vi "Position_TOTAL_R17.vi"() -> (0 "Valid Beacon Sets":bool[](array[boolean])=[TRUE, TRUE, TRUE, TRUE, FALSE], 5 "Distance Between \nCameras  (*unit)":sgl=1.6977187, 12 "dX, dY\nLeft Cam":cluster{"X":sgl[], "Y":sgl[]}={"X"=[-5.750775, -4.1849813, -3.081379, -2.0098581, 0.0], "Y"=[7.9585915, 7.9595685, 7.960258, 7.960927, 0.0]}, 13 "Position Valid":bool=TRUE, 14 "Left Camera Real Coordinates":cluster{"X":sgl, "Y":sgl}={"X"=7.9602513, "Y"=5.592073}, 16 "dX, dY\nRight Cam":cluster{"X":sgl[], "Y":sgl[]}={"X"=[-7.3032045, -5.737411, -4.6338086, -3.5622878, -1.5524296], "Y"=[7.2714148, 7.2723923, 7.2730813, 7.273751, -0.68717635]}, 17 "Distance to Each Beacon":cluster{" Right Cam":sgl[], " Left Cam":sgl[]}={" Right Cam"=[10.303839, 9.074741, 8.6335535, 8.091994, 1.0], " Left Cam"=[9.816596, 8.779684, 8.546625, 8.202919, 1.0]}, 18 "Robot Coordinates":cluster{"X":sgl, "Y":sgl}={"X"=7.616663, "Y"=6.3682876}, 19 "Orietnation\n(current)":sgl=-23.843685 format="%#_13g")   [LabVIEW 2015]
uses:
  <vilib>/Analysis/NI_AALPro.lvlib
  <vilib>/myRIO/Instrument Drivers/Onboard IO/DIO/DIO.lvlib
  <vilib>/Instr/_visa.llb/VISA Configure Serial Port (Instr).vi
  <vilib>/Analysis/coordinate.llb/2D Cartesian Coordinate Rotation (Array).vi
panel:
  out "IMAQ Scale":sgl=54.176815
  out "Current Recovery State -L":enum16{"Generic Sweep", "Recovery Search"}(ring)=enum."Recovery Search"
  out "Current Move Delta - L 2":u16
  out "Next Recovery State - Left":enum16{"Generic Sweep", "Recovery Search"}(ring)=enum."Recovery Search"
  out "Next Recovery State - Right":enum16{"Generic Sweep", "Recovery Search"}(ring)=enum."Recovery Search"
  out "Current Recovery State - Right":enum16{"Generic Sweep", "Recovery Search"}(ring)=enum."Recovery Search"
  in  "Initial Recovery State  - Right":enum16{"Generic Sweep", "Recovery Search"}(ring)=enum."Recovery Search"
  in  "Initial Recovery State - L":enum16{"Generic Sweep", "Recovery Search"}(ring)=enum."Recovery Search"
  out "Next Tracking State - Right":enum16{"Track", "Reactive Predict", ""}(ring)
  out "Current Tracking State - Right 2":enum16{"Track", "Reactive Predict", ""}(ring)
  in  "Initial Tracking State - Right":enum16{"Track", "Reactive Predict", ""}(ring)
  out "Last Track Angle - R":sgl=98.61328
  out "Next Tracking State - Left":enum16{"Track", "Reactive Predict", ""}(ring)
  in  "Initial Tracking State - Left":enum16{"Track", "Reactive Predict", ""}(ring)
  out "Current Tracking State - Left":enum16{"Track", "Reactive Predict", ""}(ring)
  in  "Timeout to \nEnable Reactive Predict":u16=5
  out "Tracking Timeout\nCount - R":i32
  in  "Tracking Timeout\nThreshold":i32=10
  out "Tracking Timeout\nCount - L":i32
  in  "Search Direction - in - Right":bool=TRUE
  out "Next Main State - Right":T1(ring)=enum."Tracking"
  in  "Recovery Search\nDirection - R":bool
  out "Recovery Mode Count in Right":i32
  out "Frames Processed\nCount - in Right":i32
  out "Recovery Search\nmove Count - Right":u16
  out "Recovery Search\nAttempt Count - Right":u16
  in  "Mounting Offset - Right":sgl=45.0
  in  "Tracking Angle - Right":sgl=98.60307
  in  "Current Servo Position\n- Right":u16
  out "New Data  Flag\nRight Servo":bool
  in  "Track Angle Valid  - R":bool=TRUE
  out "Current Main State - Right":T1(ring)=enum."Tracking"
  in  "Initial Main State- Right":T1(ring)
  in  "Recovery Search\nDirection - L 2":bool
  in  "Max Recovery Count\n(Recovery Search) 2":u16
  in  "Max Recovery\nSearch Attempts 2":u16
  in  "Image Lock - Right 2":bool
  out "Last Track Angle - L":sgl=87.24609
  in  "Recovery Search\nDirection - L":bool=TRUE
  out "Next Main State - Left":T1(ring)=enum."Tracking"
  out "Current Move Delta - L":u16
  in  "Max Recovery Count\n(Recovery Search)":u16=10
  in  "Max Recovery\nSearch Attempts":u16=3
  out "Recovery Search\nAttempt Count - in - L":u16
  out "Recovery Search\nmove Count - in - L":u16
  in  "Image Lock - Right":bool=TRUE
  out "Recovery Mode Count - in Left":u16
  in  "Middle Beacon\nCoordinates":cluster{"X":sgl, "Y":sgl}={"X"=0.0, "Y"=2.5}
  in  "Min Num Frames\nper Search":i32=2
  in  "Wait Tick Threshold":i32=10
  out "Frames Processed\nCount - in -L":i32
  in  "Maximum Move \nServo Threshold":i16=300
  in  "Minimum Delta \nServo Threshold":i16=3
  in  "Mounting Offset - Left":sgl=-45.0
  in  "Search Step Size":u16=50
  in  "Search Direction - in - L":bool
  in  "Current Servo Position\n- Left":u16
  in  "Tracking Angle - Left":sgl=87.25689
  out "New Data  Flag\nLeft Servo":bool
  in  "Track Angle Valid - Left":bool=TRUE
  in  "Image Lock - Left":bool=TRUE
  in  "Initial Main State - Left":T1(ring)
  out "Current Main State - Left":T1(ring)=enum."Tracking"
  in  "Position Calc\nTimer":u32=100 caption="Position Calc Timer"
  in  "Fetch Input\n(mSec)":u32=20 caption="Update Camera Input\n(mSec)"
  out "Right Data\nInput Flag\n- Internal":bool=TRUE
  in  "Position Calc\nReady":bool
  out "This Servo \nAngle - Right":sgl=98.90625
  in  "Beacon Angles -R":sgl[](array[numeric])=[111.28093, 105.355774, 98.60307, 92.04714, 103.90625]
  in  "Beacon Angles - L":sgl[](array[numeric])=[101.98467, 94.59042, 87.25689, 80.30646, 91.66016]
  in  "Valid Angles -R":bool[](array[boolean])=[TRUE, TRUE, TRUE, TRUE, FALSE]
  in  "Valid Angles - L":bool[](array[boolean])=[TRUE, TRUE, TRUE, TRUE, FALSE]
  out "Left Data\nInput Flag\n- Internal":bool
  in  "Check Shared Var Timer":u32=50 caption="Main Loop\n Timer (ms)"
  out "Left_Flag 2":bool
  out "Right_Flag 2":bool
  out "Beacons Found\n- Left (Bool Array) 2":bool[](array[boolean])=[TRUE, TRUE, TRUE, TRUE, FALSE]
  out "LEFT Beacon Coord - X px (IN) 2":sgl[](array[numeric])=[76.306, 116.841255, 157.35043, 195.67218, 0.0]
  out "LEFT Beacon Position - Y px (IN) 2":sgl[](array[numeric])=[154.30304, 148.59094, 148.39949, 146.94655, 0.0]
  out "This Servo \nAngle - Left":sgl=86.66016
  in  "Compliance Slope":u8=128
  out "deltaMoveServo\n- R":i16
  out "Move Respond - R":bool
  out "Move Respond - L":bool
  out "Last Position":cluster{"X":sgl, "Y":sgl}={"X"=7.6261, "Y"=6.350474}
  out "Last Orientation":sgl=-23.876373
  in  "Distance\nBetween Beacons \n- Tolerance":sgl=0.35 format="%#_13g"
  in  "Distance\nBetween Beacons":sgl=1.0 format="%#_13g"
  out "atan2(y,x)":sgl=0.35412386
  out "dT":dbl=143.499
  in  "Orientation (-2) \nWeight":sgl=0.083333336 format="%#_13g"
  in  "Orientation (-1) \nWeight":sgl=0.16666667 format="%#_13g"
  in  "New Orientation \nThreshold":sgl=10.0
  out "Position Valid\nHistory":bool[](array[boolean])=[TRUE, FALSE, FALSE, TRUE, TRUE, FALSE, TRUE, TRUE, TRUE, TRUE, TRUE, TRUE, FALSE, TRUE, FALSE]
  out "Orientation\nHistory":sgl[](array[numeric])=[-23.876373, 0.0, 0.0, -23.938759, -24.0458, 0.0, -23.14014, -22.504314, -22.596928, -22.90728, -23.237453, -23.75214, 0.0, -23.808718, 0.0]
  out "Robot Coordinates\nHistory":cluster{sgl, sgl}[](array[cluster])=[{7.6261, 6.350474}, {0.0, 0.0}, {0.0, 0.0}, {7.63815, 6.33973}, {7.6316156, 6.322055}, {0.0, 0.0}, {7.6863523, 6.2558875}, {7.688662, 6.2228284}, {7.6736236, 6.2455945}, {7.6880507, 6.2819676}, {7.6893277, 6.3140097}, {7.668109, 6.3330927}, {0.0, 0.0}, {7.6506357, 6.3142757}, {0.0, 0.0}]
  in  "New Position \nThreshold":sgl=0.2
  in  "position(-2) weight":sgl=0.2 format="%#_13g"
  in  "position(-1) weight":sgl=0.3 format="%#_13g"
  out "Orientation Avgd":sgl=-23.876373
  in  "History Size":u8=15
  in  "Max Y (arena)":sgl=15.0
  in  "Max X (arena)":sgl=35.0
  in  "New Position\nWeight":sgl=0.5 format="%#_13g"
  in  "New Orientation\nWeight":sgl=0.75 format="%#_13g"
  in  "Max Std Dev (3)":sgl=0.2 format="%#_13g"
  in  "Max Std Dev (4)":sgl=0.2 format="%#_13g"
  out "Post Filtering\n- Valid Beacons":bool[](array[boolean])=[FALSE, TRUE, TRUE, TRUE, FALSE]
  in  "New Pos\nThreshold (*unit)\nfilterd UNUSED":sgl=0.2
  out "Robot Coordinates - Avgd":cluster{"X":sgl, "Y":sgl}={"X"=7.6261, "Y"=6.350474}
  out "Real Position in Course 2":cluster{"X":dbl[], "Y":dbl[]}(graph)={"X"=[7.626100046018056], "Y"=[6.35047366782369]}
  out "Position \nLock Status":bool=TRUE
  out "Right Camera Real Coordinate":cluster{"X":sgl, "Y":sgl}={"X"=7.2730746, "Y"=7.1445026}
  out "deltaMoveServo\n- L":i16
  in  "Search Step Size\n(deg)":sgl=15.0 format="%#_13g"
  out "Beacons Found\n- Right (Bool Array)":bool[](array[boolean])=[TRUE, TRUE, TRUE, TRUE, FALSE]
  out "RIGHT Beacon Position - Y px (IN)":sgl[](array[numeric])=[153.02994, 149.48933, 150.4864, 150.33003, 0.0]
  out "RIGHT Beacon Coord - X px (IN)":sgl[](array[numeric])=[91.3685, 123.99656, 161.27843, 197.4523, 0.0]
  in  "Right Servo\nID":string="\u0001"
  in  "Servo Comm\nWait Time - (ms)":i32
  in  "Left Servo\nID":string="\u0000"
  out "dT - Comm Loop":u32=19
  in  "Servo Comm\nLoop Time (ms)":i32=20
  in  "close comms":bool
  in  "Max Read\nTx Attempts":u8=3
  in  "Max Write\nTx Attempts":u8=3
  out "Current R (10bit)":u16=696
  out "Servo Moving - R":bool
  out "Servo Moving - L":bool
  out "Current L (10bit)":u16=347
  in  "SERVO ENABLE":bool=TRUE
  out "Move Servo - L":bool
  out "Move Servo - R":bool
  in  "Servo Goal Position\n - Right":u16=695
  in  "Move Servo\nThreshold (deg)":sgl=2.0 format="%#_13g"
  in  "Servo Algorithm\nCycle Time(ms)":i32=25
  in  "Servo Goal Position\n - Left":u16=349
  in  "Current Angle\n - Left (internal)":sgl=86.66016
  in  "Current Angle\n - Right (internal)":sgl=98.90625
  in  "stop":bool
  in  "Num of Beacons (Total)":i8=5
  out "Angle to Pixel Ratios":T2={"Angle to Pixel\nRatio - Horizontal"=0.18125, "Angle to Pixel\nRatio - Vertical"=0.1875} {"Angle to Pixel\nRatio - Vertical" format="%#_13g"; "Angle to Pixel\nRatio - Horizontal" format="%#_13g"}
  in  "Cam AOV Vertical (deg)":sgl=45.0
  in  "Cam AOV Horizontal (deg)":sgl=58.0
  in  "Image Height (px)":sgl=240.0
  in  "Image Width (px)":sgl=320.0
  out "Beacon Coordinates - Left Image":T3={"Beacon Position - X px"=[76.306, 116.841255, 157.35043, 195.67218, 0.0], "Beacon Position - Y px"=[154.30304, 148.59094, 148.39949, 146.94655, 0.0]}
  out "Beacon Coordinates - Right Image":T3={"Beacon Position - X px"=[91.3685, 123.99656, 161.27843, 197.4523, 0.0], "Beacon Position - Y px"=[153.02994, 149.48933, 150.4864, 150.33003, 0.0]}
  out "Distance to LBF":sgl[](array[numeric])=[0.024284193, 0.015691843, 0.008273765, 0.028971607, 0.03291407]
  out "Local Coordinates - Calculated":cluster{sgl[], sgl[]}(graph)={[-2.0384164, -0.70265853, 0.4090246, 1.3811935, 0.0], [9.602626, 8.751521, 8.536832, 8.085801, 0.0]}
  out "Local Coordinates - Adjusted":cluster{sgl[], sgl[]}(graph)={[-2.0372734, -0.60508364, 0.4043527, 1.3844445, 0.0], [9.605212, 8.972328, 8.526259, 8.093158, 0.0]}
  out "Normalized Beacons\nCoordinates Relative\nto Robot\n- Local":cluster{"X":sgl[], "Y":sgl[]}={"X"=[-2.0372734, -0.60508364, 0.4043527, 1.3844445, 0.0], "Y"=[9.605212, 8.972328, 8.526259, 8.093158, 0.0]}
  out "Local Coordinates - Rotated":cluster{dbl[], dbl[]}(graph)={[1.5524295802029098, -5.750774735805926, -4.1849814062260675, -3.0813788557258652, -2.009858210562305, 0.0], [0.6871763361707266, 7.9585912385832795, 7.959568450875426, 7.960257859242679, 7.960927027680405, 0.0]}
  out "All Object Coordinates \n- Local - Rotated":cluster{"X":sgl[], "Y":sgl[]}={"X"=[1.5524296, -5.750775, -4.1849813, -3.081379, -2.0098581, 0.0], "Y"=[0.68717635, 7.9585915, 7.9595685, 7.960258, 7.960927, 0.0]}
  out "Local Coordinates - Normalized":cluster{sgl[], dbl[]}(graph)={[1.6977187, -2.0372734, -0.60508364, 0.4043527, 1.3844445, 0.0], [0.0, 9.605212211608887, 8.972328186035156, 8.526259422302246, 8.093157768249512, 0.0]}
  in  "Max Std Dev (5)":sgl=0.2 format="%#_13g"
  out "All Object Coordinates \n- Local":cluster{"X":sgl[], "Y":sgl[]}={"X"=[1.6977187, -2.0372734, -0.60508364, 0.4043527, 1.3844445, 0.0], "Y"=[0.0, 9.605212, 8.972328, 8.526259, 8.093158, 0.0]}
  out "LOCAL\nBeacon Coordinates\nRelative to Robot":cluster{"dX_beacon":sgl[], "dY_beacon":sgl[]}={"dX_beacon"=[-2.0384164, -0.70265853, 0.4090246, 1.3811935, 0.0], "dY_beacon"=[9.602626, 8.751521, 8.536832, 8.085801, 0.0]}
  out "dA2":sgl=9.6935425 format="%#_13g"
  out "All Same\nDirection":bool=TRUE
  out "Valid Data\nSets":bool[](array[boolean])=[TRUE, TRUE, TRUE, TRUE, FALSE]
  in  "Distance Threshold\nRef Triangles (*unit)":sgl=30.0
  in  "Real Beacon\n - Coordinates":cluster{"X":dbl[], "Y":dbl[]}={"X"=[0.0, 0.0, 0.0, 0.0, 0.0, 0.0], "Y"=[0.5, 1.5, 2.5, 3.5, 4.5, 0.0]}
  # "POSITION CALCULATION VARIABLES"
  # "OUTPUT VALUES"
  # "CONFIG VALUES"
  # "FILTER CONFIG VALUES"
  # "FEEDBACK INPUT VALUES"
  # "INPUT VALUES"
  # "INTERMEDIATE VALUES"
  # "IMAGE TO ANGLE VARIABLES"
  # "VISION PROCESSEING INPUTS"
  # "Use moving average for previous orientation thresholds"
  # "INPUTS"
  # "CONFIG"
  # "OUTPUT VALUES"
  # "*********************"
  # "unfiltered"
  # "NEW FILTER VALS"
  # "Inter Beacon Distance Filtering"
  # "**Calibrate \"distance between cameras\" to image scale"
  # "SERVO CONTROL VARIABLES"
  # "SERVO CONTROL VARIABLES"
  # "CONFIG"
  # "SHARED VARIABLE INPUTS"
  # "LOCAL VARIABLE INPUTS"
  # "INTERNRAL VARIABLES"
  # "SEARCH ROUTINE VARIABLES"
  # "MISC"
  # "SERVO IDs"
  # "CONTROL DELAYS"
  # "COMM LOOP DELAY"
  # "COMM PROTOCOL"
  # "SETTINGS"
  # "Make function of distance^^"
  # "**** only left side starts search\nat previously known good angle"
  # "LEFT SERVO"
  # "RIGHT SERVO"
  # "Main State Machine"
  # "Recovery State Machine"
  # "Current Track Angle Inputs"
  # "Servo Status Inputs"
  # "Main State Machine Inputs"
  # "Recovery State Machine Inputs"
  # "Current Track Angle Inputs"
  # "Servo Status Inputs"
  # "Recovery State Machine Feedback"
  # "Tracking State Machine Inputs"
  # "Tracking State Machine Inputs"
  # "NOTE: Must be 1 bigger than amount of beacons"
  # "NOTE: Must be 1 bigger than amount of beacons"
types:
  T1 = enum16{"Start Up Search", "Tracking", "Recovery Mode", ""}
  T2 = cluster{"Angle to Pixel\nRatio - Horizontal":sgl, "Angle to Pixel\nRatio - Vertical":sgl}
  T3 = cluster{"Beacon Position - X px":sgl[], "Beacon Position - Y px":sgl[]}
  T4 = cluster{"Array of Double":dbl[], "Array of Double":dbl[]}
  T5 = typedef "DIO.lvlib/DIO Reference.ctl" = cluster{"myRIO Reference":T6, "DIO Channels List":T10}
  T6 = typedef "myRIO Generic Hardware Reference.ctl" = cluster{"myRIO Model":T7, "myRIO Hardware Reference":T8}
  T7 = typedef "Hardware Version Enum.ctl" = enum16{"Unknown", "myRIO-1900", "myRIO-1950", "roboRIO"}
  T8 = typedef "myRIO v1.0 Reference.ctl" = cluster{"Generic FPGA Reference":T9, "Allow multiple opens":bool}
  T9 = typedef "Generic FPGA Reference.ctl" = refnum<k20>
  T10 = typedef "DIO Channels List.ctl" = T11[]
  T11 = typedef "DIO Channels Enum.ctl" = enum16{"Not Connected", "C/DIO0", "C/DIO1", "C/DIO2", "C/DIO3", "C/DIO4", "C/DIO5", "C/DIO6", "C/DIO7", "A/DIO0", "A/DIO1", "A/DIO2", "A/DIO3", "A/DIO4", "A/DIO5", "A/DIO6", "A/DIO7", "A/DIO8", "A/DIO9", "A/DIO10", "A/DIO11", "A/DIO12", "A/DIO13", "A/DIO14", "A/DIO15", "B/DIO0", "B/DIO1", "B/DIO2", "B/DIO3", "B/DIO4", "B/DIO5", "B/DIO6", "B/DIO7", "B/DIO8", "B/DIO9", "B/DIO10", "B/DIO11", "B/DIO12", "B/DIO13", "B/DIO14", "B/DIO15", "LED0", "LED1", "LED2", "LED3", "Button0", "DIO/DIO0", "DIO/DIO1", "DIO/DIO2", "DIO/DIO3", "DIO/DIO4", "DIO/DIO5", "DIO/DIO6", "DIO/DIO7", "DIO/DIO8", "DIO/DIO9", "SPI/CS0", "SPI/CS1", "SPI/CS2", "SPI/CS3", "LED RADIO (Green)", "LED RADIO (Red)", "LED COMM (Green)", "LED COMM (Red)", "LED MODE (Green)", "LED MODE (Red)"}
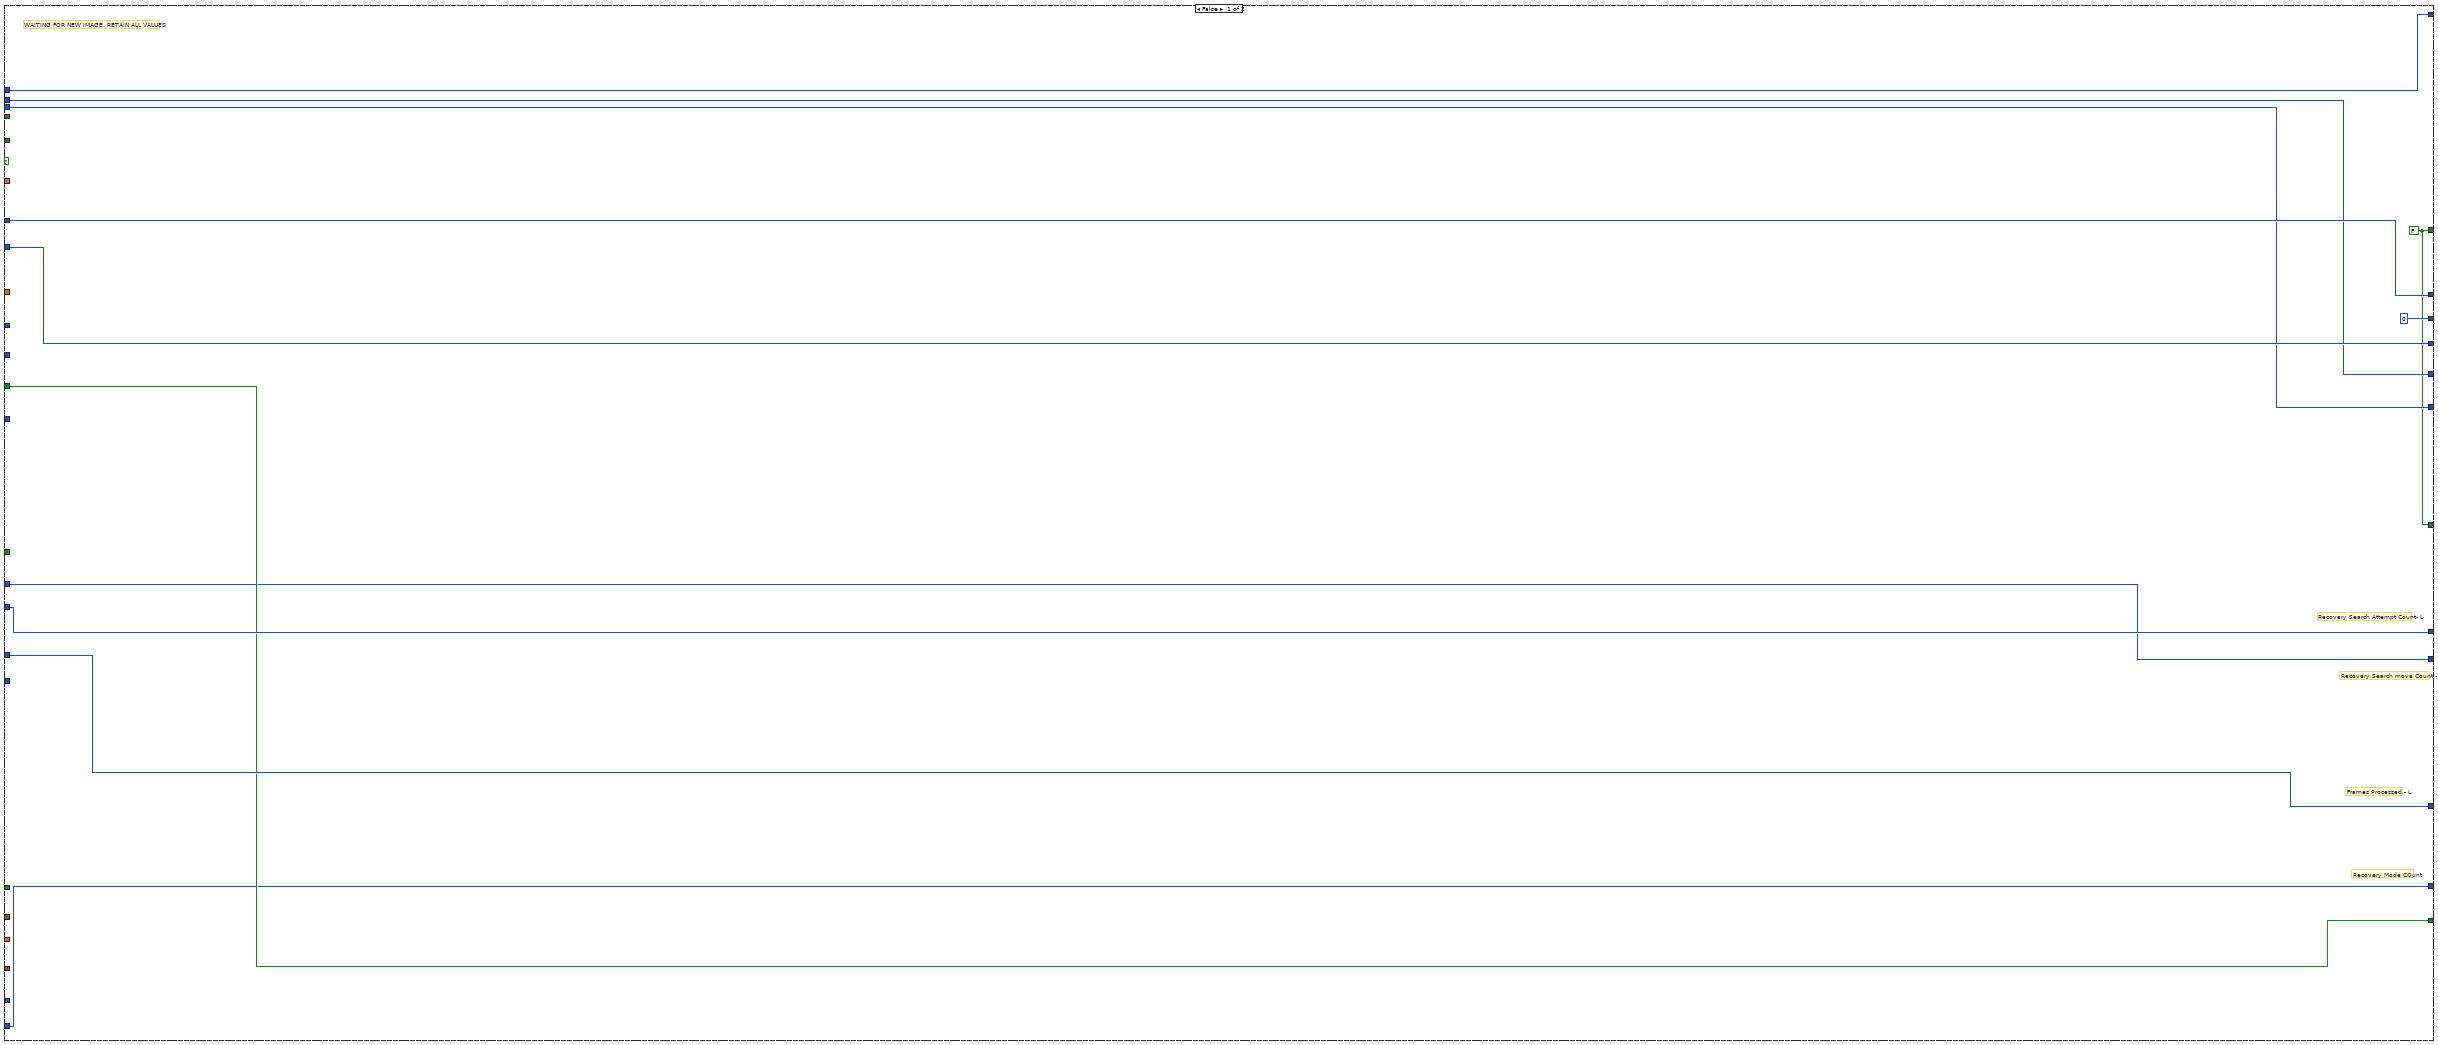
[diagram p2: hidden frame]
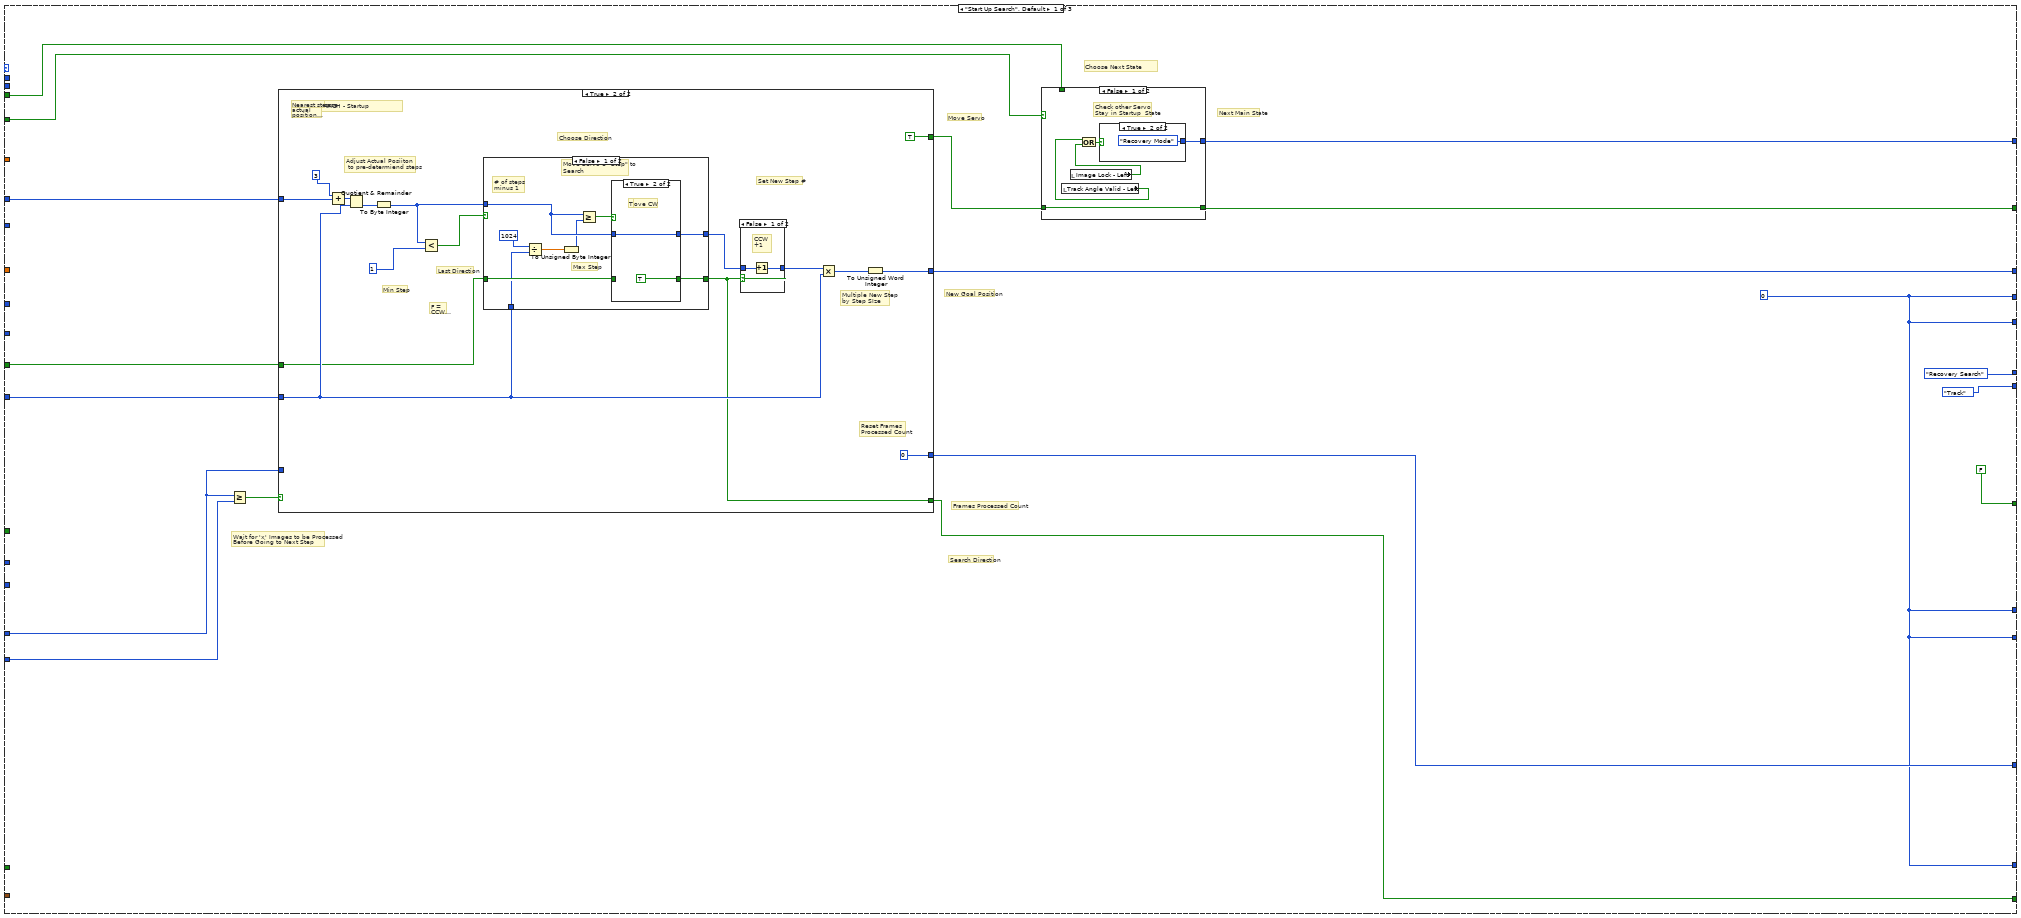
[diagram p3: hidden frame]
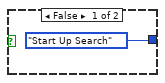
[diagram p4: hidden frame]
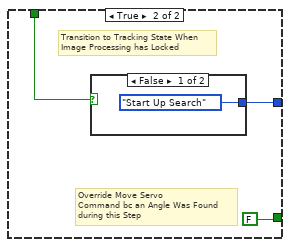
[diagram p5: hidden frame]
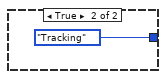
[diagram p6: hidden frame]
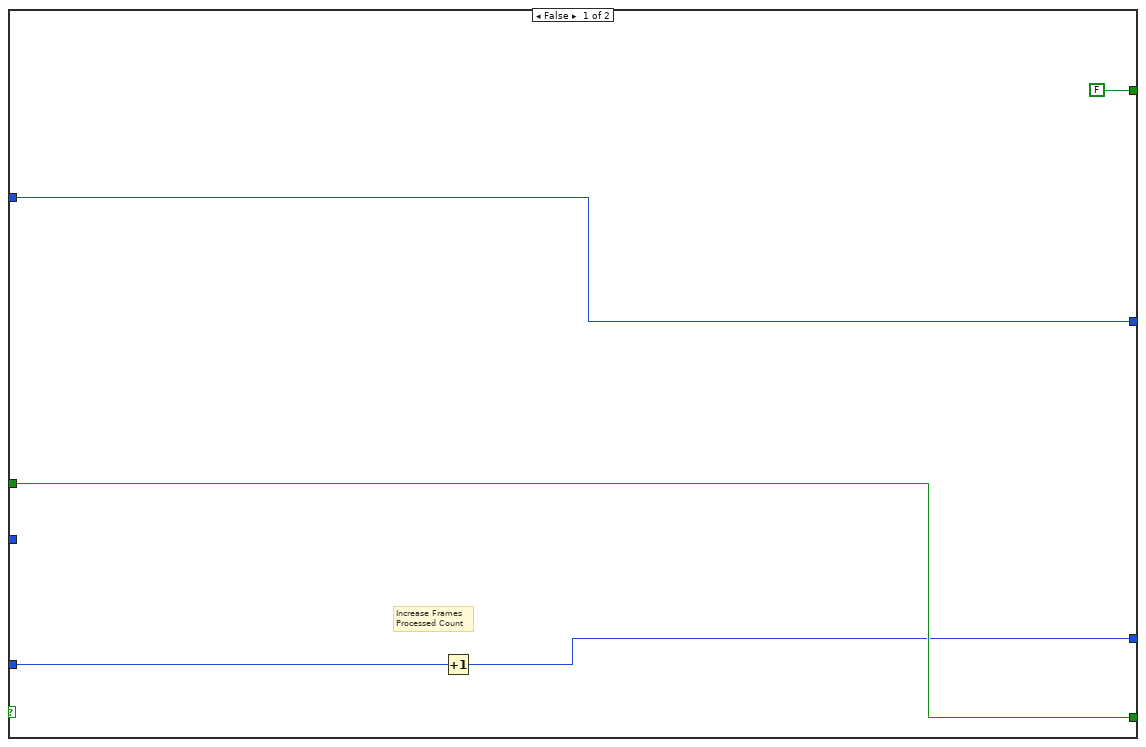
[diagram p7: hidden frame]
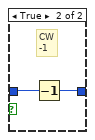
[diagram p8: hidden frame]
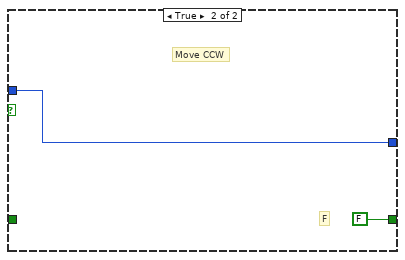
[diagram p10: hidden frame]
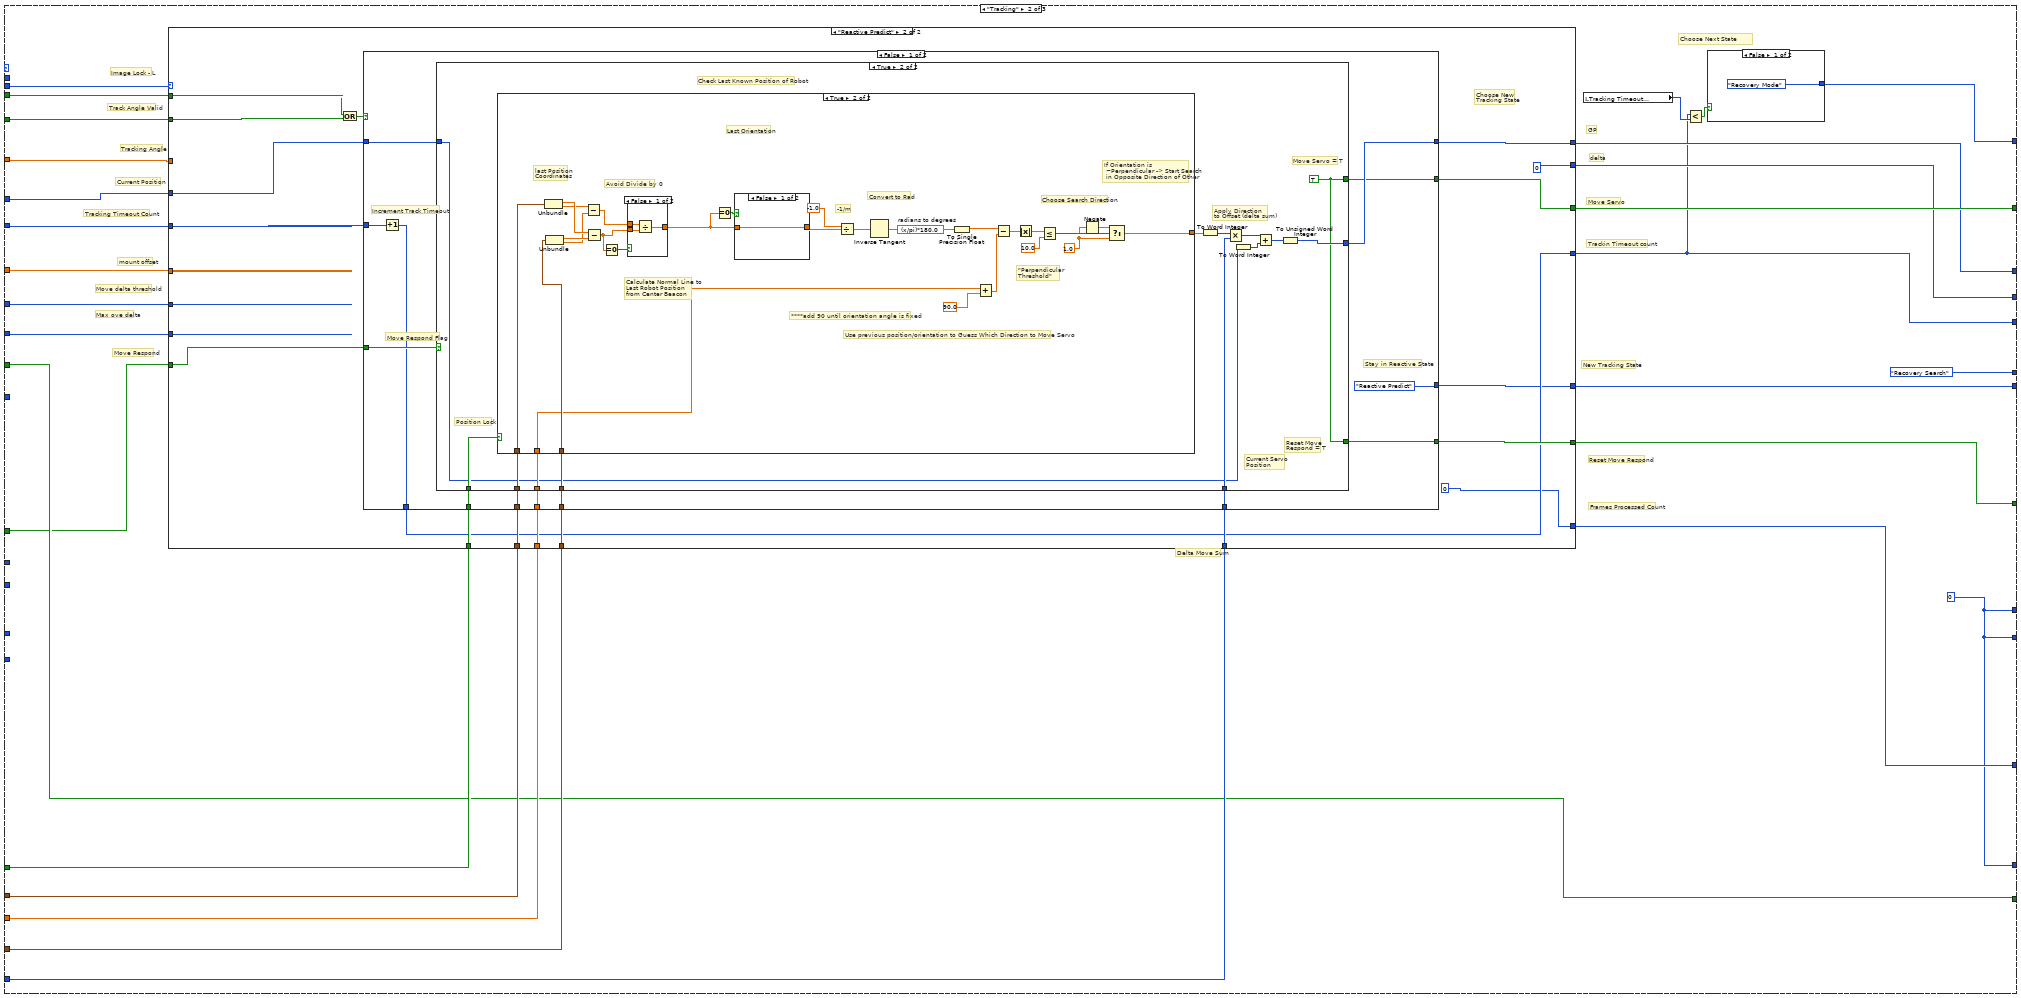
[diagram p11: hidden frame]
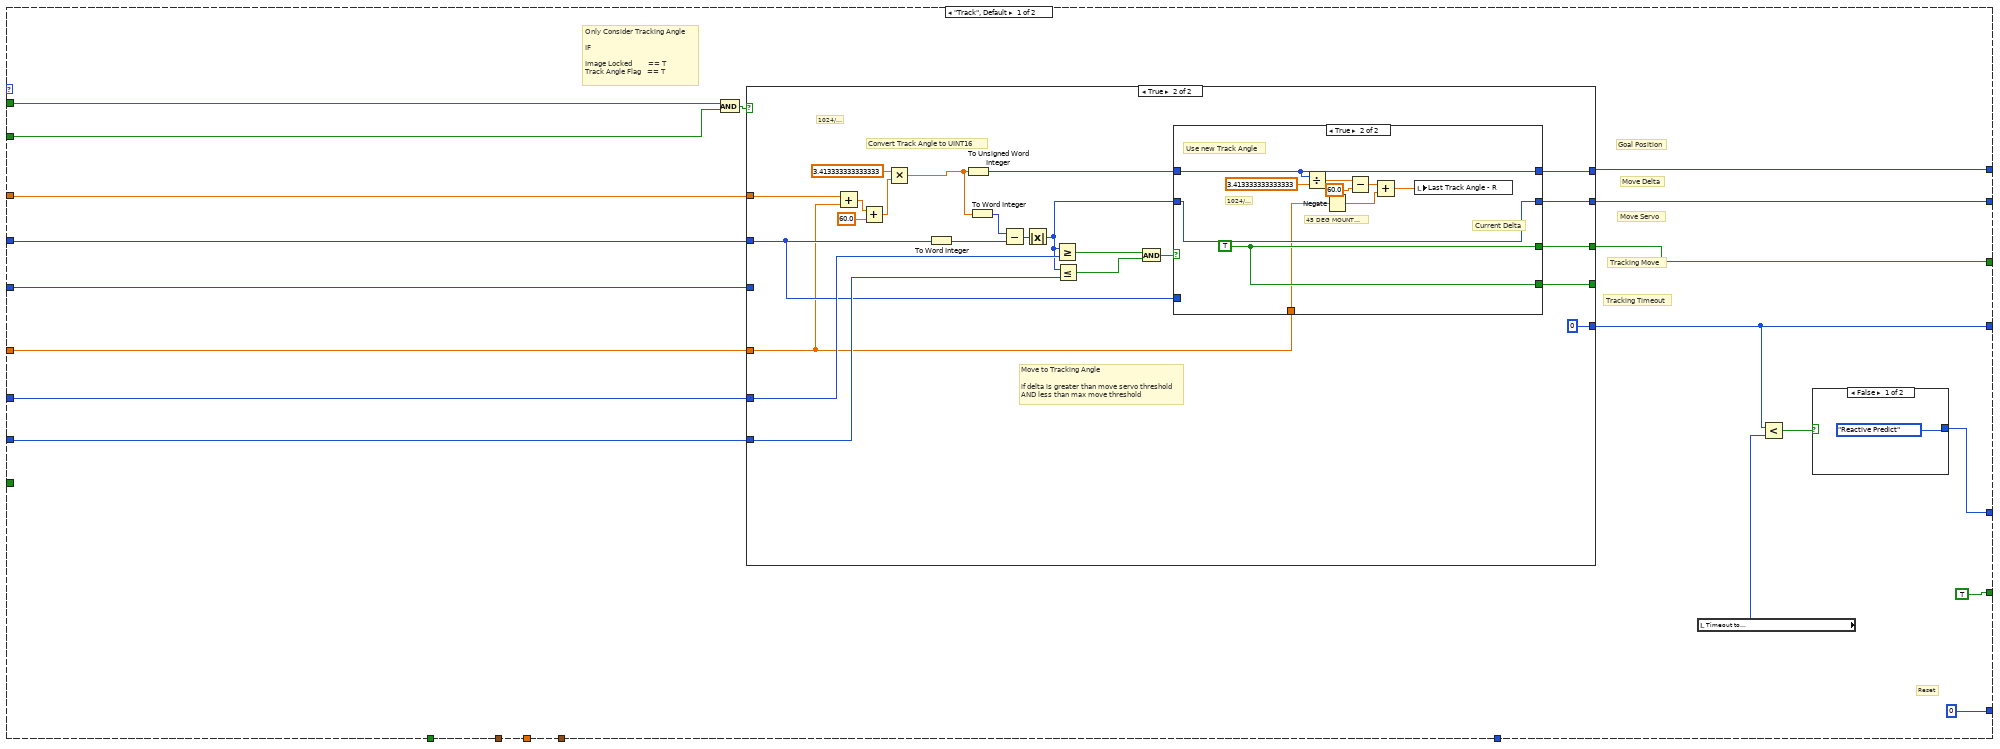
[diagram p12: hidden frame]
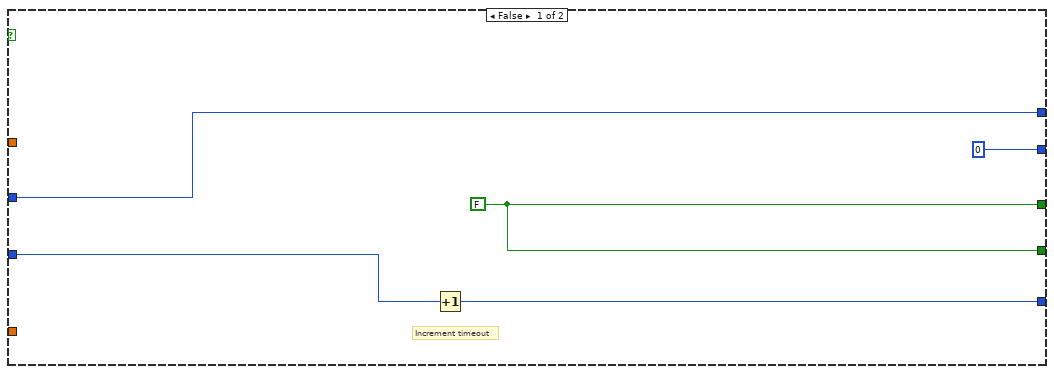
[diagram p13: hidden frame]
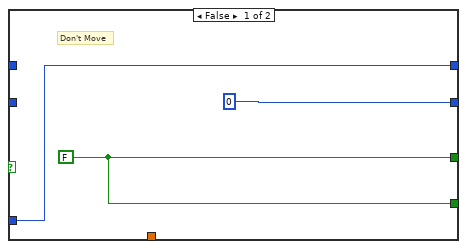
[diagram p14: hidden frame]
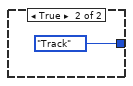
[diagram p15: hidden frame]
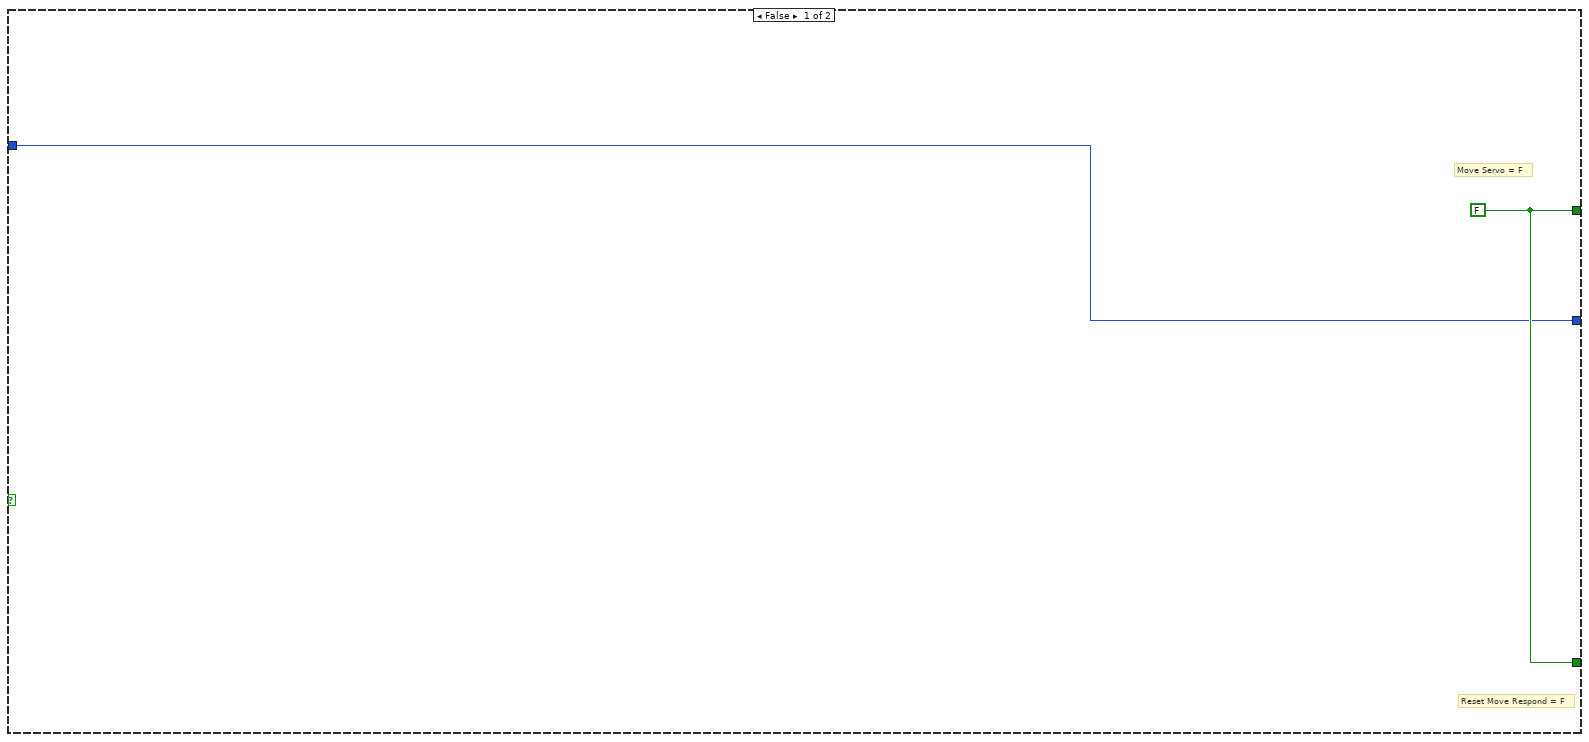
[diagram p16: hidden frame]
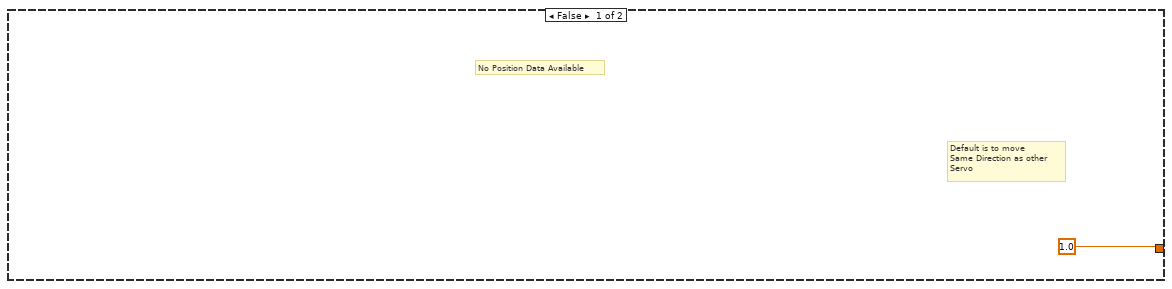
[diagram p17: hidden frame]
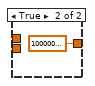
[diagram p18: hidden frame]
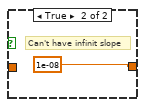
[diagram p19: hidden frame]
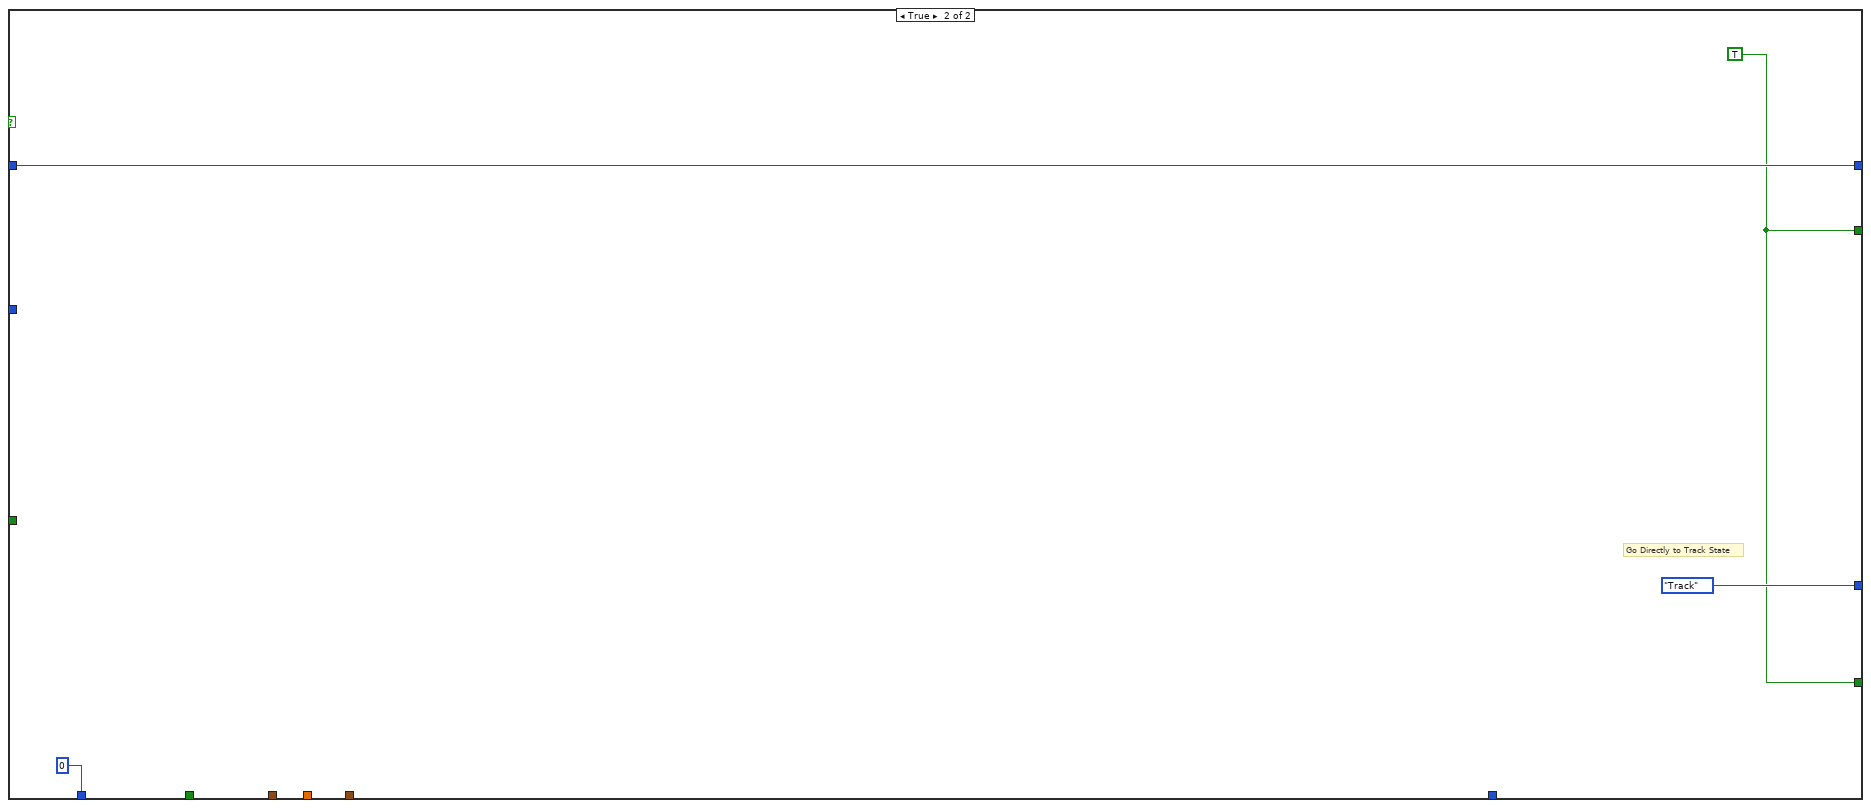
[diagram p20: hidden frame]
diagram:
  (unwired) enum16{"Generic Sweep", "Recovery Search"}."Recovery Search"
  w11 = 0 ("Frames Processed\nCount - in")
  w12 = 0 ("Frames Processed\nCount - in")
  w1 = FALSE
  w34 = sgl 0.0
  # "SERVO CONTROL FLAGS"
  # "***"
  # "Next Tracking State"
  # "Tracking Timeout Count"
  # "Search Direction - L"
  # "Next Recovery State"
  # "Move Respond"
  # "Recovery Mode Count - L"
  # "Delta Move Sum - L"
  # "Wait Tick Count - L"
  # "Frames Processed - L"
  # "Recovery Search move Count - L"
  # "Recovery Search Attempt Count- L"
  # "Next Main State"
  # "Search Direction - L"
  # "Next Recovery State"
  # "INPUTS - Local vars"
  # "Recovery Mode Count - L"
  # "Delta Move Sum - L"
  # "Frames Processed\nLeft"
  # "Move Respond - R"
  # "Initial Search Direction\n- Right"
  # "Move Respond"
  # "Recovery Mode Count - L"
  # "Delta Move Sum - L"
  # "Wait Tick Count - L"
  # "Frames Processed - L"
  # "Recovery Search move Count - L"
  # "Recovery Search Attempt Count- L"
  # "Next Main State"
  # "Settings -- Update in a slow loop"
  # "Recovery Mode Count - L"
  # "Delta Move Sum - L"
  # "Frames Processed\nLeft"
  # "Move Respond - L"
  # "Replace these with\nconstants"
  # "Initial Search Direction\n- Left"
  # "Read Inputs when Available"
  # "# of Physical Beacons"
  # "Right Data Internal Falg"
  # "Left Data Internal Falg"
  # "Initialize Shift Arrays"
  # "Robot Position (cluster)\nShift Array"
  # "Robot Position (cluster)\nShift Array"
  # "Position Valid Shift Array"
  # "Orientation Shift Array"
  # "Position Valid Shift Array"
  # "Orientation Shift Array"
  # "Servo Communication (to Servo- UART))"
  # "Internal Local Variables"
  # "Servo Control Logic"
  # "Local Variables"
  # "Images to Robot Position Calculation Process"
  # "SERVO MOTOR CONTROL"
  # "SERVO MOTOR CONTROL"
  n1 = Divide(x="Cam AOV Horizontal (deg)", y="Image Width (px)") -> (x/y=w25:sgl)
  n2 = Divide(x="Cam AOV Vertical (deg)", y="Image Height (px)") -> (x/y=w26:sgl)
  n3 = Bundle(w25, w26) -> (w20:cluster{sgl, sgl})  [unwired: 1 in]
  "Angle to Pixel Ratios" <- w20
  n4 = disable-structure shown="Disabled" {
    frame Disabled {
      # "Always Read Incoming Flags & Store"
      n5 = while {
        tunnel: "Check Shared Var Timer" -> [w46]
        stop <- FALSE stop-if-true
        n6 = shared-variable "myRIO-1900\\Lib1.lvlib\\RIGHT_FLAG"() -> (→"Right_Flag 2":bool)  [unwired: 1 in, 1 out]
        n7 = shared-variable "myRIO-1900\\Lib1.lvlib\\Left_Flag"() -> (→"Left_Flag 2":bool)  [unwired: 1 in, 1 out]
        n8 = call "Wait8"("Count(mSec)"=w46) -> ()  [unwired: 1 out]
      }
    }
    frame Enabled {
    }
  }
  n9 = while {
    shift-right: [w55] -> _
    shift-left: w1 -> [w60]
    shift-right: [w54] -> _
    shift-left: w1 -> [w58]
    tunnel: w20 -> [w56]
    tunnel: "Num of Beacons (Total)" -> [w57]
    stop <- FALSE stop-if-true
    # "Wait for Both Internal Flags"
    n10 = call "Wait6"("Count(mSec)"="Fetch Input\n(mSec)") -> ()  [unwired: 1 out]
    n11 = shared-variable "RT myRIO Target - Overlord\\Localization_Variables_r0.lvlib\\RIGHT_FLAG"() -> (w51:bool)  [unwired: 1 in, 1 out]
    n12 = shared-variable "RT myRIO Target - Overlord\\Localization_Variables_r0.lvlib\\Left_Flag"() -> (w52:bool)  [unwired: 1 in, 1 out]
    n13 = case shown="True" w51 {
      tunnel: w57 -> [_ w75]
      tunnel: w56 -> [_ w73]
      tunnel: [w61 w62] -> w49
      tunnel: w58 -> [w61 _]
      frame False {
        # "Don't Update Servo Position\nbc we're waiting on new Data to\ncome in and the servo position\nwas set at the previous set of data"
      }
      frame True {
        w62 = TRUE
        # "Store Values"
        # "Raise Internal Flag"
        # "If New Data Available"
        # "From Shift Reg"
        # "Perforrm Indivudual Angle Calculation"
        # "Pull Down Individual Flag"
        n14 = shared-variable "RT myRIO Target - Overlord\\Localization_Variables_r0.lvlib\\RIGHT_BEACON_X_array"() -> (w68:dbl[])  [unwired: 1 in, 1 out]
        "RIGHT Beacon Coord - X px (IN)" <- w68
        n15 = shared-variable "RT myRIO Target - Overlord\\Localization_Variables_r0.lvlib\\Image Lock - R"() -> (w63:bool)  [unwired: 1 in, 1 out]
        n16 = shared-variable "RT myRIO Target - Overlord\\Localization_Variables_r0.lvlib\\RIGHT_BEACON_Y_array"() -> (w67:dbl[])  [unwired: 1 in, 1 out]
        "RIGHT Beacon Position - Y px (IN)" <- w67
        n17 = shared-variable "RT myRIO Target - Overlord\\Localization_Variables_r0.lvlib\\RIGHT_BEACON_BOOL_array"() -> (w66:bool[])  [unwired: 1 in, 1 out]
        "Beacons Found\n- Right (Bool Array)" <- w66
        n18 = local write "Image Lock - Right"(w63) -> ()
        n19 = Bundle("Array of Double"=w68, "Array of Double"=w67) -> (w65:T4)  [unwired: 1 in]
        "Beacon Coordinates - Right Image" <- w65
        n20 = shared-variable "RT myRIO Target - Overlord\\Localization_Variables_r0.lvlib\\Right Servo Angle_Image"() -> (w64:dbl)  [unwired: 1 in, 1 out]
        "This Servo \nAngle - Right" <- w64
        n21 = shared-variable "RT myRIO Target - Overlord\\Localization_Variables_r0.lvlib\\RIGHT_FLAG"(FALSE) -> ()  [unwired: 1 in, 1 out]
        n22 = feedback #1() -> (w77:sgl[])  [unwired: 1 in]
        n23 = feedback #2() -> (w76:bool[])  [unwired: 1 in]
        n24 = call "Angle Calc_Individual Process R2.vi"("Angle to Pixel Ratios"=w73, "Previous Angles"=w77, "Num of Beacons"=w75, "Beacon Coordinates - Image"=w65, "Current Servo Angle"=w64, "Beacons Found (Bool Array)"=w66, "Previous Valid Angles"=w76) -> ("Servo Goal Angle"=w72:dbl, "Valid Beacons (Bool Array)\nPosition Calc"=w70:bool[], "Angle Of Beacons \nRelative to Robot"=w69:sgl[], "Angles Valid\nServo Control"=w71:bool)  [unwired: 2 in, 3 out]
        n25 = feedback-in #1(w69) -> ()
        n26 = feedback-in #2(w70) -> ()
        n27 = local write "Track Angle Valid  - R"(w71) -> ()
        n28 = local write "Beacon Angles -R"(w69) -> ()
        n29 = local write "Valid Angles -R"(w70) -> ()
        n30 = local write "Tracking Angle - Right"(w72) -> ()
        n31 = local write "New Data  Flag\nRight Servo"(w62) -> ()
      }
    }
    "Right Data\nInput Flag\n- Internal" <- w49
    n32 = case shown="False" w52 {
      tunnel: [w78 w79] -> w48
      tunnel: w60 -> [w78 _]
      tunnel: w56 -> [_ w83]
      tunnel: w57 -> [_ w82]
      frame False {
        # "Don't Update Servo Position\nbc we're waiting on new Data to\ncome in and the servo position\nwas set at the previous set of data"
      }
      frame True {
        w79 = TRUE
        # "Store Values"
        # "Raise Internal Flag"
        # "If New Data Available"
        # "Perforrm Indivudual Angle Calculation"
        # "Pull Down Individual Flag"
        n33 = shared-variable "RT myRIO Target - Overlord\\Localization_Variables_r0.lvlib\\LEFT_BEACON_X_array"() -> (w90:dbl[])  [unwired: 1 in, 1 out]
        "LEFT Beacon Coord - X px (IN) 2" <- w90
        n34 = shared-variable "RT myRIO Target - Overlord\\Localization_Variables_r0.lvlib\\LEFT_BEACON_Y_array"() -> (w91:dbl[])  [unwired: 1 in, 1 out]
        "LEFT Beacon Position - Y px (IN) 2" <- w91
        n35 = shared-variable "RT myRIO Target - Overlord\\Localization_Variables_r0.lvlib\\LEFT_BEACON_BOOL_array"() -> (w92:bool[])  [unwired: 1 in, 1 out]
        "Beacons Found\n- Left (Bool Array) 2" <- w92
        n36 = shared-variable "RT myRIO Target - Overlord\\Localization_Variables_r0.lvlib\\Image Lock - L"() -> (w80:bool)  [unwired: 1 in, 1 out]
        n37 = local write "Image Lock - Left"(w80) -> ()
        n38 = Bundle("Array of Double"=w90, "Array of Double"=w91) -> (w88:T4)  [unwired: 1 in]
        "Beacon Coordinates - Left Image" <- w88
        n39 = shared-variable "RT myRIO Target - Overlord\\Localization_Variables_r0.lvlib\\Left Servo Angle_Image"() -> (w81:dbl)  [unwired: 1 in, 1 out]
        "This Servo \nAngle - Left" <- w81
        n40 = shared-variable "RT myRIO Target - Overlord\\Localization_Variables_r0.lvlib\\Left_Flag"(FALSE) -> ()  [unwired: 1 in, 1 out]
        n41 = feedback #3() -> (w94:sgl[])  [unwired: 1 in]
        n42 = feedback #4() -> (w93:bool[])  [unwired: 1 in]
        n43 = call "Angle Calc_Individual Process R2.vi"("Angle to Pixel Ratios"=w83, "Previous Angles"=w94, "Num of Beacons"=w82, "Beacon Coordinates - Image"=w88, "Current Servo Angle"=w81, "Beacons Found (Bool Array)"=w92, "Previous Valid Angles"=w93) -> ("Servo Goal Angle"=w87:dbl, "Valid Beacons (Bool Array)\nPosition Calc"=w85:bool[], "Angle Of Beacons \nRelative to Robot"=w84:sgl[], "Angles Valid\nServo Control"=w86:bool)  [unwired: 2 in, 3 out]
        n44 = feedback-in #3(w84) -> ()
        n45 = feedback-in #4(w85) -> ()
        n46 = local write "Track Angle Valid - Left"(w86) -> ()
        n47 = local write "Beacon Angles - L"(w84) -> ()
        n48 = local write "Valid Angles - L"(w85) -> ()
        n49 = local write "Tracking Angle - Left"(w87) -> ()
        n50 = local write "New Data  Flag\nLeft Servo"(w79) -> ()
      }
    }
    "Left Data\nInput Flag\n- Internal" <- w48
    n51 = And(x=w48, y=w49) -> (x .and. y?=w59:bool)
    n52 = case shown="True" w59 {
      selector: w59 -> [_ w97]
      tunnel: w48 -> [w96 _]
      tunnel: [w96 w98] -> w55
      tunnel: [w95 w98] -> w54
      tunnel: w49 -> [w95 _]
      frame False {
      }
      frame True {
        w98 = FALSE
        # "Reset Internal Data Flags"
        # "Position Data\nReady Enabled"
        n53 = local write "Position Calc\nReady"(w97) -> ()
      }
    }
  }
  n54 = Bundle(w34, w34) -> (w37:cluster{sgl, sgl})  [unwired: 1 in]
  n55 = Initialize Array(w34, "History Size") -> (w32:sgl[])
  n56 = Initialize Array(w37, "History Size") -> (w33:cluster{sgl, sgl}[])
  n57 = Initialize Array(FALSE, "History Size") -> (w31:bool[])
  n58 = call "Tick Count4"() -> ("Tick Count(uSec)"=w30:u32)
  n59 = while {
    shift-right: [w109] -> _
    shift-left: w32 -> [w106]
    shift-right: [w108] -> _
    shift-left: w31 -> [w107]
    shift-right: [w110] -> _
    shift-left: w33 -> [w101]
    shift-right: [w102] -> _
    shift-left: w30 -> [w103]
    stop <- "stop" stop-if-true
    n60 = call "Wait5"("Count(mSec)"="Position Calc\nTimer") -> ()  [unwired: 1 out]
    n61 = case shown="True" "Position Calc\nReady" {
      selector: "Position Calc\nReady" -> [_ w124]
      tunnel: w101 -> [_ w159]
      tunnel: w101 -> [w119 w149]
      tunnel: w106 -> [w121 w148]
      tunnel: w107 -> [w120 w147]
      tunnel: [w121 w146] -> w109
      tunnel: [w120 w141] -> w108
      tunnel: [w119 w145] -> w110
      tunnel: w107 -> [_ w144]
      tunnel: w106 -> [_ w143]
      tunnel: [w118 w136] -> w104
      tunnel: w103 -> [_ w136]
      tunnel: [FALSE TRUE] -> w105
      tunnel: w101 -> [_ w131]
      frame False {
        n62 = call "Tick Count5"() -> ("Tick Count(uSec)"=w118:u32)
      }
      frame True {
        # "Update Outputs\nif Current Calc is Invalid\n(shouldn't matter)"
        # "Estimate Orienation Based on Previous Position"
        # "****# of previous in history that must be true\nin order for position to be considered \"locked\""
        # "New Position is Valid if both \nOrientation and Positions\nis within range of previous"
        # "Robot Position\n Shift Array"
        # "Position Valid Shift Array"
        # "Orientation Shift Array"
        # "Orientation Value"
        # "Shift & Insert Current Position Valid"
        # "Position Valid\n(orientation)"
        # "Position Valid\n(position)"
        # "Update Shift Registers"
        # "Shift & Insert Current Calculated Orientation"
        # "Shift & Insert Current Robot Position"
        # "UPDATE FINAL OUTPUT\n VALUES"
        # "Find Common Beacons\nAmong Cameras"
        # "Valid Beacon Sets"
        # "Currently will only\ncalculate position if 2+ \nbeacons are available \nfrom both cameras"
        n63 = Not(x=w124) -> (.not. x?=w125:bool)
        n64 = local write "Position Calc\nReady"(w125) -> ()
        n65 = disable-structure shown="Disabled" {
          disable-tunnel: "Valid Angles - L" -> [w225 _]
          disable-tunnel: "Valid Angles -R" -> [w224 _]
          frame Disabled {
            # "Each has at \nleast 1 beacon"
            n66 = Boolean Array To Number(Boolean array=w224) -> (number=w226:u32)
            n67 = Boolean Array To Number(Boolean array=w225) -> (number=w227:u32)
            n68 = Greater Than 0?(x=w226) -> (x > 0?=w228:bool)
            n69 = Greater Than 0?(x=w227) -> (x > 0?=w229:bool)
            n70 = And(x=w229, y=w228) -> ()  [unwired: 1 out]
          }
          frame Enabled {
          }
        }
        n71 = And(x="Valid Angles - L", y="Valid Angles -R") -> (x .and. y?=w160:bool[])
        "Valid Beacon Sets" <- w160
        n72 = local read "Num of Beacons (Total)"() -> (w126:i8)
        n73 = Boolean To (0,1)(Boolean=w160) -> (0, 1=w164:i16[])
        n74 = Add Array Elements(numeric array=w164) -> (sum=w163:i16)
        n75 = Greater?(x=w163, y=1) -> (0:w161:bool)
        n76 = case shown="True" w161 {
          tunnel: w160 -> [_ w252]
          tunnel: "Beacon Angles - L" -> [_ w250]
          tunnel: "Beacon Angles -R" -> [_ w249]
          tunnel: w126 -> [_ w251]
          tunnel: w160 -> [_ w248]
          tunnel: w159 -> [_ w247]
          tunnel: [w231 w246] -> w151
          tunnel: [w232 w245] -> w134
          tunnel: [w232 w244] -> w133
          tunnel: [w230 w243] -> w152
          tunnel: w144 -> [_ w242]
          tunnel: w143 -> [_ w241]
          tunnel: w131 -> [_ w240]
          frame False {
            w230 = sgl 0.0 ("f")
            w232 = FALSE
            # "FALSE"
            # "F"
            n77 = Bundle("f"=w230, "f"=w230) -> (w231:cluster{"f":sgl, "f":sgl})  [unwired: 1 in]
          }
          frame True {
            # "Number of Beacons"
            # "**maybe add case\nto handle if some arent\nsame direction"
            # "Check 1st element\nwith rest of elements"
            # "Find delta X and delta Y\nto Each Camera from Each Beacon"
            # "Make Sure all Pointed \nIn Same Direction"
            # "For Each Valid Beacon\nCalculate Distance from Each Camera to Each Beacon"
            n78 = shared-variable "RT myRIO Target - Overlord\\Localization_Variables_r0.lvlib\\Scale - Right"() -> (w236:sgl)  [unwired: 1 in, 1 out]
            n79 = shared-variable "RT myRIO Target - Overlord\\Localization_Variables_r0.lvlib\\Scale - Left"() -> (w237:sgl)  [unwired: 1 in, 1 out]
            n80 = Add(x=w237, y=w236) -> (x+y=w235:sgl)
            n81 = Divide(x=w235, y=sgl 2.0) -> (x/y=w233:sgl)
            "IMAQ Scale" <- w233
            n82 = call "Scaling and Mapping"("Signals"=w233) -> ("Scaled Signals"=w239:dynamicdata)  [unwired: 9 in, 1 out]
            n83 = To Single Precision Float(number=w239) -> (single precision float=w238:sgl)
            "Distance Between \nCameras  (*unit)" <- w238
            n84 = for {
              N: w251 -> [_]
              tunnel: w252 -> [w726] mode=indexing
              tunnel: w250 -> [w725] mode=indexing
              tunnel: w249 -> [w724] mode=indexing
              tunnel: w238 -> [w723]
              tunnel: "Distance Threshold\nRef Triangles (*unit)" -> [w722]
              tunnel: [w721] -> w257 mode=indexing
              tunnel: [w720] -> _ mode=indexing
              tunnel: [w719] -> w258 mode=indexing
              tunnel: [w718] -> w254 mode=indexing
              tunnel: [w717] -> w253 mode=indexing
              tunnel: [w716] -> w259 mode=indexing
              n85 = case shown="True" w726 {
                tunnel: w725 -> [w731 w741]
                tunnel: w724 -> [w730 w740]
                tunnel: w723 -> [_ w732]
                tunnel: w722 -> [_ w733]
                tunnel: [w731 w739] -> w721
                tunnel: [w730 w738] -> w720
                tunnel: [FALSE w737] -> w719
                tunnel: [w728 w736] -> w718
                tunnel: [w728 w735] -> w717
                tunnel: [0 w734] -> w716
                frame False {
                  w728 = sgl 1.0
                }
                frame True {
                  # "Build Reference Triangle"
                  n86 = call "Position Calc_Build Reference Triangle_R1.vi"("A2_in"=w741, "A3_in"=w740, "S1 (Length Between\n Cameras - inches)"=w732, "Distance\nThreshold"=w733) -> ("S2"=w736:sgl, "S3"=w735:sgl, "Direction"=w734:i8, "A2"=w739:sgl, "A3"=w738:sgl, "Accept"=w737:bool)  [unwired: 6 in]
                }
              }
            }
            "Valid Data\nSets" <- w258
            n87 = Bundle(w254, w253) -> (→"Distance to Each Beacon":cluster{sgl[], sgl[]})  [unwired: 1 in]
            n88 = Boolean To (0,1)(Boolean=w258) -> (0, 1=w267:i16[])
            n89 = for {
              N: w251 -> [_]
              tunnel: w258 -> [w269] mode=indexing
              tunnel: w259 -> [w270] mode=indexing
              tunnel: [w270] -> w264 mode=indexing if=w269
              # "Only add to array\nif valid distance"
            }
            n90 = Add Array Elements(numeric array=w267) -> (sum=w255:i16)
            n91 = Greater?(x=w255, y=1) -> (0:w261:bool)
            n92 = Index Array(array=w264, index=0) -> (element=w263:i32)
            n93 = Equal?(x=w264, y=w263) -> (x = y?=w262:bool[])
            n94 = And Array Elements(Boolean array=w262) -> (logical AND=w260:bool)
            "All Same\nDirection" <- w260
            n95 = case shown="True" w260 {
              tunnel: w251 -> [_ w291]
              tunnel: w258 -> [_ w295]
              tunnel: w261 -> [_ w294]
              tunnel: w253 -> [_ w292]
              tunnel: w254 -> [_ _]
              tunnel: w257 -> [_ w293]
              tunnel: w255 -> [_ w290]
              tunnel: w254 -> [_ w289]
              tunnel: w253 -> [_ w288]
              tunnel: w250 -> [_ w287]
              tunnel: w249 -> [_ w286]
              tunnel: w248 -> [_ w285]
              tunnel: w238 -> [_ w284]
              tunnel: w247 -> [_ w283]
              tunnel: [w272 w282] -> w246
              tunnel: [w273 w281] -> w245
              tunnel: [w273 w280] -> w244
              tunnel: [w271 w279] -> w243
              tunnel: w242 -> [_ w278]
              tunnel: w241 -> [_ w277]
              tunnel: w240 -> [_ w276]
              frame False {
                w271 = sgl 0.0 ("f")
                w273 = FALSE
                w274 = 0
                w275 = sgl 0.0
                (unwired) FALSE
                # "FALSE"
                n96 = Build Array(w275, w275, w275) -> ()  [unwired: 1 out]
                n97 = Build Array(w275, w275, w275) -> ()  [unwired: 1 out]
                n98 = Build Array(w275, w275, w275) -> ()  [unwired: 1 out]
                n99 = Build Array(w275, w275, w275) -> ()  [unwired: 1 out]
                n100 = Build Array(w275, w275, w275) -> ()  [unwired: 1 out]
                n101 = Build Array(w275, w275, w275) -> ()  [unwired: 1 out]
                n102 = Build Array(w274, w274, w274) -> ()  [unwired: 1 out]
                n103 = Bundle("f"=w271, "f"=w271) -> (w272:cluster{"f":sgl, "f":sgl})  [unwired: 1 in]
              }
              frame True {
                # "All Values in Same Direction"
                n104 = case shown="True" w294 {
                  tunnel: w291 -> [_ w313]
                  tunnel: w295 -> [_ w383]
                  tunnel: w293 -> [_ w382]
                  tunnel: w292 -> [_ w381]
                  tunnel: w290 -> [_ _]
                  tunnel: w289 -> [_ _]
                  tunnel: w288 -> [_ _]
                  tunnel: w287 -> [_ _]
                  tunnel: w286 -> [_ _]
                  tunnel: w285 -> [_ _]
                  tunnel: w284 -> [_ w346]
                  tunnel: w283 -> [_ w331]
                  tunnel: [w298 w328] -> w282
                  tunnel: [w296 w325] -> w281
                  tunnel: [w296 w319] -> w280
                  tunnel: [w297 w316] -> w279
                  tunnel: w278 -> [_ w320]
                  tunnel: w277 -> [_ w321]
                  tunnel: w276 -> [_ w309]
                  frame False {
                    w297 = sgl 0.0 ("f")
                    w296 = FALSE
                    w299 = 0
                    w300 = sgl 0.0
                    (unwired) FALSE
                    # "FALSE"
                    # "1 Valid Data Set\n\nRun Single Position Calc for each?\n\nor estimate position based on previous \nposition and orientation"
                    n105 = Build Array(w300, w300, w300) -> ()  [unwired: 1 out]
                    n106 = Build Array(w300, w300, w300) -> ()  [unwired: 1 out]
                    n107 = Build Array(w300, w300, w300) -> ()  [unwired: 1 out]
                    n108 = Build Array(w300, w300, w300) -> ()  [unwired: 1 out]
                    n109 = Build Array(w300, w300, w300) -> ()  [unwired: 1 out]
                    n110 = Build Array(w300, w300, w300) -> ()  [unwired: 1 out]
                    n111 = Build Array(w299, w299, w299) -> ()  [unwired: 1 out]
                    n112 = Bundle("f"=w297, "f"=w297) -> (w298:cluster{"f":sgl, "f":sgl})  [unwired: 1 in]
                  }
                  frame True {
                    w357 = sgl 2.0
                    w376 = 0
                    # "Only Apply This Filtering \nif 3 or More Beacons Still Valid"
                    # "Orientation Value"
                    # "Orientation Valid"
                    # "Y (current)"
                    # "X (current)"
                    # "Number of Valid\nPrevious Orientations"
                    # "Position Valid Shift Array"
                    # "More than 1 Previous\nValid Positions"
                    # "More than\n1 previous position\navailable"
                    # "Choose Beacon Set\nwith Lowest Std Dev"
                    # "Y value cannot be negative"
                    # "Find New # Of Valid Beacons"
                    # "Adjust/Normalize\nLocal Beacon Positions\nusing Line of Best fit"
                    # "# Valid\nData Sets"
                    # "cam, y"
                    # "cam, x"
                    # "Calculate dX and dY\nfor right cam"
                    # "Average dX and dY from each (valid) beacon to find position of each camera\n\nthen average all  positions for each camera find center between"
                    # "Convert Slope\nto Radians"
                    # "*rotate CCW in rad"
                    # "Rotate Coordinate\n System by Slope"
                    # "2+ Data Sets"
                    n113 = for {
                      N: w313 -> [_]
                      tunnel: w383 -> [w684] mode=indexing
                      tunnel: w382 -> [w688] mode=indexing
                      tunnel: w381 -> [w687] mode=indexing
                      tunnel: [w686] -> w339 mode=indexing
                      tunnel: [w685] -> w338 mode=indexing
                      tunnel: [w683] -> w324 mode=indexing
                      n114 = case shown="True" w684 {
                        selector: w684 -> [w690 w694]
                        tunnel: w688 -> [_ w702]
                        tunnel: [w689 w692] -> w686
                        tunnel: [w689 w693] -> w685
                        tunnel: w687 -> [_ w691]
                        tunnel: [w690 w694] -> w683
                        frame False {
                          w689 = sgl 0.0
                          # "Current Data Set Was Not Valid\nFill with 0\nWill not be used later"
                        }
                        frame True {
                          # "dY"
                          # "dX"
                          # "Negate dX if A2>90"
                          # "Find LOCAL Coordinate of Each Beacon"
                          # "Current - Valid Data Set"
                          n115 = Less?(x=w702, y=sgl 90.0) -> (x < y?=w704:bool)
                          n116 = case shown="False" w704 {
                            tunnel: w702 -> [w711 w713]
                            tunnel: [w709 w714] -> w701
                            tunnel: [FALSE TRUE] -> w696
                            frame False {
                              # "Negative Y"
                              # "A2 is > 90"
                              n117 = Subtract(x=w711, y=sgl 90.0) -> (x-y=w709:sgl)
                            }
                            frame True {
                              # "Positive Y"
                              # "A2 is < 90"
                              n118 = Subtract(x=sgl 90.0, y=w713) -> (x-y=w714:sgl)
                            }
                          }
                          "dA2" <- w701
                          n119 = expression code="(x/180.0)*pi" "degrees to radians"(w701) -> (w699:sgl)
                          n120 = expression code="(x/180.0)*pi" "degrees to radians"(w701) -> (w700:sgl)
                          n121 = Cosine(x=w699) -> (cos(x)=w697:sgl)
                          n122 = Sine(x=w700) -> (sin(x)=w698:sgl)
                          n123 = Multiply(x=w691, y=w697) -> (x*y=w693:sgl)
                          n124 = Multiply(x=w691, y=w698) -> (x*y=w695:sgl)
                          n125 = case shown="True" w696 {
                            tunnel: w695 -> [w706 w707]
                            tunnel: [w705 w707] -> w692
                            frame False {
                              n126 = Negate(x=w706) -> (-x=w705:sgl)
                            }
                            frame True {
                            }
                          }
                        }
                      }
                    }
                    n127 = Boolean To (0,1)(Boolean=w320) -> (0, 1=w334:i16[])
                    n128 = Add Array Elements(numeric array=w334) -> (sum=w318:i16)
                    n129 = Greater?(x=w318, y=1) -> (0:w322:bool)
                    n130 = Bundle(w339, w338) -> (→"LOCAL\nBeacon Coordinates\nRelative to Robot" →"Local Coordinates - Calculated":cluster{sgl[], sgl[]})  [unwired: 1 in]
                    n131 = call "Coordinate_Outlier_Filtering_R2.vi"("Num of Beacons"=w313, "Max Std Dev(all 5)"="Max Std Dev (5)", "X in"=w339, "Valid Data\nSets in"=w324, "Y in"=w338, "Max Std Dev( 4 )"="Max Std Dev (4)", "Max Std Dev (3)"="Max Std Dev (3)") -> ("Y out"=w311:sgl[], "X out"=w312:sgl[], "Valid Beacons\nout"=w308:bool[], "Slope out"=w327:dbl)  [unwired: 3 in, 2 out]
                    n132 = Inverse Tangent(1:w327) -> (0:w351:dbl)
                    n133 = expression code="(x/pi)*180.0" "radians to degrees"(w351) -> (w326:dbl)
                    n134 = Boolean To (0,1)(Boolean=w308) -> (0, 1=w307:i16[])
                    n135 = To Single Precision Float(number=w326) -> (single precision float=w317:sgl)
                    "Orietnation\n(current)" <- w317
                    n136 = case shown="True" w322 {
                      tunnel: w320 -> [_ w417]
                      tunnel: [w393 w403] -> w319
                      tunnel: w321 -> [_ w404]
                      tunnel: w317 -> [w394 w398]
                      tunnel: [w392 w399] -> w316
                      tunnel: w309 -> [_ _]
                      frame False {
                        # "Since no history available,\ncheck that current is with 0-360"
                        # "Use Current Orientation bc \nPrevious are not available"
                        # "New Position\nValid"
                        n137 = In Range and Coerce(upper limit=sgl 360.0, x=w394, lower limit=sgl -360.0 ("upper limit")) -> (In Range?=w393:bool)  [unwired: 1 out]
                        n138 = Select(t=w394, s=w393, f=sgl 0.0) -> (s? t:f=w392:sgl)
                      }
                      frame True {
                        # "Valid Position Ccount\n(up to 2)"
                        # "Weighted\nOrientation"
                        # "New \nWeight"
                        # "Weighted Orientation (new)"
                        # "Position\nValid\n(current)\n\nbased on orientation"
                        # "Only Calculate MOving Avg\nif xx% of previous positions were valid"
                        n139 = Initialize Array(u8 0, u8 2) -> (w412:u8[])
                        n140 = local read "History Size"() -> (w413:u8)
                        n141 = while {
                          shift-right: [w468] -> w405
                          shift-left: w412 -> [w470]
                          tunnel: w417 -> [w477] mode=indexing
                          shift-right: [w475] -> w410
                          shift-left: u8 0 -> [w478]
                          tunnel: w413 -> [w476]
                          i -> [w469]
                          stop <- w471 stop-if-true
                          # "Grab Last 2 Valid Position Indexes"
                          n142 = case shown="True" w477 {
                            tunnel: w478 -> [w480 w482]
                            tunnel: [w480 w485] -> w475
                            tunnel: w470 -> [w479 w484]
                            tunnel: w469 -> [_ w483]
                            tunnel: [w479 w481] -> w468
                            frame False {
                            }
                            frame True {
                              # "Update Index\nto use"
                              # "Increment\nValid Count"
                              n143 = Replace Array Subset(array=w484, new element=w483, index=w482) -> (w481:u8[])
                              n144 = Increment(x=w482) -> (x+1=w485:u8)
                            }
                          }
                          n145 = Greater?(x=w469, y=w476) -> (0:w472:bool)
                          n146 = Greater?(x=w475, y=u8 2) -> (0:w473:bool)
                          n147 = Or(x=w473, y=w472) -> (x .or. y?=w471:bool)
                        }
                        n148 = case shown="2, Default" w410 {
                          tunnel: w405 -> [_ w452 w464]
                          tunnel: w404 -> [_ w453 w463]
                          tunnel: [sgl 0.0 ("y") w446 w459] -> w408
                          tunnel: "Orientation (-2) \nWeight" -> [w438 w449 w458]
                          tunnel: "Orientation (-1) \nWeight" -> [w440 w442 w456]
                          tunnel: "New Orientation\nWeight" -> [w439 w444 w457]
                          tunnel: [w437 w443 w457] -> w409
                          frame 0 {
                            n149 = Compound Arithmetic op=ADD(w440, w439, w438) -> (w437:sgl)
                          }
                          frame 1 {
                            # "Grab Last 1 Valid Position Values"
                            n150 = Index Array(array=w452, index=u8 0) -> (element=w450:u8)
                            n151 = Index Array(array=w453, index=w450) -> (element=w441:sgl)
                            n152 = Divide(x=w449, y=sgl 2.0) -> (x/y=w445:sgl)
                            n153 = Add(x=w442, y=w445) -> (x+y=w447:sgl)
                            n154 = Add(x=w445, y=w444) -> (x+y=w443:sgl)
                            n155 = Multiply(x=w441, y=w447) -> (x*y=w446:sgl)
                          }
                          frame 2, Default {
                            # "weighted vals"
                            # "Grab Last 2 Valid Position Values"
                            n156 = Index Array(array=w464, index=u8 0) -> (element=w466:u8)
                            n157 = Index Array(array=w464, index=u8 1) -> (element=w462:u8)
                            n158 = Index Array(array=w463, index=w466) -> (element=w455:sgl)
                            n159 = Index Array(array=w463, index=w462) -> (element=w454:sgl)
                            n160 = Multiply(x=w456, y=w455) -> (x*y=w460:sgl)
                            n161 = Multiply(x=w454, y=w458) -> (x*y=w461:sgl)
                            n162 = Add(x=w460, y=w461) -> (x+y=w459:sgl)
                          }
                        }
                        n163 = Multiply(x=w398, y=w409) -> (x*y=w407:sgl)
                        n164 = Add(x=w407, y=w408) -> (x+y=w406:sgl)
                        n165 = Greater Than 0?(x=w410) -> (x > 0?=w411:bool)
                        n166 = case shown="True" w411 {
                          tunnel: w406 -> [w420 w425]
                          tunnel: w405 -> [_ w433]
                          tunnel: w404 -> [_ w432]
                          tunnel: [w419 w424] -> w399
                          tunnel: [w418 w427] -> w403
                          frame False {
                            # "No Pevious is Available to Compare\ncheck that current is real angle"
                            n167 = In Range and Coerce(upper limit=sgl 360.0, x=w420, lower limit=sgl -360.0 ("upper limit")) -> (In Range?=w418:bool)  [unwired: 1 out]
                            n168 = Select(t=w420, s=w418, f=sgl 0.0) -> (s? t:f=w419:sgl)
                          }
                          frame True {
                            # "Calculate New, Weighted\nOrientation"
                            # "Check That New Value\nis within Range of Old\n(avg)"
                            # "(X1 - X2)^2"
                            # "Previous"
                            # "Pevious is Available to Compare"
                            n169 = Index Array(array=w433, index=u8 0) -> (element=w434:u8)
                            n170 = Index Array(array=w432, index=w434) -> (element=w430:sgl)
                            n171 = Subtract(x=w430, y=w425) -> (x-y=w429:sgl)
                            n172 = Absolute Value(x=w429) -> (abs(x)=w428:sgl)
                            n173 = Less Or Equal?(x=w428, y="New Orientation \nThreshold") -> (x <= y?=w427:bool)
                            n174 = Select(t=w425, s=w427, f=sgl 0.0) -> (s? t:f=w424:sgl)
                          }
                        }
                      }
                    }
                    n175 = Add Array Elements(numeric array=w307) -> (sum=w306:i16)
                    n176 = Greater?(x=w306, y=i16 2) -> (0:w304:bool)
                    n177 = case shown="True" w304 {
                      tunnel: w313 -> [_ w391]
                      tunnel: w308 -> [w384 w390]
                      tunnel: w312 -> [_ w389]
                      tunnel: w311 -> [_ w388]
                      tunnel: [w384 w387] -> w310
                      tunnel: "Distance\nBetween Beacons" -> [_ w386]
                      tunnel: "Distance\nBetween Beacons \n- Tolerance" -> [_ w385]
                      frame False {
                        # "Don't apply filtering,\nnot enough data points"
                      }
                      frame True {
                        # "This will filter beacons if they are calculate to be \ntoo close to each other. The beacon(s) that is\n discarded is chosen based distance between each/every\nbeacon,. Capable of filtering as long as 1/2 of sample\nset has uniform distances (between beacons)."
                        # "Validate Distance Between\nEach Beacon"
                        n178 = call "Beacon_Filtering_Inter_Beacon_Distance_R1.vi"("Num of Beacons"=w391, "Inter Beacon\nReal Distance"=w386, "X in"=w389, "Inter Beacon\ndelta Threshold"=w385, "Y in"=w388, "Valid Data\nSets in"=w390) -> ("Beacons Valid - Out"=w387:bool[])  [unwired: 9 in]
                      }
                    }
                    "Post Filtering\n- Valid Beacons" <- w310
                    n179 = Bundle("X out"=w312, "Y out"=w311) -> (→"Normalized Beacons\nCoordinates Relative\nto Robot\n- Local" →"Local Coordinates - Adjusted":cluster{"X out":sgl[], "Y out":sgl[]})  [unwired: 1 in]
                    n180 = Increment(x=w313) -> (x+1=w377:i8)
                    n181 = for {
                      N: w377 -> [_]
                      tunnel: [w673] -> w379 mode=indexing
                      tunnel: w312 -> [w669]
                      tunnel: w311 -> [w672]
                      tunnel: [w671] -> w380 mode=indexing
                      tunnel: w346 -> [w668]
                      i -> [w670]
                      # "Build Array's of Coordinates\nFor All Objects"
                      n182 = Greater Than 0?(x=w670) -> (x > 0?=w674:bool)
                      n183 = case shown="True" w674 {
                        tunnel: [w676 w682] -> w673
                        tunnel: w669 -> [w679 _]
                        tunnel: w672 -> [w678 _]
                        tunnel: [w675 0.0] -> w671
                        tunnel: w670 -> [w680 _]
                        tunnel: w668 -> [_ w682]
                        frame True {
                          # "Rest of Array is\nBeacon Coordinates"
                          n184 = Decrement(x=w680) -> (x-1=w677:i32)
                          n185 = Index Array(array=w679, index=w677) -> (element=w676:sgl)
                          n186 = Index Array(array=w678, index=w677) -> (element=w675:sgl)
                        }
                        frame False {
                          # "First object is the\nother Camera\n\nthis coordinate\nis simply:\nx = 0\ny = distance btween cams"
                        }
                      }
                    }
                    n187 = Bundle(w379, w380) -> (→"All Object Coordinates \n- Local" →"Local Coordinates - Normalized":cluster{sgl[], dbl[]})  [unwired: 1 in]
                    n188 = expression code="(x/180.0)*pi" "degrees to radians"(w316) -> (w323:sgl)
                    n189 = call-poly <vilib>:"2D Cartesian Coordinate Rotation.vi"("theta"=w323, "Y"=w380, "X"=w379) -> ("Y Out"=w354:dbl[], "X Out"=w355:dbl[])  [unwired: 6 in, 1 out]
                    n190 = Bundle("X Out"=w355, "Y Out"=w354) -> (→"All Object Coordinates \n- Local - Rotated" →"Local Coordinates - Rotated":cluster{"X Out":dbl[], "Y Out":dbl[]})  [unwired: 1 in]
                    n191 = Index Array(array=w354, index=w376) -> (element=w347:dbl)
                    n192 = Index Array(array=w355, index=w376) -> (element=w375:dbl)
                    n193 = for {
                      N: w313 -> [_]
                      tunnel: w354 -> [w664]
                      tunnel: w355 -> [w665]
                      tunnel: w375 -> [w663]
                      tunnel: w347 -> [w662]
                      tunnel: [w661] -> w343 mode=indexing
                      tunnel: [w660] -> w342 mode=indexing
                      tunnel: [w659] -> w301 mode=indexing
                      tunnel: [w658] -> w344 mode=indexing
                      i -> [w667]
                      n194 = Increment(x=w667) -> (x+1=w666:i32)
                      n195 = Index Array(array=w664, index=w666) -> (element=w658:dbl)
                      n196 = Index Array(array=w665, index=w666) -> (element=w659:dbl)
                      n197 = Subtract(x=w658, y=w662) -> (x-y=w660:dbl)
                      n198 = Subtract(x=w659, y=w663) -> (x-y=w661:dbl)
                    }
                    n199 = Bundle(w343, w342) -> (→"dX, dY\nRight Cam":cluster{dbl[], dbl[]})  [unwired: 1 in]
                    n200 = Bundle(w301, w344) -> (→"dX, dY\nLeft Cam":cluster{dbl[], dbl[]})  [unwired: 1 in]
                    n201 = Unbundle("Real Beacon\n - Coordinates") -> ("X"=w372:dbl[], "Y"=w348:dbl[])
                    n202 = Boolean To (0,1)(Boolean=w310) -> (0, 1=w345:i16[])
                    n203 = for {
                      N: w313 -> [_]
                      tunnel: w310 -> [w644] mode=indexing
                      tunnel: w372 -> [w641] mode=indexing
                      tunnel: w348 -> [w640] mode=indexing
                      tunnel: w301 -> [w643] mode=indexing
                      tunnel: w344 -> [w639] mode=indexing
                      tunnel: w343 -> [w642] mode=indexing
                      tunnel: w342 -> [w638] mode=indexing
                      tunnel: [w637] -> w371 mode=indexing
                      tunnel: [w636] -> w370 mode=indexing
                      tunnel: [w635] -> w369 mode=indexing
                      tunnel: [w634] -> w368 mode=indexing
                      n204 = case shown="True" w644 {
                        tunnel: w643 -> [_ w657]
                        tunnel: w642 -> [_ w656]
                        tunnel: w641 -> [_ w647]
                        tunnel: w640 -> [_ w646]
                        tunnel: w639 -> [_ w655]
                        tunnel: w638 -> [_ w648]
                        tunnel: [w645 w653] -> w637
                        tunnel: [w645 w652] -> w636
                        tunnel: [w645 w651] -> w635
                        tunnel: [w645 w650] -> w634
                        frame False {
                          w645 = sgl 0.0
                          # "Add Nothing"
                        }
                        frame True {
                          # "realX = beaconX + dY\nrealY = beaconY + (-dx)"
                          # "Right Cam"
                          # "Left Cam"
                          # "dX = -dX\nSwap dX, dY"
                          # "Translate to Real Coordinates\nOnly Apply for Valid Beacons"
                          n205 = Negate(x=w657) -> (-x=w654:dbl)
                          n206 = Negate(x=w656) -> (-x=w649:dbl)
                          n207 = Add(x=w647, y=w655) -> (x+y=w653:dbl)
                          n208 = Add(x=w646, y=w654) -> (x+y=w652:dbl)
                          n209 = Add(x=w647, y=w648) -> (x+y=w651:dbl)
                          n210 = Add(x=w646, y=w649) -> (x+y=w650:dbl)
                        }
                      }
                    }
                    n211 = Add Array Elements(numeric array=w345) -> (sum=w349:i16)
                    n212 = Add Array Elements(numeric array=w371) -> (sum=w367:dbl)
                    n213 = Add Array Elements(numeric array=w370) -> (sum=w366:dbl)
                    n214 = Add Array Elements(numeric array=w369) -> (sum=w365:dbl)
                    n215 = Add Array Elements(numeric array=w368) -> (sum=w364:dbl)
                    n216 = Divide(x=w367, y=w349) -> (x/y=w362:dbl)
                    n217 = Divide(x=w366, y=w349) -> (x/y=w360:dbl)
                    n218 = Divide(x=w365, y=w349) -> (x/y=w361:dbl)
                    n219 = Divide(x=w364, y=w349) -> (x/y=w359:dbl)
                    n220 = Bundle(w362, w360) -> (→"Left Camera Real Coordinates":cluster{dbl, dbl})  [unwired: 1 in]
                    n221 = Bundle(w361, w359) -> (→"Right Camera Real Coordinate":cluster{dbl, dbl})  [unwired: 1 in]
                    n222 = Add(x=w362, y=w361) -> (x+y=w358:dbl)
                    n223 = Add(x=w360, y=w359) -> (x+y=w356:dbl)
                    n224 = Divide(x=w358, y=w357) -> (x/y=w330:dbl)
                    n225 = Divide(x=w356, y=w357) -> (x/y=w329:dbl)
                    n226 = Bundle(w330, w329) -> (→"Robot Coordinates":cluster{dbl, dbl})  [unwired: 1 in]
                    n227 = case shown="False" w322 {
                      tunnel: w320 -> [_ w524]
                      tunnel: w318 -> [_ _]
                      tunnel: w330 -> [w490 w512]
                      tunnel: [w491 w502] -> w325
                      tunnel: w331 -> [_ w497]
                      tunnel: w329 -> [w489 w511]
                      tunnel: [w488 w523] -> w328
                      tunnel: "Max X (arena)" -> [w487 w500]
                      tunnel: "Max Y (arena)" -> [w486 w499]
                      frame False {
                        # "New Position\nValid"
                        # "Since no history available,\ncheck that current is within\nthe bounds of the arena size"
                        # "Use Current Position bc \nPrevious are not available"
                        n228 = In Range and Coerce(upper limit=w487, x=w490, lower limit=sgl 0.0 ("upper limit")) -> (In Range?=w493:bool)  [unwired: 1 out]
                        n229 = In Range and Coerce(upper limit=w486, x=w489, lower limit=sgl 0.0 ("upper limit")) -> (In Range?=w492:bool)  [unwired: 1 out]
                        n230 = Bundle(w490, w489) -> (w488:cluster{dbl, dbl})  [unwired: 1 in]
                        n231 = And(x=w493, y=w492) -> (x .and. y?=w491:bool)
                      }
                      frame True {
                        # "Only consider if velocity is\ngreater than certain speed"
                        # "Valid Position Ccount\n(up to 2)"
                        # "Weighted Y"
                        # "Weighted X"
                        # "New Pos\nWeight"
                        # "Weighted Robot \nCoordinates"
                        # "Position\nValid\n(current)"
                        # "Only Calculate MOving Avg\nif xx% of previous positions were valid"
                        n232 = Initialize Array(u8 0, u8 2) -> (w518:u8[])
                        n233 = local read "History Size"() -> (w519:u8)
                        n234 = while {
                          shift-right: [w617] -> w496
                          shift-left: w518 -> [w619]
                          tunnel: w524 -> [w625] mode=indexing
                          shift-right: [w623] -> w514
                          shift-left: u8 0 -> [w626]
                          tunnel: w519 -> [w624]
                          tunnel: [w616] -> w498
                          i -> [w618]
                          stop <- w620 stop-if-true
                          # "Grab Last 3 Valid Position Indexes"
                          n235 = case shown="True" w625 {
                            tunnel: w626 -> [w628 w630]
                            tunnel: [w628 w633] -> w623
                            tunnel: w619 -> [w627 w632]
                            tunnel: w618 -> [_ w631]
                            tunnel: [w627 w629] -> w617
                            frame False {
                            }
                            frame True {
                              # "Update Index\nto use"
                              # "Increment\nValid Count"
                              n236 = Replace Array Subset(array=w632, new element=w631, index=w630) -> (w629:u8[])
                              n237 = Increment(x=w630) -> (x+1=w633:u8)
                            }
                          }
                          n238 = Greater?(x=w618, y=w624) -> (0:w621:bool)
                          n239 = Greater?(x=w623, y=u8 2) -> (0:w616:bool)
                          n240 = Or(x=w616, y=w621) -> (x .or. y?=w620:bool)
                        }
                        n241 = case shown="True" w498 {
                          tunnel: w497 -> [_ w546]
                          tunnel: w496 -> [_ w532]
                          frame False {
                          }
                          frame True {
                            # "Angle between p(1) - p(2)"
                            # "Angle between p(0) - p(1)"
                            # "Calculate Orientation Based on Recent Positions"
                            # "*******"
                            n242 = Index Array(array=w532, index #1=0, index #2=1, index #3=2) -> (element #1=w528:u8, element #2=w527:u8, element #3=w526:u8)
                            n243 = Index Array(array=w546, index=w528) -> (element=w545:cluster{sgl, sgl})
                            n244 = Unbundle(w545) -> (w542:sgl, w541:sgl)
                            n245 = Index Array(array=w546, index=w527) -> (element=w544:cluster{sgl, sgl})
                            n246 = Unbundle(w544) -> (w534:sgl, w533:sgl)
                            n247 = Subtract(x=w542, y=w534) -> (x-y=w543:sgl)
                            n248 = Subtract(x=w541, y=w533) -> (x-y=w540:sgl)
                            n249 = Inverse Tangent (2 Input)(1:w540, 2:w543) -> (0:→"atan2(y,x)":sgl)
                            n250 = Index Array(array=w546, index=w526) -> (element=w535:cluster{sgl, sgl})
                            n251 = Unbundle(w535) -> (w538:sgl, w537:sgl)
                            n252 = Subtract(x=w534, y=w538) -> (x-y=w539:sgl)
                            n253 = Subtract(x=w533, y=w537) -> (x-y=w536:sgl)
                            n254 = Inverse Tangent (2 Input)(1:w536, 2:w539) -> ()  [unwired: 1 out]
                          }
                        }
                        n255 = case shown="2, Default" w514 {
                          tunnel: w496 -> [_ w593 w613]
                          tunnel: w497 -> [_ w594 w612]
                          tunnel: [w574 w583 w601] -> w510
                          tunnel: [w574 w582 w600] -> w509
                          tunnel: "position(-2) weight" -> [w576 w587 w599]
                          tunnel: "position(-1) weight" -> [w578 w585 w598]
                          tunnel: "New Position\nWeight" -> [w577 w580 w597]
                          tunnel: [w575 w579 w597] -> w513
                          frame 0 {
                            w574 = sgl 0.0 ("y")
                            n256 = Compound Arithmetic op=ADD(w578, w577, w576) -> (w575:sgl)
                          }
                          frame 1 {
                            # "Grab Last 1 Valid Position Values"
                            n257 = Index Array(array=w593, index=u8 0) -> (element=w591:u8)
                            n258 = Index Array(array=w594, index=w591) -> (element=w588:cluster{sgl, sgl})
                            n259 = Unbundle(w588) -> (w589:sgl, w590:sgl)
                            n260 = Divide(x=w587, y=sgl 2.0) -> (x/y=w581:sgl)
                            n261 = Add(x=w585, y=w581) -> (x+y=w584:sgl)
                            n262 = Add(x=w581, y=w580) -> (x+y=w579:sgl)
                            n263 = Multiply(x=w589, y=w584) -> (x*y=w583:sgl)
                            n264 = Multiply(x=w590, y=w584) -> (x*y=w582:sgl)
                          }
                          frame 2, Default {
                            # "weighted vals"
                            # "Grab Last 2 Valid Position Values"
                            n265 = Index Array(array=w613, index #1=u8 0, index #2=u8 1) -> (element #1=w614:u8, element #2=w595:u8)
                            n266 = Index Array(array=w612, index=w614) -> (element=w611:cluster{sgl, sgl})
                            n267 = Index Array(array=w612, index=w595) -> (element=w610:cluster{sgl, sgl})
                            n268 = Unbundle(w611) -> (w608:sgl, w609:sgl)
                            n269 = Unbundle(w610) -> (w607:sgl, w606:sgl)
                            n270 = Multiply(x=w608, y=w598) -> (x*y=w604:sgl)
                            n271 = Multiply(x=w609, y=w598) -> (x*y=w603:sgl)
                            n272 = Multiply(x=w607, y=w599) -> (x*y=w605:sgl)
                            n273 = Multiply(x=w606, y=w599) -> (x*y=w602:sgl)
                            n274 = Add(x=w604, y=w605) -> (x+y=w601:sgl)
                            n275 = Add(x=w603, y=w602) -> (x+y=w600:sgl)
                          }
                        }
                        n276 = Multiply(x=w512, y=w513) -> (x*y=w507:dbl)
                        n277 = Multiply(x=w511, y=w513) -> (x*y=w508:dbl)
                        n278 = Greater Than 0?(x=w514) -> (x > 0?=w515:bool)
                        n279 = Add(x=w507, y=w510) -> (x+y=w506:dbl)
                        n280 = Add(x=w508, y=w509) -> (x+y=w505:dbl)
                        n281 = case shown="True" w515 {
                          tunnel: w506 -> [w551 w558]
                          tunnel: w505 -> [w550 w557]
                          tunnel: w496 -> [_ w570]
                          tunnel: w497 -> [_ w569]
                          tunnel: [w548 w558] -> w504
                          tunnel: [w547 w557] -> w503
                          tunnel: [w552 w559] -> w502
                          tunnel: w500 -> [w554 _]
                          tunnel: w499 -> [w553 _]
                          frame False {
                            w549 = sgl 0.0 ("upper limit")
                            # "Check that within bounds of arena"
                            # "No Pevious is Available to Compare"
                            n282 = In Range and Coerce(upper limit=w554, x=w551, lower limit=w549) -> (In Range?=w556:bool)  [unwired: 1 out]
                            n283 = In Range and Coerce(upper limit=w553, x=w550, lower limit=w549) -> (In Range?=w555:bool)  [unwired: 1 out]
                            n284 = And(x=w556, y=w555) -> (x .and. y?=w552:bool)
                            n285 = Select(t=w551, s=w552, f=w549) -> (s? t:f=w548:dbl)
                            n286 = Select(t=w550, s=w552, f=w549) -> (s? t:f=w547:dbl)
                          }
                          frame True {
                            # "New"
                            # "(Y1 - Y2)^2"
                            # "(X1 - X2)^2"
                            # "Previous"
                            # "Pevious is Available to Compare"
                            n287 = Index Array(array=w570, index=u8 0) -> (element=w572:u8)
                            n288 = Index Array(array=w569, index=w572) -> (element=w571:cluster{sgl, sgl})
                            n289 = Unbundle(w571) -> (w561:sgl, w560:sgl)
                            n290 = Subtract(x=w561, y=w558) -> (x-y=w566:dbl)
                            n291 = Subtract(x=w557, y=w560) -> (x-y=w565:dbl)
                            n292 = Square(x=w566) -> (x^2=w564:dbl)
                            n293 = Square(x=w565) -> (x^2=w563:dbl)
                            n294 = Add(x=w564, y=w563) -> (x+y=w567:dbl)
                            n295 = Square Root(x=w567) -> (sqrt(x)=w562:dbl)
                            n296 = Less Or Equal?(x=w562, y="New Position \nThreshold") -> (x <= y?=w559:bool)
                          }
                        }
                        n297 = Bundle("upper limit"=w504, "upper limit"=w503) -> (w523:cluster{"upper limit":dbl, "upper limit":dbl})  [unwired: 1 in]
                      }
                    }
                    n298 = Less Than 0?(x=w329) -> ()  [unwired: 1 out]
                  }
                }
              }
            }
          }
        }
        n299 = And(x=w134, y=w133) -> (x .and. y?=w137:bool)
        "Position Valid" <- w137
        n300 = Exclusive Or(1:w133, 2:w134) -> (0:w132:bool)
        n301 = case shown="True" w137 {
          tunnel: [w171 w175] -> w150
          tunnel: [w172 w174] -> w122
          tunnel: w152 -> [_ w175]
          tunnel: w151 -> [_ w174]
          tunnel: w132 -> [_ _]
          frame False {
            w171 = sgl 0.0 ("f")
            n302 = Bundle("f"=w171, "f"=w171) -> (w172:cluster{"f":sgl, "f":sgl})  [unwired: 1 in]
          }
          frame True {
            # "For Servos"
            n303 = Unbundle(w174) -> ("upper limit"=w173:dbl)  [unwired: 1 out]
            n304 = shared-variable "RT myRIO Target - Overlord\\Localization_Variables_r0.lvlib\\loc_y"(w173) -> ()  [unwired: 1 in, 1 out]
            n305 = shared-variable "RT myRIO Target - Overlord\\Localization_Variables_r0.lvlib\\loc_x"(w173) -> ()  [unwired: 1 in, 1 out]
            "Last Orientation" <- w175
            "Last Position" <- w174
          }
        }
        "Robot Coordinates - Avgd" <- w122
        "Orientation Avgd" <- w150
        n306 = local read "History Size"() -> (w142:u8)
        n307 = Reverse 1D Array(array=w149) -> (reversed array=w155:cluster{sgl, sgl}[])
        n308 = for {
          N: w142 -> [w213]
          shift-right: [w214] -> w156
          shift-left: w155 -> [w209]
          tunnel: w122 -> [w208]
          i -> [w210]
          n309 = Decrement(x=w213) -> (x-1=w211:i32)
          n310 = Equal?(x=w211, y=w210) -> (x = y?=w212:bool)
          n311 = case shown="True" w212 {
            tunnel: w210 -> [w216 w221]
            tunnel: w209 -> [w219 w222]
            tunnel: [w217 w223] -> w214
            tunnel: w208 -> [_ w220]
            frame False {
              n312 = Increment(x=w216) -> (x+1=w215:i32)
              n313 = Index Array(array=w219, index=w215) -> (element=w218:cluster{sgl, sgl})
              n314 = Replace Array Subset(array=w219, new element=w218, index=w216) -> (w217:cluster{sgl, sgl}[])
            }
            frame True {
              n315 = Replace Array Subset(array=w222, new element=w220, index=w221) -> (w223:cluster{sgl, sgl}[])
            }
          }
        }
        n316 = Reverse 1D Array(array=w148) -> (reversed array=w157:sgl[])
        n317 = Reverse 1D Array(array=w156) -> (reversed array=w145:cluster{sgl, sgl}[])
        n318 = for {
          N: w142 -> [w197]
          shift-right: [w198] -> w158
          shift-left: w157 -> [w193]
          tunnel: w150 -> [w192]
          i -> [w194]
          n319 = Decrement(x=w197) -> (x-1=w195:i32)
          n320 = Equal?(x=w195, y=w194) -> (x = y?=w196:bool)
          n321 = case shown="True" w196 {
            tunnel: w194 -> [w200 w205]
            tunnel: w193 -> [w203 w206]
            tunnel: [w201 w207] -> w198
            tunnel: w192 -> [_ w204]
            frame False {
              n322 = Increment(x=w200) -> (x+1=w199:i32)
              n323 = Index Array(array=w203, index=w199) -> (element=w202:sgl)
              n324 = Replace Array Subset(array=w203, new element=w202, index=w200) -> (w201:sgl[])
            }
            frame True {
              n325 = Replace Array Subset(array=w206, new element=w204, index=w205) -> (w207:sgl[])
            }
          }
        }
        n326 = Reverse 1D Array(array=w147) -> (reversed array=w153:bool[])
        n327 = Reverse 1D Array(array=w158) -> (reversed array=w146:sgl[])
        n328 = for {
          N: w142 -> [w181]
          shift-right: [w182] -> w154
          shift-left: w153 -> [w177]
          tunnel: w137 -> [w176]
          i -> [w178]
          n329 = Decrement(x=w181) -> (x-1=w179:i32)
          n330 = Equal?(x=w179, y=w178) -> (x = y?=w180:bool)
          n331 = case shown="True" w180 {
            tunnel: w178 -> [w184 w189]
            tunnel: w177 -> [w187 w190]
            tunnel: [w185 w191] -> w182
            tunnel: w176 -> [_ w188]
            frame False {
              n332 = Increment(x=w184) -> (x+1=w183:i32)
              n333 = Index Array(array=w187, index=w183) -> (element=w186:bool)
              n334 = Replace Array Subset(array=w187, new element=w186, index=w184) -> (w185:bool[])
            }
            frame True {
              n335 = Replace Array Subset(array=w190, new element=w188, index=w189) -> (w191:bool[])
            }
          }
        }
        n336 = Reverse 1D Array(array=w154) -> (reversed array=w141:bool[])
        n337 = Boolean To (0,1)(Boolean=w141) -> (0, 1=w140:i16[])
        n338 = Add Array Elements(numeric array=w140) -> (sum=w139:i16)
        n339 = Greater Or Equal?(x=w139, y=i16 2) -> (x >= y?=w123:bool)
        "Position \nLock Status" <- w123
        n340 = shared-variable "RT myRIO Target - Overlord\\Localization_Variables_r0.lvlib\\loc_flag"(w123) -> ()  [unwired: 1 in, 1 out]
        n341 = case shown="True" w137 {
          tunnel: w122 -> [_ w170]
          frame False {
          }
          frame True {
            # "update debug graph\nif current is valid"
            n342 = Unbundle(w170) -> ("upper limit"=w169:dbl, "upper limit"=w168:dbl)
            n343 = Build Array(w168) -> (w166:dbl[])
            n344 = Build Array(w169) -> (w167:dbl[])
            n345 = Bundle(w167, w166) -> (→"Real Position in Course 2":cluster{dbl[], dbl[]})  [unwired: 1 in]
          }
        }
      }
    }
    n346 = case shown="True" w105 {
      tunnel: w104 -> [_ w112]
      frame False {
      }
      frame True {
        n347 = call "Tick Count3"() -> ("Tick Count(uSec)"=w113:u32)
        n348 = Subtract(x=w113, y=w112) -> (x-y=w116:u32)
        n349 = Divide(x=w116, y=u32 1000 ("x")) -> (x/y=→"dT":dbl)
      }
    }
    n350 = call "Tick Count6"() -> ("Tick Count(uSec)"=w102:u32)
    "Robot Coordinates\nHistory" <- w101
    "Orientation\nHistory" <- w106
    "Position Valid\nHistory" <- w107
  }
  n351 = disable-structure shown="Disabled" {
    frame Disabled {
      w748 = sgl 0.0
      # "Y"
      # "X"
      n352 = Bundle(w748, w748) -> (w745:cluster{sgl, sgl})  [unwired: 1 in]
      n353 = Initialize Array(w748, 10 ("dimension size")) -> (w742:sgl[])
      n354 = Initialize Array(FALSE, 10 ("dimension size")) -> (w743:bool[])
      n355 = local read "Real Beacon\n - Coordinates"() -> (w749:cluster{"X":dbl[], "Y":dbl[]})
      n356 = Unbundle(w749) -> ("X"=w747:dbl[], "Y"=w746:dbl[])
      n357 = while {
        shift-right: [w775] -> _
        shift-left: w742 -> [w776]
        shift-right: [w759] -> _
        shift-left: w743 -> [w779]
        shift-right: [w761] -> _
        shift-left: w742 -> [w780]
        shift-right: [w762] -> _
        shift-left: w745 -> [w764]
        shift-right: [w758] -> _
        shift-left: FALSE -> [w763]
        tunnel: w747 -> [w755]
        tunnel: w746 -> [w754]
        stop <- FALSE stop-if-true
        w760 = 0
        w772 = 5
        # "Update Shift Regs"
        # "Update Shift Arrays"
        n358 = local read "Robot Coordinates"() -> (w768:cluster{"X":sgl, "Y":sgl})
        n359 = local read "Position Valid"() -> (w769:bool)
        n360 = Unbundle(w768) -> ("X"=w778:sgl, "Y"=w777:sgl)
        n361 = Reverse 1D Array(array=w779) -> (reversed array=w781:bool[])
        n362 = Reverse 1D Array(array=w780) -> (reversed array=w787:sgl[])
        n363 = Reverse 1D Array(array=w776) -> (reversed array=w784:sgl[])
        n364 = for {
          N: 10 -> [w876]
          shift-right: [w877] -> w789
          shift-left: w787 -> [w872]
          tunnel: w778 -> [w871]
          i -> [w873]
          n365 = Decrement(x=w876) -> (x-1=w874:i32)
          n366 = Equal?(x=w874, y=w873) -> (x = y?=w875:bool)
          n367 = case shown="True" w875 {
            tunnel: w873 -> [w879 w884]
            tunnel: w872 -> [w882 w885]
            tunnel: [w880 w886] -> w877
            tunnel: w871 -> [_ w883]
            frame False {
              n368 = Increment(x=w879) -> (x+1=w878:i32)
              n369 = Index Array(array=w882, index=w878) -> (element=w881:sgl)
              n370 = Replace Array Subset(array=w882, new element=w881, index=w879) -> (w880:sgl[])
            }
            frame True {
              n371 = Replace Array Subset(array=w885, new element=w883, index=w884) -> (w886:sgl[])
            }
          }
        }
        n372 = for {
          N: 10 -> [w860]
          shift-right: [w861] -> w786
          shift-left: w784 -> [w856]
          tunnel: w777 -> [w855]
          i -> [w857]
          n373 = Decrement(x=w860) -> (x-1=w858:i32)
          n374 = Equal?(x=w858, y=w857) -> (x = y?=w859:bool)
          n375 = case shown="True" w859 {
            tunnel: w857 -> [w863 w868]
            tunnel: w856 -> [w866 w869]
            tunnel: [w864 w870] -> w861
            tunnel: w855 -> [_ w867]
            frame False {
              n376 = Increment(x=w863) -> (x+1=w862:i32)
              n377 = Index Array(array=w866, index=w862) -> (element=w865:sgl)
              n378 = Replace Array Subset(array=w866, new element=w865, index=w863) -> (w864:sgl[])
            }
            frame True {
              n379 = Replace Array Subset(array=w869, new element=w867, index=w868) -> (w870:sgl[])
            }
          }
        }
        n380 = for {
          N: 10 -> [w844]
          shift-right: [w845] -> w783
          shift-left: w781 -> [w840]
          tunnel: w769 -> [w839]
          i -> [w841]
          n381 = Decrement(x=w844) -> (x-1=w842:i32)
          n382 = Equal?(x=w842, y=w841) -> (x = y?=w843:bool)
          n383 = case shown="False" w843 {
            tunnel: w841 -> [w847 w852]
            tunnel: w840 -> [w850 w853]
            tunnel: [w848 w854] -> w845
            tunnel: w839 -> [_ w851]
            frame False {
              n384 = Increment(x=w847) -> (x+1=w846:i32)
              n385 = Index Array(array=w850, index=w846) -> (element=w849:bool)
              n386 = Replace Array Subset(array=w850, new element=w849, index=w847) -> (w848:bool[])
            }
            frame True {
              n387 = Replace Array Subset(array=w853, new element=w851, index=w852) -> (w854:bool[])
            }
          }
        }
        n388 = Reverse 1D Array(array=w783) -> (reversed array=w759:bool[])
        n389 = Reverse 1D Array(array=w786) -> (reversed array=w775:sgl[])
        n390 = Reverse 1D Array(array=w789) -> (reversed array=w761:sgl[])
        n391 = Boolean To (0,1)(Boolean=w759) -> (0, 1=w774:i16[])
        n392 = Add Array Elements(numeric array=w774) -> (sum=w767:i16)
        n393 = Greater Or Equal?(x=w767, y=3) -> (x >= y?=w765:bool)
        n394 = case shown="True" w765 {
          tunnel: w775 -> [_ w808]
          tunnel: w761 -> [_ w807]
          tunnel: w759 -> [_ w802]
          tunnel: w767 -> [_ w801]
          tunnel: [w793 w794] -> w762
          tunnel: w764 -> [w793 w800]
          tunnel: "New Pos\nThreshold (*unit)\nfilterd UNUSED" -> [_ w799]
          tunnel: w763 -> [_ w798]
          tunnel: [FALSE w797] -> w758
          tunnel: [w791 w796] -> w757
          tunnel: [w791 w795] -> w756
          frame False {
            w791 = sgl 0.0
            # "false bc did not meet\ncriteria for enough previous \nvalid positions"
            # "Retain Last Valid Position Value"
          }
          frame True {
            w806 = sgl 0.0
            # "Only Calculate MOving Avg\nif xx% of previous positions were valid"
            n395 = for {
              N: 10 -> [_]
              tunnel: w802 -> [w830] mode=indexing
              tunnel: w808 -> [w829] mode=indexing
              tunnel: w807 -> [w828] mode=indexing
              shift-right: [w826] -> w804
              shift-left: w806 -> [w827]
              shift-right: [w824] -> w803
              shift-left: w806 -> [w825]
              # "Calculate Moving Average"
              n396 = case shown="True" w830 {
                tunnel: w829 -> [_ w834]
                tunnel: w828 -> [_ w837]
                tunnel: w827 -> [w832 w838]
                tunnel: [w832 w836] -> w826
                tunnel: w825 -> [w831 w835]
                tunnel: [w831 w833] -> w824
                frame False {
                }
                frame True {
                  n397 = Add(x=w838, y=w837) -> (x+y=w836:sgl)
                  n398 = Add(x=w835, y=w834) -> (x+y=w833:sgl)
                }
              }
            }
            n399 = Divide(x=w804, y=w801) -> (x/y=w796:sgl)
            n400 = Divide(x=w803, y=w801) -> (x/y=w795:sgl)
            n401 = Bundle(w796, w795) -> (w794:cluster{sgl, sgl})  [unwired: 1 in]
            n402 = case shown="True" w798 {
              tunnel: w800 -> [_ w813]
              tunnel: w794 -> [_ w812]
              tunnel: w799 -> [_ w811]
              tunnel: [TRUE w810] -> w797
              frame False {
                # "True bc this position has\nno previous position\nto compare to"
              }
              frame True {
                # "Previous Position"
                # "New (filtered) Position"
                # "Only Check If Close to previous position\nif previous position was valid"
                # "(Y1 - Y2)^2"
                # "(X1 - X2)^2"
                n403 = Unbundle(w813) -> (w821:sgl, w823:sgl)
                n404 = Unbundle(w812) -> (w820:sgl, w822:sgl)
                n405 = Subtract(x=w820, y=w821) -> (x-y=w818:sgl)
                n406 = Subtract(x=w822, y=w823) -> (x-y=w817:sgl)
                n407 = Square(x=w818) -> (x^2=w816:sgl)
                n408 = Square(x=w817) -> (x^2=w815:sgl)
                n409 = Add(x=w816, y=w815) -> (x+y=w819:sgl)
                n410 = Square Root(x=w819) -> (sqrt(x)=w814:sgl)
                n411 = Less?(x=w814, y=w811) -> (x < y?=w810:bool)
              }
            }
          }
        }
        n412 = Replace Array Subset(array=w761, new element=w757, index=w760) -> ()  [unwired: 1 out]
        n413 = Replace Array Subset(array=w759, new element=w758, index=w760) -> ()  [unwired: 1 out]
        n414 = Replace Array Subset(array=w761, new element=w756, index=w760) -> ()  [unwired: 1 out]
        n415 = Replace Array Subset(array=w755, new element=w757, index=w772) -> (w771:dbl[])
        n416 = Replace Array Subset(array=w754, new element=w756, index=w772) -> (w770:dbl[])
        n417 = call "Wait7"("Count(mSec)"=u32 200) -> ()  [unwired: 1 out]
      }
    }
    frame Enabled {
    }
  }
  n418 = disable-structure shown="Enabled" {
    disable-tunnel: [w889 _] -> _
    disable-tunnel: ["Search Step Size\n(deg)" _] -> _
    frame Enabled {
      n419 = Multiply(x=3.413333333333333, y="Search Step Size\n(deg)") -> (x*y=w887:dbl)
      n420 = To Unsigned Word Integer(number=w887) -> (unsigned 16bit integer=w889:u16)
    }
    frame Disabled {
    }
  }
  n421 = Multiply(x="Move Servo\nThreshold (deg)", y=3.413333333333333) -> (x*y=w17:dbl)
  n422 = To Unsigned Word Integer(number=w17) -> ()  [unwired: 1 out]
  n423 = call "Tick Count8"() -> ()  [unwired: 1 out]
  n424 = flat-sequence {
    tunnel: [w893] -> w42
    tunnel: [w892] -> w41
    tunnel: [w897] -> w40
    tunnel: ["Left Servo\nID"] -> w29
    tunnel: ["Right Servo\nID"] -> w28
    tunnel: ["Compliance Slope"] -> w27
    tunnel: [w937] -> w39
    tunnel: [w936] -> w38
    tunnel: w42 -> [w935]
    tunnel: w41 -> [w934]
    tunnel: w40 -> [w933]
    tunnel: w29 -> [w931]
    tunnel: w28 -> [w930]
    tunnel: w27 -> [w929]
    tunnel: w39 -> [w1210]
    tunnel: w38 -> [w1209]
    frame #0 {
      # "BAUD RATE"
      # "Initialize UART and DIO"
      n425 = call-poly "VISA Configure Serial Port"("VISA resource name"=refnum<visa-resource-name> "ASRL1::INSTR", "Enable Termination\nChar (T)"=FALSE ("Enable Termination\nChar (T)"), "baud rate (9600)"=u32 115200) -> ("VISA resource name out"=w893:refnum<visa-resource-name>)  [unwired: 11 in, 1 out]
      n426 = call <vilib>:"Smart Open.vi"("Channel Names"=tag[] ["A/DIO2"]) -> ("DIO Ref Out"=w892:T5)  [unwired: 9 in, 1 out]
      n427 = flat-sequence {
        tunnel: w893 -> [w905]
        tunnel: w892 -> [w904]
        tunnel: "Left Servo\nID" -> [w906]
        tunnel: [w903] -> w894
        tunnel: "Compliance Slope" -> [w902]
        tunnel: "Right Servo\nID" -> [w919]
        tunnel: w894 -> [w918]
        tunnel: "Compliance Slope" -> [w917]
        tunnel: w893 -> [w916]
        tunnel: w892 -> [w915]
        frame #0 {
          w903 = 3
          n428 = while {
            tunnel: w903 -> [w912]
            tunnel: w905 -> [w910]
            tunnel: w904 -> [w909]
            tunnel: w906 -> [w908]
            tunnel: w902 -> [w907]
            i -> [w913]
            stop <- w911 stop-if-true
            n429 = call "Set_Compliance_Slope_R2.vi"("Compliance Slope"=w907, "DIO Ref Out"=w909, "VISA resource name"=w910, "Servo ID"=w908) -> ()  [unwired: 6 in, 2 out]
            n430 = Increment(x=w913) -> (x+1=w914:i32)
            n431 = Greater Or Equal?(x=w914, y=w912) -> (x >= y?=w911:bool)
          }
        }
        frame #1 {
          n432 = while {
            tunnel: w918 -> [w925]
            tunnel: w919 -> [w923]
            tunnel: w916 -> [w922]
            tunnel: w915 -> [w921]
            tunnel: w917 -> [w920]
            i -> [w926]
            stop <- w924 stop-if-true
            n433 = call "Set_Compliance_Slope_R2.vi"("Compliance Slope"=w920, "DIO Ref Out"=w921, "VISA resource name"=w922, "Servo ID"=w923) -> ()  [unwired: 6 in, 2 out]
            n434 = Increment(x=w926) -> (x+1=w927:i32)
            n435 = Greater Or Equal?(x=w927, y=w925) -> (x >= y?=w924:bool)
          }
        }
      }
      n436 = call "Tick Count"() -> ("Tick Count(uSec)"=w897:u32)
    }
    frame #1 {
      # "Service Count"
      n437 = while {
        shift-right: [w940] -> _
        shift-left: w933 -> [w957]
        tunnel: "Max Write\nTx Attempts" -> [w952]
        tunnel: "Max Read\nTx Attempts" -> [w951]
        shift-right: [w947] -> w937
        shift-left: w935 -> [w950]
        shift-right: [w946] -> w936
        shift-left: w934 -> [w949]
        tunnel: w931 -> [w945]
        tunnel: w930 -> [w944]
        tunnel: w929 -> [w943]
        shift-right: [w941] -> _
        shift-left: u16 0 -> [w942]
        stop <- "close comms" stop-if-true
        # "Loop Timer"
        n438 = local read "SERVO ENABLE"() -> (w939:bool)
        n439 = call "Tick Count2"() -> ("Tick Count(uSec)"=w940:u32)
        n440 = Subtract(x=w940, y=w957) -> (x-y=w956:u32)
        n441 = call "Wait4"("Count(mSec)"="Servo Comm\nLoop Time (ms)") -> ()  [unwired: 1 out]
        n442 = Divide(x=w956, y=u32 1000) -> (x/y=→"dT - Comm Loop":dbl)
        n443 = case shown="True" w939 {
          tunnel: w952 -> [_ w966]
          tunnel: w951 -> [_ w997]
          tunnel: w950 -> [w960 w961]
          tunnel: w949 -> [w959 w990]
          tunnel: [w960 w963] -> w947
          tunnel: [w959 w962] -> w946
          tunnel: w945 -> [_ w969]
          tunnel: w944 -> [_ w968]
          tunnel: w943 -> [_ w967]
          tunnel: w942 -> [_ w965]
          tunnel: [u16 100 w964] -> w941
          frame False {
            # "Restart at same value\nUsed to Periodically update \nCompliance Slope"
          }
          frame True {
            n444 = flat-sequence {
              tunnel: [w1003] -> w1001
              tunnel: [w1004] -> w1000
              tunnel: [w1002] -> w999
              tunnel: w997 -> [w1005]
              tunnel: [w1007] -> w988
              tunnel: [w1006] -> w986
              tunnel: w961 -> [w1007]
              tunnel: w990 -> [w1006]
              tunnel: w969 -> [w1002]
              tunnel: w1001 -> [w1025]
              tunnel: w1000 -> [w1026]
              tunnel: w999 -> [w1024]
              tunnel: [w1024] -> w998
              tunnel: [w1023] -> w991
              tunnel: [w1022] -> w989
              tunnel: w988 -> [w1022]
              tunnel: [w1021] -> w987
              tunnel: w986 -> [w1021]
              tunnel: w998 -> [w1047]
              tunnel: w966 -> [w1046]
              tunnel: w991 -> [w1041]
              tunnel: w989 -> [w1043]
              tunnel: w987 -> [w1042]
              tunnel: [w1043] -> w984
              tunnel: [w1042] -> w982
              tunnel: [w1080] -> w985
              tunnel: w984 -> [w1080]
              tunnel: [w1079] -> w983
              tunnel: w982 -> [w1079]
              tunnel: ["Servo Comm\nWait Time - (ms)"] -> w974
              tunnel: w997 -> [w1087]
              tunnel: [w1086] -> w996
              tunnel: [w1085] -> w995
              tunnel: [w1081] -> w993
              tunnel: w985 -> [w1084]
              tunnel: w983 -> [w1083]
              tunnel: [w1084] -> w981
              tunnel: [w1083] -> w978
              tunnel: [w1082] -> w975
              tunnel: w974 -> [w1082]
              tunnel: w968 -> [w1081]
              tunnel: w996 -> [w1107]
              tunnel: w995 -> [w1106]
              tunnel: [w1105] -> w994
              tunnel: w993 -> [w1105]
              tunnel: [w1104] -> w992
              tunnel: w981 -> [w1103]
              tunnel: [w1103] -> w980
              tunnel: [w1102] -> w979
              tunnel: w978 -> [w1102]
              tunnel: w975 -> [w1101]
              tunnel: [w1101] -> w973
              tunnel: w994 -> [w1129]
              tunnel: w992 -> [w1127]
              tunnel: w966 -> [w1128]
              tunnel: w980 -> [w1126]
              tunnel: w979 -> [w1125]
              tunnel: [w1126] -> w977
              tunnel: [w1125] -> w976
              tunnel: w973 -> [w1122]
              tunnel: [w1122] -> w972
              tunnel: w977 -> [w1162]
              tunnel: w976 -> [w1161]
              tunnel: w972 -> [w1160]
              tunnel: [w1162] -> w971
              tunnel: [w1161] -> w970
              tunnel: w971 -> [w1166]
              tunnel: w970 -> [w1165]
              tunnel: w969 -> [w1171]
              tunnel: w968 -> [w1170]
              tunnel: w967 -> [w1169]
              tunnel: w965 -> [w1164]
              tunnel: w966 -> [w1168]
              tunnel: [w1167] -> w964
              tunnel: [w1166] -> w963
              tunnel: [w1165] -> w962
              frame #0 {
                n445 = while {
                  tunnel: [w1020] -> w1003
                  tunnel: w1002 -> [w1019]
                  tunnel: [w1012] -> w1004
                  tunnel: w1005 -> [w1010]
                  tunnel: w1007 -> [w1009]
                  tunnel: w1006 -> [w1008]
                  i -> [w1011]
                  stop <- w1013 stop-if-true
                  # "Attemp to Read Until\nMax Read Tx Attemps Limit"
                  n446 = call "ReadServo_R3.vi"("DIO Ref In"=w1008, "VISA resource name out"=w1009, "Servo ID"=w1019) -> ("Error"=w1016:u8, "Valid Checksum"=w1017:bool, "Current Position"=w1020:u64)  [unwired: 6 in]
                  n447 = Increment(x=w1011) -> (x+1=w1014:i32)
                  n448 = Equal To 0?(x=w1016) -> (x = 0?=w1018:bool)
                  n449 = Greater Or Equal?(x=w1014, y=w1010) -> (x >= y?=w1015:bool)
                  n450 = And(x=w1017, y=w1018) -> (x .and. y?=w1012:bool)
                  n451 = Or(x=w1012, y=w1015) -> (x .or. y?=w1013:bool)
                }
              }
              frame #1 {
                # "Read Position First"
                n452 = local read "Servo Goal Position\n - Left"() -> (w1023:u16)
                n453 = case shown="True" w1026 {
                  tunnel: w1025 -> [_ w1031]
                  tunnel: w1023 -> [_ w1029]
                  frame False {
                  }
                  frame True {
                    # "Convert Received Position to Angle Relative to Robot"
                    # "45 DEG MOUNT OFFSET"
                    # "1024/300"
                    n454 = local write "Current L (10bit)"(w1031) -> ()
                    n455 = To Word Integer(number=w1031) -> (16bit integer=w1035:i16)
                    n456 = To Word Integer(number=w1029) -> (16bit integer=w1034:i16)
                    n457 = Subtract(x=w1034, y=w1035) -> (x-y=w1033:i16)
                    n458 = Divide(x=w1031, y=3.413333333333333) -> (x/y=w1039:dbl)
                    n459 = Absolute Value(x=w1033) -> (abs(x)=w1032:i16)
                    n460 = Subtract(x=w1039, y=sgl 60.0) -> (x-y=w1037:dbl)
                    n461 = Greater?(x=w1032, y=u16 5) -> (0:w1028:bool)
                    n462 = Add(x=w1037, y=sgl 45.0) -> (x+y=w1027:dbl)
                    n463 = local write "Move Servo - L"(w1028) -> ()
                    n464 = local write "Servo Moving - L"(w1028) -> ()
                    n465 = local write "Current Angle\n - Left (internal)"(w1027) -> ()
                    n466 = shared-variable "RT myRIO Target - Overlord\\Localization_Variables_r0.lvlib\\Left Servo Angle_Current"(w1027) -> ()  [unwired: 1 in, 1 out]
                  }
                }
              }
              frame #2 {
                n467 = local read "Move Servo - L"() -> (w1044:bool)
                n468 = case shown="True" w1044 {
                  tunnel: w1047 -> [_ w1062]
                  tunnel: w1041 -> [_ w1049]
                  tunnel: [TRUE w1060] -> w1045
                  tunnel: w1046 -> [_ w1052]
                  tunnel: w1043 -> [_ w1051]
                  tunnel: w1042 -> [_ w1050]
                  frame False {
                    # "Only Send if Current Position is far enough"
                  }
                  frame True {
                    w1058 = 1
                    # "High Byte"
                    # "Low Byte"
                    n469 = Type Cast(type="", x=w1049) -> (*(type *) &x=w1059:string)
                    n470 = local write "Servo Moving - L"(TRUE) -> ()
                    n471 = String Subset(string=w1059, offset (0)=1, length (rest)=w1058) -> (substring=w1054:string)
                    n472 = String Subset(string=w1059, offset (0)=0, length (rest)=w1058) -> (substring=w1053:string)
                    n473 = while {
                      tunnel: w1062 -> [w1076]
                      tunnel: [w1068] -> w1060
                      tunnel: w1054 -> [w1072]
                      tunnel: w1053 -> [w1071]
                      tunnel: w1052 -> [w1065]
                      tunnel: w1051 -> [w1064]
                      tunnel: w1050 -> [w1063]
                      i -> [w1066]
                      stop <- w1067 stop-if-true
                      # "Attemp to Write Until\nMax Write Tx Attemps Limit"
                      n474 = call "MoveServo_R3.vi"("DIO Ref Out"=w1063, "VISA resource name out"=w1064, "GP - Low Byte"=w1072, "GP - High Byte"=w1071, "Servo ID"=w1076) -> ("Valid Checksum"=w1073:bool, "Error"=w1075:u64)  [unwired: 5 in]
                      n475 = Equal To 0?(x=w1075) -> (x = 0?=w1074:bool)
                      n476 = And(x=w1073, y=w1074) -> (x .and. y?=w1068:bool)
                      n477 = Increment(x=w1066) -> (x+1=w1070:i32)
                      n478 = Greater Or Equal?(x=w1070, y=w1065) -> (x >= y?=w1069:bool)
                      n479 = Or(x=w1068, y=w1069) -> (x .or. y?=w1067:bool)
                    }
                  }
                }
                n480 = case shown="True" w1045 {
                  frame False {
                  }
                  frame True {
                    # "Update Servo flag"
                    n481 = local write "Move Servo - L"(FALSE) -> ()
                  }
                }
              }
              frame #3 {
                n482 = call "Wait2"("Count(mSec)"="Servo Comm\nWait Time - (ms)") -> ()  [unwired: 1 out]
              }
              frame #4 {
                n483 = while {
                  tunnel: [w1100] -> w1086
                  tunnel: w1081 -> [w1099]
                  tunnel: [w1092] -> w1085
                  tunnel: w1087 -> [w1090]
                  tunnel: w1084 -> [w1089]
                  tunnel: w1083 -> [w1088]
                  i -> [w1091]
                  stop <- w1093 stop-if-true
                  # "Attemp to Read Until\nMax Read Tx Attemps Limit"
                  n484 = call "ReadServo_R3.vi"("DIO Ref In"=w1088, "VISA resource name out"=w1089, "Servo ID"=w1099) -> ("Error"=w1096:u8, "Valid Checksum"=w1097:bool, "Current Position"=w1100:u64)  [unwired: 6 in]
                  n485 = Increment(x=w1091) -> (x+1=w1094:i32)
                  n486 = Equal To 0?(x=w1096) -> (x = 0?=w1098:bool)
                  n487 = Greater Or Equal?(x=w1094, y=w1090) -> (x >= y?=w1095:bool)
                  n488 = And(x=w1097, y=w1098) -> (x .and. y?=w1092:bool)
                  n489 = Or(x=w1092, y=w1095) -> (x .or. y?=w1093:bool)
                }
              }
              frame #5 {
                n490 = local read "Servo Goal Position\n - Right"() -> (w1104:u16)
                n491 = case shown="True" w1106 {
                  tunnel: w1107 -> [_ w1111]
                  tunnel: w1104 -> [_ w1110]
                  frame False {
                    # "Don't update current position"
                  }
                  frame True {
                    # "Convert Received Position to Angle Relative to Robot"
                    # "45 DEG MOUNT OFFSET"
                    # "1024/300"
                    n492 = local write "Current R (10bit)"(w1111) -> ()
                    n493 = Divide(x=w1111, y=3.413333333333333) -> (x/y=w1120:dbl)
                    n494 = Subtract(x=w1120, y=sgl 60.0) -> (x-y=w1118:dbl)
                    n495 = Subtract(x=w1118, y=sgl 45.0) -> (x-y=w1108:dbl)
                    n496 = To Word Integer(number=w1110) -> (16bit integer=w1115:i16)
                    n497 = To Word Integer(number=w1111) -> (16bit integer=w1116:i16)
                    n498 = shared-variable "RT myRIO Target - Overlord\\Localization_Variables_r0.lvlib\\Right Servo Angle_Current"(w1108) -> ()  [unwired: 1 in, 1 out]
                    n499 = local write "Current Angle\n - Right (internal)"(w1108) -> ()
                    n500 = Subtract(x=w1115, y=w1116) -> (x-y=w1114:i16)
                    n501 = Absolute Value(x=w1114) -> (abs(x)=w1113:i16)
                    n502 = Greater?(x=w1113, y=u16 5) -> (0:w1109:bool)
                    n503 = local write "Move Servo - R"(w1109) -> ()
                    n504 = local write "Servo Moving - R"(w1109) -> ()
                  }
                }
              }
              frame #6 {
                n505 = local read "Move Servo - R"() -> (w1123:bool)
                n506 = case shown="True" w1123 {
                  tunnel: w1127 -> [_ w1132]
                  tunnel: w1129 -> [_ w1139]
                  tunnel: [TRUE w1140] -> w1124
                  tunnel: w1128 -> [_ w1135]
                  tunnel: w1126 -> [_ w1134]
                  tunnel: w1125 -> [_ w1133]
                  frame False {
                  }
                  frame True {
                    w1142 = 1
                    # "High Byte"
                    # "Low Byte"
                    n507 = Type Cast(type="", x=w1132) -> (*(type *) &x=w1141:string)
                    n508 = local write "Servo Moving - R"(TRUE) -> ()
                    n509 = String Subset(string=w1141, offset (0)=1, length (rest)=w1142) -> (substring=w1138:string)
                    n510 = String Subset(string=w1141, offset (0)=0, length (rest)=w1142) -> (substring=w1137:string)
                    n511 = while {
                      tunnel: [w1151] -> w1140
                      tunnel: w1139 -> [w1156]
                      tunnel: w1138 -> [w1155]
                      tunnel: w1137 -> [w1154]
                      tunnel: w1135 -> [w1149]
                      tunnel: w1134 -> [w1147]
                      tunnel: w1133 -> [w1146]
                      i -> [w1150]
                      stop <- w1148 stop-if-true
                      # "Attemp to Write Until\nMax Write Tx Attemps Limit"
                      n512 = call "MoveServo_R3.vi"("DIO Ref Out"=w1146, "VISA resource name out"=w1147, "GP - Low Byte"=w1155, "GP - High Byte"=w1154, "Servo ID"=w1156) -> ("Valid Checksum"=w1158:bool, "Error"=w1157:u64)  [unwired: 5 in]
                      n513 = Increment(x=w1150) -> (x+1=w1152:i32)
                      n514 = Greater Or Equal?(x=w1152, y=w1149) -> (x >= y?=w1153:bool)
                      n515 = Equal To 0?(x=w1157) -> (x = 0?=w1159:bool)
                      n516 = And(x=w1158, y=w1159) -> (x .and. y?=w1151:bool)
                      n517 = Or(x=w1151, y=w1153) -> (x .or. y?=w1148:bool)
                    }
                  }
                }
                n518 = case shown="True" w1124 {
                  frame False {
                  }
                  frame True {
                    # "Update Servo flag"
                    n519 = local write "Move Servo - R"(FALSE) -> ()
                  }
                }
              }
              frame #7 {
                n520 = call "Wait3"("Count(mSec)"=w1160) -> ()  [unwired: 1 out]
              }
              frame #8 {
                # "Increment Service Count"
                # "Update Compliance Slope\nEvery x loops"
                n521 = Equal?(x=w1164, y=u16 1000) -> (x = y?=w1173:bool)
                n522 = case shown="True" w1173 {
                  tunnel: w1169 -> [_ w1183]
                  tunnel: w1166 -> [_ w1182]
                  tunnel: w1165 -> [_ w1181]
                  tunnel: w1166 -> [_ w1180]
                  tunnel: w1165 -> [_ w1179]
                  tunnel: w1171 -> [_ w1178]
                  tunnel: w1170 -> [_ w1177]
                  tunnel: w1164 -> [w1174 _]
                  tunnel: [w1174 u16 0] -> w1172
                  tunnel: w1168 -> [_ w1175]
                  frame False {
                  }
                  frame True {
                    # "Reset Service\nCount"
                    n523 = flat-sequence {
                      tunnel: w1182 -> [w1188]
                      tunnel: w1181 -> [w1187]
                      tunnel: w1178 -> [w1189]
                      tunnel: [w1185] -> w1184
                      tunnel: w1183 -> [w1186]
                      tunnel: w1175 -> [w1185]
                      tunnel: w1177 -> [w1201]
                      tunnel: w1184 -> [w1200]
                      tunnel: w1183 -> [w1199]
                      tunnel: w1180 -> [w1198]
                      tunnel: w1179 -> [w1197]
                      frame #0 {
                        n524 = while {
                          tunnel: w1185 -> [w1196]
                          tunnel: w1188 -> [w1194]
                          tunnel: w1187 -> [w1193]
                          tunnel: w1189 -> [w1192]
                          tunnel: w1186 -> [w1191]
                          i -> [w1190]
                          stop <- w1195 stop-if-true
                          n525 = call "Set_Compliance_Slope_R2.vi"("Compliance Slope"=w1191, "DIO Ref Out"=w1193, "VISA resource name"=w1194, "Servo ID"=w1192) -> ()  [unwired: 6 in, 2 out]
                          n526 = Greater Or Equal?(x=w1190, y=w1196) -> (x >= y?=w1195:bool)
                        }
                      }
                      frame #1 {
                        n527 = while {
                          tunnel: w1200 -> [w1208]
                          tunnel: w1201 -> [w1206]
                          tunnel: w1198 -> [w1205]
                          tunnel: w1197 -> [w1204]
                          tunnel: w1199 -> [w1203]
                          i -> [w1202]
                          stop <- w1207 stop-if-true
                          n528 = call "Set_Compliance_Slope_R2.vi"("Compliance Slope"=w1203, "DIO Ref Out"=w1204, "VISA resource name"=w1205, "Servo ID"=w1206) -> ()  [unwired: 6 in, 2 out]
                          n529 = Greater Or Equal?(x=w1202, y=w1208) -> (x >= y?=w1207:bool)
                        }
                      }
                    }
                  }
                }
                n530 = Increment(x=w1172) -> (x+1=w1167:u16)
              }
            }
          }
        }
      }
    }
    frame #2 {
      n531 = VISA Close(VISA resource name=w1210) -> ()  [unwired: 1 in, 1 out]
      n532 = call <vilib>:"Close.vi"("DIO Ref In"=w1209) -> ()  [unwired: 10 in, 1 out]
    }
  }
  n533 = while {
    stop <- FALSE stop-if-true
    n534 = call "Wait9"("Count(mSec)"=u32 1000) -> ()  [unwired: 1 out]
  }
  n535 = while {
    shift-right: [w1271] -> _
    shift-left: "Initial Main State - Left" -> [w1296]
    shift-right: [w1263] -> _
    shift-left: "Search Direction - in - L" -> [w1290]
    shift-right: [w1262] -> _
    shift-left: FALSE -> [w1289]
    shift-right: [w1265] -> _
    shift-left: w12 -> [w1264]
    shift-right: [w1266] -> _
    shift-left: w12 -> [w1283]
    shift-right: [w1267] -> _
    shift-left: w12 -> [w1288]
    shift-right: [w1268] -> _
    shift-left: w12 -> [w1282]
    shift-right: [w1269] -> _
    shift-left: w12 -> [w1281]
    shift-right: [w1214] -> _
    shift-left: "Search Direction - in - Right" -> [w1238]
    shift-right: [w1259] -> _
    shift-left: FALSE -> [w1236]
    shift-right: [w1260] -> _
    shift-left: w11 -> [w1227]
    shift-right: [w1215] -> _
    shift-left: w11 -> [w1226]
    shift-right: [w1216] -> _
    shift-left: w11 -> [w1233]
    shift-right: [w1217] -> _
    shift-left: w11 -> [w1235]
    shift-right: [w1218] -> _
    shift-left: w11 -> [w1234]
    shift-right: [w1225] -> _
    shift-left: "Initial Main State- Right" -> [w1250]
    shift-right: [w1255] -> _
    shift-left: 0 -> [w1257]
    shift-right: [w1222] -> _
    shift-left: 0 -> [w1242]
    shift-right: [w1254] -> _
    shift-left: "Initial Tracking State - Left" -> [w1256]
    shift-right: [w1220] -> _
    shift-left: "Initial Tracking State - Right" -> [w1248]
    shift-right: [w1221] -> _
    shift-left: "Initial Recovery State  - Right" -> [w1249]
    shift-right: [w1252] -> _
    shift-left: "Initial Recovery State - L" -> [w1253]
    stop <- FALSE stop-if-true
    w1275 = T1."Tracking" ("Next Main State")
    # "Wait for New"
    # "ADD TRACKING TIMEOUT COUNT**********************"
    # "Service Track Angle Flag"
    # "Add Logic to Have Search Directions\nopposite if Both Searching"
    # "REMOVE LAST GOAL POSITION WITH cURRENT"
    # "Go to Current State"
    # "Add Logic to Have Search Directions\nopposite if Both Searching"
    # "Manuallly Reset\nRespond Var"
    # "Manuallly Reset\nRespond Var"
    # "Update Comm Process Variables"
    # "Both Tracking"
    # "Current delta - L"
    # "delta move sum - R"
    # "delta move sum - L"
    # "Current delta - R"
    # "Service Move Respond Variables"
    n536 = local read "Min Num Frames\nper Search"() -> (w1261:i32)
    n537 = local read "Minimum Delta \nServo Threshold"() -> (w1280:i16)
    n538 = local read "Maximum Move \nServo Threshold"() -> (w1279:i16)
    n539 = local read "Middle Beacon\nCoordinates"() -> (w1228:cluster{"X":sgl, "Y":sgl})
    n540 = local read "Position \nLock Status"() -> (w1287:bool)
    n541 = local read "Position \nLock Status"() -> (w1231:bool)
    n542 = local read "Search Step Size"() -> (w1278:u16)
    n543 = local read "Last Orientation"() -> (w1285:sgl)
    n544 = local read "Last Orientation"() -> (w1229:sgl)
    n545 = local read "Last Position"() -> (w1286:cluster{"X":sgl, "Y":sgl})
    n546 = local read "Last Position"() -> (w1230:cluster{"X":sgl, "Y":sgl})
    n547 = local read "Min Num Frames\nper Search"() -> (w1232:i32)
    n548 = call "Wait"("Count(mSec)"="Servo Algorithm\nCycle Time(ms)") -> ()  [unwired: 1 out]
    n549 = local read "Minimum Delta \nServo Threshold"() -> (w1240:i16)
    n550 = local read "Maximum Move \nServo Threshold"() -> (w1239:i16)
    n551 = local read "Search Step Size"() -> (w1237:u16)
    n552 = local read "New Data  Flag\nRight Servo"() -> (w1245:bool)
    n553 = local read "New Data  Flag\nLeft Servo"() -> (w1251:bool)
    n554 = local read "Image Lock - Right"() -> (w1247:bool)
    n555 = local read "Image Lock - Left"() -> (w1295:bool)
    n556 = local read "Tracking Angle - Right"() -> (w1244:sgl)
    n557 = local read "Tracking Angle - Left"() -> (w1293:sgl)
    n558 = local read "Current R (10bit)"() -> (w1243:u16)
    n559 = local read "Current L (10bit)"() -> (w1292:u16)
    n560 = case shown="True" w1245 {
      tunnel: [w1323 w1361] -> w1213
      tunnel: [w1317 w1360] -> w1224
      tunnel: w1250 -> [w1318 w1359]
      tunnel: w1247 -> [_ w1358]
      tunnel: "Track Angle Valid  - R" -> [_ w1357]
      tunnel: w1244 -> [_ w1356]
      tunnel: w1243 -> [w1323 w1355]
      tunnel: "Mounting Offset - Right" -> [_ w1354]
      tunnel: w1238 -> [w1314 w1353]
      tunnel: w1236 -> [_ w1352]
      tunnel: w1233 -> [w1315 w1351]
      tunnel: w1231 -> [_ w1350]
      tunnel: w1230 -> [_ w1349]
      tunnel: w1229 -> [_ w1348]
      tunnel: w1228 -> [_ w1347]
      tunnel: w1226 -> [w1313 w1346]
      tunnel: w1235 -> [w1312 w1345]
      tunnel: w1234 -> [w1316 w1344]
      tunnel: w1240 -> [_ w1343]
      tunnel: w1239 -> [_ w1342]
      tunnel: w1237 -> [_ w1341]
      tunnel: [0 w1340] -> w1223
      tunnel: [w1318 w1339] -> w1225
      tunnel: [w1317 w1338] -> w1219
      tunnel: [w1316 w1337] -> w1218
      tunnel: [w1312 w1336] -> w1217
      tunnel: [w1315 w1335] -> w1216
      tunnel: [w1313 w1334] -> w1215
      tunnel: w1227 -> [_ w1333]
      tunnel: [w1314 w1332] -> w1214
      tunnel: w1232 -> [_ w1331]
      tunnel: w1242 -> [w1321 w1330]
      tunnel: w1248 -> [w1320 w1329]
      tunnel: [w1321 w1328] -> w1222
      tunnel: [w1320 w1327] -> w1220
      tunnel: w1249 -> [w1319 w1326]
      tunnel: [w1319 w1325] -> w1221
      frame False {
        w1317 = FALSE
        # "Recovery Mode COunt"
        # "Frames Processed - L"
        # "Recovery Search move Count - L"
        # "Recovery Search Attempt Count- L"
        # "WAITING FOR NEW IMAGE, RETAIN ALL VALUES"
      }
      frame True {
        w1363 = u16 1023
        w1366 = u16 0
        # "New Tracking State"
        # "Tracking Timeout Count"
        # "Next Main State"
        # "Next Recovery State"
        # "Reset Respond"
        # "Search Direction"
        # "Recovery Count"
        # "Recovery Search move Count"
        # "Recovery Search Attempt Count"
        # "Frames Processed"
        # "Apply Floor/Ceiling to Goal Position"
        # "Current move Delta"
        # "Service Track Angle Flag"
        # "Move Servo"
        # "Goal Position"
        # "Go to Current State"
        n561 = case shown="\"Recovery Mode\"" w1359 {
          tunnel: w1355 -> [w1385 w1462 w1640]
          tunnel: w1356 -> [_ w1464 _]
          tunnel: w1341 -> [w1384 _ w1635]
          tunnel: w1353 -> [w1383 w1444 w1629]
          tunnel: [w1382 w1460 w1639] -> w1367
          tunnel: [w1380 w1461 w1638] -> w1360
          tunnel: w1357 -> [w1378 w1455 w1616]
          tunnel: [w1377 w1457 w1625] -> w1339
          tunnel: w1358 -> [w1376 w1456 w1615]
          tunnel: w1354 -> [_ w1465 w1636]
          tunnel: w1343 -> [_ w1463 _]
          tunnel: [w1370 w1459 w1620] -> w1340
          tunnel: w1342 -> [_ w1458 _]
          tunnel: w1351 -> [w1375 _ w1630]
          tunnel: [enum16{"Generic Sweep", "Recovery Search"}."Recovery Search" enum16{"Generic Sweep", "Recovery Search"}."Recovery Search" w1637] -> w1325
          tunnel: w1346 -> [_ _ w1634]
          tunnel: w1326 -> [_ _ w1617]
          tunnel: w1352 -> [_ w1441 w1646]
          tunnel: w1333 -> [_ w1446 w1641]
          tunnel: w1348 -> [_ w1448 w1643]
          tunnel: w1349 -> [_ w1449 w1644]
          tunnel: w1350 -> [_ w1450 w1645]
          tunnel: w1347 -> [_ w1447 w1642]
          tunnel: [FALSE w1443 w1618] -> w1338
          tunnel: w1331 -> [w1374 _ w1628]
          tunnel: [w1370 w1438 w1627] -> w1334
          tunnel: [w1370 w1438 w1633] -> w1337
          tunnel: [w1370 w1438 w1632] -> w1336
          tunnel: [w1373 w1439 w1631] -> w1335
          tunnel: w1345 -> [_ _ w1623]
          tunnel: w1344 -> [_ _ w1622]
          tunnel: [w1371 w1444 w1621] -> w1332
          tunnel: w1330 -> [_ w1454 _]
          tunnel: [w1370 w1445 w1620] -> w1328
          tunnel: w1329 -> [_ w1451 _]
          tunnel: [enum16{"Track", "Reactive Predict", ""}."Track" ("Initial Tracking State - Right") w1442 enum16{"Track", "Reactive Predict", ""}."Track" ("Initial Tracking State - Right")] -> w1327
          frame "Start Up Search", Default {
            w1370 = u16 0
            # "Search Direction"
            # "Wait for 'x' Images to be Processed\nBefore Going to Next Step"
            # "Next Main State"
            # "New Goal Position"
            # "Move Servo"
            # "Choose Next State"
            # "Frames Processed Count"
            n562 = Greater Or Equal?(x=w1375, y=w1374) -> (x >= y?=w1381:bool)
            n563 = case shown="True" w1381 {
              tunnel: w1385 -> [w1400 w1412]
              tunnel: w1384 -> [_ w1410]
              tunnel: w1383 -> [w1399 w1409]
              tunnel: [w1400 w1406] -> w1382
              tunnel: [w1398 0] -> w1373
              tunnel: [FALSE TRUE] -> w1379
              tunnel: w1375 -> [w1401 _]
              tunnel: [w1399 w1403] -> w1371
              frame False {
                # "Increase Frames\nProcessed Count"
                n564 = Increment(x=w1401) -> (x+1=w1398:i32)
              }
              frame True {
                # "Reset Frames\nProcessed Count"
                # "SWEEP SEARCH - Startup"
                # "Multiple New Step\nby Step SIze"
                # "F = CCW\nT = CW"
                # "Last Direction"
                # "Min Step"
                # "add 10 in case\nactual position\nis lower than GP"
                # "Set New Step #"
                # "Choose Direction"
                # "Nearest step"
                # "Adjust Actual Posiiton\n to pre-determiend steps"
                # "Move Servo 1 \"Step\" to\nSearch"
                n565 = Add(x=3, y=w1412) -> (x+y=w1418:i32)
                n566 = Quotient & Remainder(x=w1418, y=w1410) -> (floor(x/y)=w1416:i32)  [unwired: 1 out]
                n567 = To Byte Integer(number=w1416) -> (8bit integer=w1407:i8)
                n568 = Less?(x=w1407, y=1) -> (x < y?=w1413:bool)
                n569 = case shown="False" w1413 {
                  tunnel: w1407 -> [w1429 w1437]
                  tunnel: [w1431 FALSE] -> w1403
                  tunnel: [w1430 w1437] -> w1415
                  tunnel: w1409 -> [w1428 _]
                  tunnel: w1410 -> [w1426 _]
                  frame False {
                    # "Max Step"
                    # "# of steps\nminus 1"
                    n570 = Divide(x=1024, y=w1426) -> (x/y=w1423:dbl)
                    n571 = To Unsigned Byte Integer(number=w1423) -> (unsigned 8bit integer=w1424:u8)
                    n572 = Greater Or Equal?(x=w1429, y=w1424) -> (x >= y?=w1425:bool)
                    n573 = case shown="True" w1425 {
                      tunnel: [w1432 TRUE] -> w1431
                      tunnel: [w1433 w1434] -> w1430
                      tunnel: w1429 -> [w1433 w1434]
                      tunnel: w1428 -> [w1432 _]
                      frame False {
                        # "No Need to\nChange Direction"
                      }
                      frame True {
                        # "T"
                        # "Move CW"
                      }
                    }
                  }
                  frame True {
                    # "F"
                    # "Move CCW"
                  }
                }
                n574 = case shown="False" w1403 {
                  tunnel: w1415 -> [w1420 w1421]
                  tunnel: [w1419 w1422] -> w1411
                  frame False {
                    # "CCW\n+1"
                    n575 = Increment(x=w1420) -> (x+1=w1419:i8)
                  }
                  frame True {
                    # "CW\n-1"
                    n576 = Decrement(x=w1421) -> (x-1=w1422:i8)
                  }
                }
                n577 = Multiply(x=w1411, y=w1410) -> (x*y=w1408:u16)
                n578 = To Unsigned Word Integer(number=w1408) -> (unsigned 16bit integer=w1406:u16)
              }
            }
            n579 = case shown="False" w1378 {
              tunnel: [w1389 FALSE] -> w1380
              tunnel: w1379 -> [w1389 _]
              tunnel: [w1390 w1395] -> w1377
              tunnel: w1376 -> [_ w1393]
              frame False {
                # "Check other Servo\nStay in Startup  State"
                n580 = local read "Track Angle Valid - Left"() -> (w1386:bool)
                n581 = local read "Image Lock - Left"() -> (w1387:bool)
                n582 = Or(x=w1386, y=w1387) -> (x .or. y?=w1388:bool)
                n583 = case shown="True" w1388 {
                  tunnel: [T1."Start Up Search" ("Next Main State") T1."Recovery Mode" ("Next Main State")] -> w1390
                  frame False {
                  }
                  frame True {
                  }
                }
              }
              frame True {
                # "Override Move Servo\nCommand bc an Angle Was Found\nduring this Step"
                # "Transition to Tracking State When\nImage Processing has Locked"
                n584 = case shown="False" w1393 {
                  tunnel: [T1."Start Up Search" ("Next Main State") T1."Tracking" ("Next Main State")] -> w1395
                  frame False {
                  }
                  frame True {
                  }
                }
              }
            }
          }
          frame "Tracking" {
            w1438 = 0
            # "Frames Processed Count"
            # "Image Lock - L"
            # "Track Angle Valid"
            # "Tracking Angle"
            # "Tracking Timeout Count"
            # "Max ove delta"
            # "Move delta threshold"
            # "mount offset"
            # "Current Position"
            # "Move Respond"
            # "Trackin Timeout count"
            # "Move Servo"
            # "delta"
            # "GP"
            # "Reset Move Respond"
            # "New Tracking State"
            # "Delta Move Sum"
            # "Choose Next State"
            n585 = case shown="\"Reactive Predict\"" w1451 {
              tunnel: w1465 -> [w1483 _]
              tunnel: w1464 -> [w1482 _]
              tunnel: w1463 -> [w1481 _]
              tunnel: w1462 -> [w1480 w1538]
              tunnel: [w1479 w1536] -> w1461
              tunnel: [w1478 w1544] -> w1460
              tunnel: [w1477 0] -> w1459
              tunnel: w1458 -> [w1476 _]
              tunnel: w1456 -> [w1475 w1528]
              tunnel: w1455 -> [w1474 w1531]
              tunnel: w1454 -> [w1473 w1533]
              tunnel: w1450 -> [_ w1543]
              tunnel: w1449 -> [_ w1542]
              tunnel: w1448 -> [_ w1541]
              tunnel: w1447 -> [_ w1540]
              tunnel: w1441 -> [_ w1539]
              tunnel: w1446 -> [_ w1537]
              tunnel: [TRUE w1534] -> w1443
              tunnel: [w1470 w1532] -> w1445
              tunnel: [w1468 w1530] -> w1442
              tunnel: [0 0] -> w1439
              frame "Track", Default {
                # "Reset"
                # "Tracking Timeout"
                # "Move Delta"
                # "Goal Position"
                # "Tracking Move"
                # "Move Servo"
                # "Only Consider Tracking Angle\n\nIF\n\nImage Locked        == T\nTrack Angle Flag   == T"
                n586 = And(x=w1475, y=w1474) -> (x .and. y?=w1467:bool)
                n587 = case shown="True" w1467 {
                  tunnel: w1483 -> [_ w1489]
                  tunnel: w1482 -> [_ w1507]
                  tunnel: w1481 -> [_ w1504]
                  tunnel: w1480 -> [w1486 w1494]
                  tunnel: [w1486 w1503] -> w1478
                  tunnel: [w1488 w1502] -> w1479
                  tunnel: [w1488 w1501] -> _
                  tunnel: [u16 0 w1500] -> w1477
                  tunnel: w1476 -> [_ w1496]
                  tunnel: w1473 -> [w1485 _]
                  tunnel: [w1484 0] -> w1470
                  frame False {
                    w1488 = FALSE
                    # "Increment timeout"
                    n588 = Increment(x=w1485) -> (x+1=w1484:i32)
                  }
                  frame True {
                    # "Convert Track Angle to UINT16"
                    # "1024/300"
                    # "Move to Tracking Angle \n\nif delta is greater than move servo threshold\nAND less than max move threshold"
                    n589 = Add(x=w1507, y=w1489) -> (x+y=w1510:sgl)
                    n590 = Add(x=w1510, y=sgl 60.0) -> (x+y=w1509:sgl)
                    n591 = Multiply(x=3.413333333333333, y=w1509) -> (x*y=w1490:dbl)
                    n592 = To Word Integer(number=w1494) -> (16bit integer=w1492:i16)
                    n593 = To Unsigned Word Integer(number=w1490) -> (unsigned 16bit integer=w1506:u16)
                    n594 = To Word Integer(number=w1490) -> (16bit integer=w1505:i16)
                    n595 = Subtract(x=w1505, y=w1492) -> (x-y=w1495:i16)
                    n596 = Absolute Value(x=w1495) -> (abs(x)=w1491:i16)
                    n597 = Greater Or Equal?(x=w1491, y=w1504) -> (x >= y?=w1498:bool)
                    n598 = Less Or Equal?(x=w1491, y=w1496) -> (x <= y?=w1497:bool)
                    n599 = And(x=w1498, y=w1497) -> (x .and. y?=w1499:bool)
                    n600 = case shown="True" w1499 {
                      tunnel: w1506 -> [_ w1518]
                      tunnel: [w1513 w1518] -> w1503
                      tunnel: [w1514 w1524] -> w1502
                      tunnel: [w1514 w1524] -> w1501
                      tunnel: w1494 -> [w1513 _]
                      tunnel: w1491 -> [_ w1523]
                      tunnel: [u16 0 w1523] -> w1500
                      tunnel: w1489 -> [_ w1517]
                      frame False {
                        w1514 = FALSE
                        # "Don't Move"
                      }
                      frame True {
                        w1524 = TRUE
                        # "45 DEG MOUNT OFFSET"
                        # "1024/300"
                        # "Current Delta"
                        # "Use new Track Angle"
                        n601 = Divide(x=w1518, y=3.413333333333333) -> (x/y=w1520:dbl)
                        n602 = Negate(x=w1517) -> (-x=w1516:sgl)
                        n603 = Subtract(x=w1520, y=sgl 60.0) -> (x-y=w1522:dbl)
                        n604 = Add(x=w1522, y=w1516) -> (x+y=w1515:dbl)
                        n605 = local write "Last Track Angle - R"(w1515) -> ()
                      }
                    }
                  }
                }
                n606 = local read "Timeout to \nEnable Reactive Predict"() -> (w1471:u16)
                n607 = Less?(x=w1470, y=w1471) -> (x < y?=w1469:bool)
                n608 = case shown="False" w1469 {
                  tunnel: [enum16{"Track", "Reactive Predict", ""}."Reactive Predict" ("Initial Tracking State - Right") enum16{"Track", "Reactive Predict", ""}."Track" ("Initial Tracking State - Right")] -> w1468
                  frame False {
                  }
                  frame True {
                  }
                }
              }
              frame "Reactive Predict" {
                # "Choose New\nTracking State"
                n609 = Or(x=w1528, y=w1531) -> (x .or. y?=w1527:bool)
                n610 = case shown="False" w1527 {
                  tunnel: [w1557 w1609] -> w1544
                  tunnel: w1543 -> [w1556 _]
                  tunnel: w1542 -> [w1555 _]
                  tunnel: w1541 -> [w1554 _]
                  tunnel: w1540 -> [w1553 _]
                  tunnel: w1539 -> [w1552 _]
                  tunnel: w1537 -> [w1551 _]
                  tunnel: [w1550 w1608] -> w1536
                  tunnel: [w1549 w1608] -> w1534
                  tunnel: w1533 -> [w1548 _]
                  tunnel: [w1547 0] -> w1532
                  tunnel: [enum16{"Track", "Reactive Predict", ""}."Reactive Predict" ("Initial Tracking State - Right") enum16{"Track", "Reactive Predict", ""}."Track" ("Initial Tracking State - Right")] -> w1530
                  tunnel: w1538 -> [w1545 w1609]
                  frame False {
                    # "Stay in Reactive State"
                    # "Increment Track Timeout"
                    # "Move Respond Flag"
                    n611 = Increment(x=w1548) -> (x+1=w1547:i32)
                    n612 = case shown="True" w1552 {
                      tunnel: w1556 -> [_ w1572]
                      tunnel: w1555 -> [_ w1571]
                      tunnel: w1554 -> [_ w1570]
                      tunnel: w1553 -> [_ w1569]
                      tunnel: w1551 -> [_ w1566]
                      tunnel: [w1558 w1562] -> w1557
                      tunnel: [w1559 w1561] -> w1550
                      tunnel: [w1559 w1561] -> w1549
                      tunnel: w1545 -> [w1558 w1560]
                      frame False {
                        w1559 = FALSE
                        # "Reset Move Respond = F"
                        # "Move Servo = F"
                      }
                      frame True {
                        w1561 = TRUE
                        # "Position Lock"
                        # "Current Servo\nPosition"
                        # "Reset Move\nRespond = T"
                        # "Move Servo = T"
                        # "Apply Direction \nto Offset (delta sum)"
                        # "Check Last Known Position of Robot"
                        n613 = case shown="True" w1572 {
                          tunnel: w1571 -> [_ w1600]
                          tunnel: w1570 -> [_ w1575]
                          tunnel: w1569 -> [_ w1576]
                          tunnel: [sgl 1.0 ("y") w1574] -> w1568
                          frame False {
                            # "No Position Data Available"
                            # "Default is to move\nSame Direction as other\nServo"
                          }
                          frame True {
                            w1581 = sgl 1.0 ("y")
                            # "Use previous position/orientation to Guess Which Direction to Move Servo"
                            # "Choose Search Direction"
                            # "\"Perpendicular \nThreshold\""
                            # "If Orientation is\n ~Perpendicular -> Start Search\n in Opposite Direction of Other"
                            # "****add 90 until orientation angle is fixed"
                            # "Last Orientation"
                            # "Convert to Rad"
                            # "Avoid Divide by 0"
                            # "-1/m"
                            # "Calculate Normal Line to \nLast Robot Position\nfrom Center Beacon"
                            # "last Position \nCoordinates"
                            n614 = Unbundle(w1600) -> ("X"=w1580:sgl, "Y"=w1579:sgl)
                            n615 = Unbundle(w1576) -> ("X"=w1578:sgl, "Y"=w1577:sgl)
                            n616 = Subtract(x=w1579, y=w1577) -> (x-y=w1596:sgl)
                            n617 = Subtract(x=w1580, y=w1578) -> (x-y=w1594:sgl)
                            n618 = Equal To 0?(x=w1594) -> (x = 0?=w1595:bool)
                            n619 = case shown="False" w1595 {
                              tunnel: w1596 -> [w1603 _]
                              tunnel: w1594 -> [w1602 _]
                              tunnel: [w1601 1000000000000000.0] -> w1593
                              frame False {
                                n620 = Divide(x=w1603, y=w1602) -> (x/y=w1601:sgl)
                              }
                              frame True {
                              }
                            }
                            n621 = Equal To 0?(x=w1593) -> (x = 0?=w1598:bool)
                            n622 = case shown="False" w1598 {
                              tunnel: [w1605 1e-08] -> w1597
                              tunnel: w1593 -> [w1605 _]
                              frame False {
                              }
                              frame True {
                                # "Can't have infinit slope"
                              }
                            }
                            n623 = Divide(x=-1.0, y=w1597) -> (x/y=w1592:dbl)
                            n624 = Inverse Tangent(1:w1592) -> (0:w1590:dbl)
                            n625 = expression code="(x/pi)*180.0" "radians to degrees"(w1590) -> (w1591:dbl)
                            n626 = To Single Precision Float(number=w1591) -> (single precision float=w1588:sgl)
                            n627 = Add(x=w1575, y=sgl 90.0) -> (x+y=w1587:sgl)
                            n628 = Subtract(x=w1588, y=w1587) -> (x-y=w1586:sgl)
                            n629 = Absolute Value(x=w1586) -> (abs(x)=w1585:sgl)
                            n630 = Less Or Equal?(x=w1585, y=sgl 10.0) -> (x <= y?=w1583:bool)
                            n631 = Negate(x=w1581) -> (-x=w1582:sgl)
                            n632 = Select(t=w1582, s=w1583, f=w1581) -> (s? t:f=w1574:sgl)
                          }
                        }
                        n633 = To Word Integer(number=w1568) -> (16bit integer=w1567:i16)
                        n634 = Multiply(x=w1567, y=w1566) -> (x*y=w1565:i32)
                        n635 = To Word Integer(number=w1560) -> (16bit integer=w1564:i16)
                        n636 = Add(x=w1565, y=w1564) -> (x+y=w1563:i32)
                        n637 = To Unsigned Word Integer(number=w1563) -> (unsigned 16bit integer=w1562:u16)
                      }
                    }
                  }
                  frame True {
                    w1608 = TRUE
                    # "Go Directly to Track State"
                  }
                }
              }
            }
            n638 = local read "Tracking Timeout\nThreshold"() -> (w1452:i32)
            n639 = Less?(x=w1445, y=w1452) -> (x < y?=w1453:bool)
            n640 = case shown="False" w1453 {
              tunnel: [T1."Recovery Mode" ("Next Main State") T1."Tracking" ("Next Main State")] -> w1457
              frame False {
              }
              frame True {
              }
            }
          }
          frame "Recovery Mode" {
            w1620 = u16 0
            # "Increment Recovery Mode Count"
            # "Recovvery Mode\nCount"
            # "Frames Processed"
            # "Choose Next Main State"
            # "Reset recovery count"
            # "Recovery move\nCount"
            # "Recovery Search\nAttempt count"
            # "Move Servo = T"
            # "delta move sum"
            # "Robot Position Valid"
            n641 = local read "Image Lock - Left"() -> (w1624:bool)
            n642 = Or(x=w1615, y=w1616) -> (x .or. y?=w1614:bool)
            n643 = case shown="\"Generic Sweep\"" w1617 {
              tunnel: w1646 -> [_ _]
              tunnel: w1645 -> [_ _]
              tunnel: w1644 -> [_ _]
              tunnel: w1643 -> [_ _]
              tunnel: w1642 -> [_ _]
              tunnel: w1641 -> [_ _]
              tunnel: w1640 -> [w1674 w1760]
              tunnel: [w1666 w1758] -> w1639
              tunnel: [w1663 w1752] -> w1638
              tunnel: [FALSE FALSE] -> w1618
              tunnel: [w1668 w1749] -> w1637
              tunnel: w1634 -> [w1672 _]
              tunnel: w1636 -> [w1675 _]
              tunnel: w1635 -> [w1673 w1755]
              tunnel: [w1665 w1748] -> w1632
              tunnel: [w1664 w1748] -> w1633
              tunnel: w1624 -> [w1662 _]
              tunnel: [w1653 w1759] -> w1631
              tunnel: w1630 -> [w1651 w1743]
              tunnel: w1629 -> [w1656 w1756]
              tunnel: w1628 -> [w1652 w1754]
              tunnel: w1615 -> [_ _]
              tunnel: w1616 -> [_ w1751]
              tunnel: [FALSE w1750] -> w1626
              tunnel: w1623 -> [w1660 _]
              tunnel: w1622 -> [w1659 _]
              tunnel: [w1656 w1747] -> w1621
              frame "Recovery Search" {
                # "Wait for 2 Images to be Processed\nBefore Going to Next Step"
                # "Choose Next Reovery State"
                # "Recovery Search \nAttempt Count"
                # "Move Servo"
                # "Goal Position"
                # "Recovery Search\nmove Count"
                # "Attempt Recovery Search if Other Servo has Valid Angle"
                n644 = local read "Last Track Angle - L"() -> (w1655:sgl)
                n645 = Greater Or Equal?(x=w1651, y=w1652) -> (x >= y?=w1654:bool)
                n646 = case shown="True" w1654 {
                  tunnel: w1675 -> [_ w1695]
                  tunnel: [w1680 w1694] -> w1664
                  tunnel: w1674 -> [w1683 w1693]
                  tunnel: w1673 -> [_ w1692]
                  tunnel: [w1681 w1691] -> w1665
                  tunnel: [w1683 w1690] -> w1666
                  tunnel: [FALSE w1689] -> w1663
                  tunnel: w1660 -> [w1681 w1688]
                  tunnel: w1659 -> [w1680 w1687]
                  tunnel: w1662 -> [_ w1686]
                  tunnel: w1655 -> [_ w1685]
                  tunnel: [w1678 0 ("Frames Processed\nCount - in")] -> w1653
                  tunnel: w1651 -> [w1679 _]
                  frame False {
                    # "Increment Frames Processed"
                    # "WAIT"
                    n647 = Increment(x=w1679) -> (x+1=w1678:i32)
                  }
                  frame True {
                    n648 = case shown="True" w1686 {
                      tunnel: w1685 -> [_ w1708]
                      tunnel: w1688 -> [w1696 w1704]
                      tunnel: w1695 -> [_ w1709]
                      tunnel: [w1699 w1707] -> w1690
                      tunnel: [w1697 w1706] -> w1694
                      tunnel: w1687 -> [w1697 w1705]
                      tunnel: w1693 -> [w1699 w1703]
                      tunnel: w1692 -> [_ w1702]
                      tunnel: [FALSE TRUE] -> w1689
                      tunnel: [w1696 w1700] -> w1691
                      frame False {
                        # "Don't Move bc Other Servo Doesn't Have Image Lock"
                      }
                      frame True {
                        # "Move Servo = T"
                        n649 = Greater Than 0?(x=w1704) -> (x > 0?=w1710:bool)
                        n650 = case shown="False" w1710 {
                          tunnel: w1709 -> [w1717 _]
                          tunnel: w1708 -> [w1711 _]
                          tunnel: [w1716 w1727] -> w1707
                          tunnel: [w1714 w1733] -> w1706
                          tunnel: w1705 -> [w1715 w1733]
                          tunnel: w1704 -> [w1713 w1730]
                          tunnel: [w1712 w1732] -> w1700
                          tunnel: w1703 -> [_ w1728]
                          tunnel: w1702 -> [_ w1725]
                          frame False {
                            # "Increment move count to transition\nto Pan mode"
                            # "Increment Recovery Search Attempt Count"
                            # "1024/300"
                            # "Move Parallel to Other Servo"
                            n651 = Increment(x=w1715) -> (x+1=w1714:i32)
                            n652 = Add(x=w1711, y=w1717) -> (x+y=w1723:sgl)
                            n653 = Add(x=w1723, y=sgl 60.0) -> (x+y=w1722:sgl)
                            n654 = Multiply(x=3.413333333333333, y=w1722) -> (x*y=w1720:dbl)
                            n655 = Add(x=0.5, y=w1720) -> (x+y=w1718:dbl)
                            n656 = To Unsigned Word Integer(number=w1718) -> (unsigned 16bit integer=w1716:u16)
                            n657 = Increment(x=w1713) -> (x+1=w1712:i32)
                          }
                          frame True {
                            # "Apply Direction"
                            # "Step SIze"
                            # "Current Position"
                            # "Attempt to Pan in Steps Towards other Servo"
                            # "Could be same or function of \nregular search step size"
                            # "Max # of Pan\nMoves"
                            # "Pan Towards Other Servo"
                            n658 = Greater Or Equal?(x=w1730, y=u16 20) -> (x >= y?=w1731:bool)
                            n659 = case shown="False" w1731 {
                              tunnel: w1730 -> [w1741 _]
                              tunnel: [w1740 u16 0] -> w1732
                              frame False {
                                # "Increment Pan Count"
                                n660 = Increment(x=w1741) -> (x+1=w1740:i32)
                              }
                              frame True {
                                # "Reset move count"
                              }
                            }
                            n661 = local read "Recovery Search\nDirection - R"() -> (w1726:bool)
                            n662 = case shown="False" w1726 {
                              tunnel: w1728 -> [w1735 w1739]
                              tunnel: w1725 -> [w1736 w1738]
                              tunnel: [w1734 w1737] -> w1727
                              frame False {
                                # "CCW"
                                n663 = Add(x=w1735, y=w1736) -> (x+y=w1734:u16)
                              }
                              frame True {
                                # "CW"
                                n664 = Subtract(x=w1739, y=w1738) -> (x-y=w1737:u16)
                              }
                            }
                          }
                        }
                      }
                    }
                  }
                }
                n665 = local read "Max Recovery Count\n(Recovery Search)"() -> (w1657:u16)
                n666 = local read "Max Recovery\nSearch Attempts"() -> (w1658:u16)
                n667 = Less Or Equal?(x=w1664, y=w1658) -> (x <= y?=w1670:bool)
                n668 = Less Or Equal?(x=w1672, y=w1657) -> (x <= y?=w1671:bool)
                n669 = And(x=w1670, y=w1671) -> (x .and. y?=w1669:bool)
                n670 = case shown="True" w1669 {
                  tunnel: [enum16{"Generic Sweep", "Recovery Search"}."Generic Sweep" enum16{"Generic Sweep", "Recovery Search"}."Recovery Search"] -> w1668
                  frame False {
                  }
                  frame True {
                  }
                }
              }
              frame "Generic Sweep" {
                w1748 = u16 0
                # "Angle Valid?"
                # "Choose Next Recovery State"
                # "Wait for 2 Images to be Processed\nBefore Going to Next Step"
                # "New Goal Position"
                # "Move Servo"
                # "Frames Processed Count"
                n671 = Greater Or Equal?(x=w1743, y=w1754) -> (x >= y?=w1761:bool)
                n672 = case shown="True" w1761 {
                  tunnel: w1760 -> [w1777 w1789]
                  tunnel: w1755 -> [_ w1787]
                  tunnel: w1756 -> [w1776 w1786]
                  tunnel: [w1777 w1783] -> w1758
                  tunnel: [w1775 0] -> w1759
                  tunnel: [FALSE TRUE] -> w1753
                  tunnel: w1743 -> [w1778 _]
                  tunnel: [w1776 w1780] -> w1747
                  frame False {
                    # "Increment Frames Processed"
                    n673 = Increment(x=w1778) -> (x+1=w1775:i32)
                  }
                  frame True {
                    # "Reset Frames\nProcessed Count"
                    # "SWEEP SEARCH - Startup"
                    # "Multiple New Step\nby Step SIze"
                    # "F = CCW\nT = CW"
                    # "Last Direction"
                    # "Min Step"
                    # "add 10 in case\nactual position\nis lower than GP"
                    # "Set New Step #"
                    # "Choose Direction"
                    # "Nearest step"
                    # "Adjust Actual Posiiton\n to pre-determiend steps"
                    # "Move Servo 1 \"Step\" to\nSearch"
                    n674 = Add(x=5, y=w1789) -> (x+y=w1795:i32)
                    n675 = Quotient & Remainder(x=w1795, y=w1787) -> (floor(x/y)=w1793:i32)  [unwired: 1 out]
                    n676 = To Byte Integer(number=w1793) -> (8bit integer=w1784:i8)
                    n677 = Less?(x=w1784, y=1) -> (x < y?=w1790:bool)
                    n678 = case shown="False" w1790 {
                      tunnel: w1784 -> [w1806 w1814]
                      tunnel: [w1808 FALSE] -> w1780
                      tunnel: [w1807 w1814] -> w1792
                      tunnel: w1786 -> [w1805 _]
                      tunnel: w1787 -> [w1803 _]
                      frame False {
                        # "Max Step"
                        # "# of steps\nminus 1"
                        n679 = Divide(x=1024, y=w1803) -> (x/y=w1800:dbl)
                        n680 = To Unsigned Byte Integer(number=w1800) -> (unsigned 8bit integer=w1801:u8)
                        n681 = Greater Or Equal?(x=w1806, y=w1801) -> (x >= y?=w1802:bool)
                        n682 = case shown="True" w1802 {
                          tunnel: [w1809 TRUE] -> w1808
                          tunnel: [w1810 w1811] -> w1807
                          tunnel: w1806 -> [w1810 w1811]
                          tunnel: w1805 -> [w1809 _]
                          frame False {
                            # "No Need to\nChange Direction"
                          }
                          frame True {
                            # "T"
                            # "Move CW"
                          }
                        }
                      }
                      frame True {
                        # "F"
                        # "Move CCW"
                      }
                    }
                    n683 = case shown="True" w1780 {
                      tunnel: w1792 -> [w1797 w1798]
                      tunnel: [w1796 w1799] -> w1788
                      frame False {
                        # "CCW\n+1"
                        n684 = Increment(x=w1797) -> (x+1=w1796:i8)
                      }
                      frame True {
                        # "CW\n-1"
                        n685 = Decrement(x=w1798) -> (x-1=w1799:i8)
                      }
                    }
                    n686 = Multiply(x=w1788, y=w1787) -> (x*y=w1785:u16)
                    n687 = To Unsigned Word Integer(number=w1785) -> (unsigned 16bit integer=w1783:u16)
                  }
                }
                n688 = local read "Track Angle Valid - Left"() -> (w1746:bool)
                n689 = local read "Image Lock - Left"() -> (w1745:bool)
                n690 = Or(x=w1745, y=w1746) -> (x .or. y?=w1744:bool)
                n691 = case shown="False" w1751 {
                  tunnel: [w1764 w1774] -> w1752
                  tunnel: w1753 -> [w1765 _]
                  tunnel: [w1766 enum16{"Generic Sweep", "Recovery Search"}."Generic Sweep"] -> w1749
                  tunnel: [w1763 w1774] -> w1750
                  tunnel: w1744 -> [w1762 _]
                  frame False {
                    # "Is other servo tracking?"
                    n692 = case shown="True" w1762 {
                      tunnel: [enum16{"Generic Sweep", "Recovery Search"}."Generic Sweep" enum16{"Generic Sweep", "Recovery Search"}."Recovery Search"] -> w1766
                      tunnel: w1765 -> [w1769 _]
                      tunnel: [w1769 FALSE] -> w1764
                      tunnel: [FALSE TRUE] -> w1763
                      frame False {
                        # "Stay in Sweep"
                      }
                      frame True {
                        # "G o to Recovery Search  State"
                      }
                    }
                  }
                  frame True {
                    w1774 = FALSE
                    # "Override Move Servo\nCommand bc an Angle Was Found\nduring this Step"
                    # "Stay In Sweep\nLet Main State Machine transition\ninto Tracking"
                  }
                }
              }
            }
            n693 = Increment(x=w1634) -> (x+1=w1613:i32)
            n694 = case shown="True" w1626 {
              tunnel: w1613 -> [w1649 _]
              tunnel: [w1649 0] -> w1627
              frame False {
              }
              frame True {
              }
            }
            n695 = case shown="False" w1614 {
              tunnel: [T1."Recovery Mode" ("Next Main State") T1."Tracking" ("Next Main State")] -> w1625
              frame False {
              }
              frame True {
              }
            }
          }
        }
        "Current Move Delta - L 2" <- w1340
        n696 = Less?(x=w1367, y=w1366) -> (x < y?=w1365:bool)
        n697 = local write "New Data  Flag\nRight Servo"(FALSE) -> ()
        n698 = Select(t=w1366, s=w1365, f=w1367) -> (s? t:f=w1362:u16)
        n699 = Greater?(x=w1362, y=w1363) -> (0:w1364:bool)
        n700 = Select(t=w1363, s=w1364, f=w1362) -> (s? t:f=w1361:u16)
      }
    }
    "Next Main State - Right" <- w1225
    "Next Tracking State - Right" <- w1220
    "Next Recovery State - Right" <- w1221
    n701 = case shown="True" w1251 {
      tunnel: [w1826 w1864] -> w1298
      tunnel: [w1820 w1863] -> w1297
      tunnel: w1296 -> [w1821 w1862]
      tunnel: w1295 -> [_ w1861]
      tunnel: "Track Angle Valid - Left" -> [_ w1860]
      tunnel: w1293 -> [_ w1859]
      tunnel: w1292 -> [w1826 w1858]
      tunnel: "Mounting Offset - Left" -> [_ w1857]
      tunnel: w1290 -> [w1817 w1856]
      tunnel: w1289 -> [_ w1855]
      tunnel: w1288 -> [w1818 w1854]
      tunnel: w1287 -> [_ w1853]
      tunnel: w1286 -> [_ w1852]
      tunnel: w1285 -> [_ w1851]
      tunnel: "Middle Beacon\nCoordinates" -> [_ w1850]
      tunnel: w1283 -> [w1816 w1849]
      tunnel: w1282 -> [w1815 w1848]
      tunnel: w1281 -> [w1819 w1847]
      tunnel: w1280 -> [_ w1846]
      tunnel: w1279 -> [_ w1845]
      tunnel: w1278 -> [_ w1844]
      tunnel: [0 w1843] -> w1272
      tunnel: [w1821 w1842] -> w1271
      tunnel: [w1820 w1841] -> w1270
      tunnel: [w1819 w1840] -> w1269
      tunnel: [w1815 w1839] -> w1268
      tunnel: [w1818 w1838] -> w1267
      tunnel: [w1816 w1837] -> w1266
      tunnel: w1264 -> [_ w1836]
      tunnel: [w1817 w1835] -> w1263
      tunnel: w1261 -> [_ w1834]
      tunnel: w1257 -> [w1824 w1833]
      tunnel: w1256 -> [w1823 w1832]
      tunnel: [w1824 w1831] -> w1255
      tunnel: [w1823 w1830] -> w1254
      tunnel: w1253 -> [w1822 w1829]
      tunnel: [w1822 w1828] -> w1252
      frame False {
        w1820 = FALSE
        # "Recovery Mode COunt"
        # "Frames Processed - L"
        # "Recovery Search move Count - L"
        # "Recovery Search Attempt Count- L"
        # "WAITING FOR NEW IMAGE, RETAIN ALL VALUES"
      }
      frame True {
        w1866 = u16 1023
        w1869 = u16 0
        # "New Tracking State"
        # "Tracking Timeout Count"
        # "Next Main State"
        # "Next Recovery State"
        # "Reset Respond"
        # "Search Direction"
        # "Recovery Count"
        # "Recovery Search move Count"
        # "Recovery Search Attempt Count"
        # "Frames Processed"
        # "Apply Floor/Ceiling to Goal Position"
        # "Current move Delta"
        # "Service Track Angle Flag"
        # "Move Servo"
        # "Goal Position"
        # "Go to Current State"
        n702 = case shown="\"Recovery Mode\"" w1862 {
          tunnel: w1858 -> [w1888 w1965 w2143]
          tunnel: w1859 -> [_ w1967 _]
          tunnel: w1844 -> [w1887 _ w2138]
          tunnel: w1856 -> [w1886 w1947 w2132]
          tunnel: [w1885 w1963 w2142] -> w1870
          tunnel: [w1883 w1964 w2141] -> w1863
          tunnel: w1860 -> [w1881 w1958 w2119]
          tunnel: [w1880 w1960 w2128] -> w1842
          tunnel: w1861 -> [w1879 w1959 w2118]
          tunnel: w1857 -> [_ w1968 w2139]
          tunnel: w1846 -> [_ w1966 _]
          tunnel: [w1873 w1962 w2123] -> w1843
          tunnel: w1845 -> [_ w1961 _]
          tunnel: w1854 -> [w1878 _ w2133]
          tunnel: [enum16{"Generic Sweep", "Recovery Search"}."Recovery Search" enum16{"Generic Sweep", "Recovery Search"}."Recovery Search" w2140] -> w1828
          tunnel: w1849 -> [_ _ w2137]
          tunnel: w1829 -> [_ _ w2120]
          tunnel: w1855 -> [_ w1944 w2149]
          tunnel: w1836 -> [_ w1949 w2144]
          tunnel: w1851 -> [_ w1951 w2146]
          tunnel: w1852 -> [_ w1952 w2147]
          tunnel: w1853 -> [_ w1953 w2148]
          tunnel: w1850 -> [_ w1950 w2145]
          tunnel: [FALSE w1946 w2121] -> w1841
          tunnel: w1834 -> [w1877 _ w2131]
          tunnel: [w1873 w1941 w2130] -> w1837
          tunnel: [w1873 w1941 w2136] -> w1840
          tunnel: [w1873 w1941 w2135] -> w1839
          tunnel: [w1876 w1942 w2134] -> w1838
          tunnel: w1848 -> [_ _ w2126]
          tunnel: w1847 -> [_ _ w2125]
          tunnel: [w1874 w1947 w2124] -> w1835
          tunnel: w1833 -> [_ w1957 _]
          tunnel: [w1873 w1948 w2123] -> w1831
          tunnel: w1832 -> [_ w1954 _]
          tunnel: [enum16{"Track", "Reactive Predict", ""}."Track" ("Initial Tracking State - Right") w1945 enum16{"Track", "Reactive Predict", ""}."Track" ("Initial Tracking State - Right")] -> w1830
          frame "Start Up Search", Default {
            w1873 = u16 0
            # "Search Direction"
            # "Wait for 'x' Images to be Processed\nBefore Going to Next Step"
            # "Next Main State"
            # "New Goal Position"
            # "Move Servo"
            # "Choose Next State"
            # "Frames Processed Count"
            n703 = Greater Or Equal?(x=w1878, y=w1877) -> (x >= y?=w1884:bool)
            n704 = case shown="True" w1884 {
              tunnel: w1888 -> [w1903 w1915]
              tunnel: w1887 -> [_ w1913]
              tunnel: w1886 -> [w1902 w1912]
              tunnel: [w1903 w1909] -> w1885
              tunnel: [w1901 0] -> w1876
              tunnel: [FALSE TRUE] -> w1882
              tunnel: w1878 -> [w1904 _]
              tunnel: [w1902 w1906] -> w1874
              frame False {
                # "Increase Frames\nProcessed Count"
                n705 = Increment(x=w1904) -> (x+1=w1901:i32)
              }
              frame True {
                # "Reset Frames\nProcessed Count"
                # "SWEEP SEARCH - Startup"
                # "Multiple New Step\nby Step SIze"
                # "F = CCW\nT = CW"
                # "Last Direction"
                # "Min Step"
                # "add 10 in case\nactual position\nis lower than GP"
                # "Set New Step #"
                # "Choose Direction"
                # "Nearest step"
                # "Adjust Actual Posiiton\n to pre-determiend steps"
                # "Move Servo 1 \"Step\" to\nSearch"
                n706 = Add(x=3, y=w1915) -> (x+y=w1921:i32)
                n707 = Quotient & Remainder(x=w1921, y=w1913) -> (floor(x/y)=w1919:i32)  [unwired: 1 out]
                n708 = To Byte Integer(number=w1919) -> (8bit integer=w1910:i8)
                n709 = Less?(x=w1910, y=1) -> (x < y?=w1916:bool)
                n710 = case shown="False" w1916 {
                  tunnel: w1910 -> [w1932 w1940]
                  tunnel: [w1934 FALSE] -> w1906
                  tunnel: [w1933 w1940] -> w1918
                  tunnel: w1912 -> [w1931 _]
                  tunnel: w1913 -> [w1929 _]
                  frame False {
                    # "Max Step"
                    # "# of steps\nminus 1"
                    n711 = Divide(x=1024, y=w1929) -> (x/y=w1926:dbl)
                    n712 = To Unsigned Byte Integer(number=w1926) -> (unsigned 8bit integer=w1927:u8)
                    n713 = Greater Or Equal?(x=w1932, y=w1927) -> (x >= y?=w1928:bool)
                    n714 = case shown="True" w1928 {
                      tunnel: [w1935 TRUE] -> w1934
                      tunnel: [w1936 w1937] -> w1933
                      tunnel: w1932 -> [w1936 w1937]
                      tunnel: w1931 -> [w1935 _]
                      frame False {
                        # "No Need to\nChange Direction"
                      }
                      frame True {
                        # "T"
                        # "Move CW"
                      }
                    }
                  }
                  frame True {
                    # "F"
                    # "Move CCW"
                  }
                }
                n715 = case shown="False" w1906 {
                  tunnel: w1918 -> [w1923 w1924]
                  tunnel: [w1922 w1925] -> w1914
                  frame False {
                    # "CCW\n+1"
                    n716 = Increment(x=w1923) -> (x+1=w1922:i8)
                  }
                  frame True {
                    # "CW\n-1"
                    n717 = Decrement(x=w1924) -> (x-1=w1925:i8)
                  }
                }
                n718 = Multiply(x=w1914, y=w1913) -> (x*y=w1911:u16)
                n719 = To Unsigned Word Integer(number=w1911) -> (unsigned 16bit integer=w1909:u16)
              }
            }
            n720 = case shown="False" w1881 {
              tunnel: [w1892 FALSE] -> w1883
              tunnel: w1882 -> [w1892 _]
              tunnel: [w1893 w1898] -> w1880
              tunnel: w1879 -> [_ w1896]
              frame False {
                # "Check other Servo\nStay in Startup  State"
                n721 = local read "Track Angle Valid  - R"() -> (w1889:bool)
                n722 = local read "Image Lock - Right"() -> (w1890:bool)
                n723 = Or(x=w1889, y=w1890) -> (x .or. y?=w1891:bool)
                n724 = case shown="True" w1891 {
                  tunnel: [T1."Start Up Search" ("Next Main State") T1."Recovery Mode" ("Next Main State")] -> w1893
                  frame False {
                  }
                  frame True {
                  }
                }
              }
              frame True {
                # "Override Move Servo\nCommand bc an Angle Was Found\nduring this Step"
                # "Transition to Tracking State When\nImage Processing has Locked"
                n725 = case shown="False" w1896 {
                  tunnel: [T1."Start Up Search" ("Next Main State") T1."Tracking" ("Next Main State")] -> w1898
                  frame False {
                  }
                  frame True {
                  }
                }
              }
            }
          }
          frame "Tracking" {
            w1941 = 0
            # "Frames Processed Count"
            # "Image Lock - L"
            # "Track Angle Valid"
            # "Tracking Angle"
            # "Tracking Timeout Count"
            # "Max ove delta"
            # "Move delta threshold"
            # "mount offset"
            # "Current Position"
            # "Move Respond"
            # "Trackin Timeout count"
            # "Move Servo"
            # "delta"
            # "GP"
            # "Reset Move Respond"
            # "New Tracking State"
            # "Delta Move Sum"
            # "Choose Next State"
            n726 = case shown="\"Track\", Default" w1954 {
              tunnel: w1968 -> [w1986 _]
              tunnel: w1967 -> [w1985 _]
              tunnel: w1966 -> [w1984 _]
              tunnel: w1965 -> [w1983 w2041]
              tunnel: [w1982 w2039] -> w1964
              tunnel: [w1981 w2047] -> w1963
              tunnel: [w1980 0] -> w1962
              tunnel: w1961 -> [w1979 _]
              tunnel: w1959 -> [w1978 w2031]
              tunnel: w1958 -> [w1977 w2034]
              tunnel: w1957 -> [w1976 w2036]
              tunnel: w1953 -> [_ w2046]
              tunnel: w1952 -> [_ w2045]
              tunnel: w1951 -> [_ w2044]
              tunnel: w1950 -> [_ w2043]
              tunnel: w1944 -> [_ w2042]
              tunnel: w1949 -> [_ w2040]
              tunnel: [TRUE w2037] -> w1946
              tunnel: [w1973 w2035] -> w1948
              tunnel: [w1971 w2033] -> w1945
              tunnel: [0 0] -> w1942
              frame "Track", Default {
                # "Reset"
                # "Tracking Timeout"
                # "Move Delta"
                # "Goal Position"
                # "Tracking Move"
                # "Move Servo"
                # "Only Consider Tracking Angle\n\nIF\n\nImage Locked        == T\nTrack Angle Flag   == T"
                n727 = And(x=w1978, y=w1977) -> (x .and. y?=w1970:bool)
                n728 = case shown="True" w1970 {
                  tunnel: w1986 -> [_ w1992]
                  tunnel: w1985 -> [_ w2010]
                  tunnel: w1984 -> [_ w2007]
                  tunnel: w1983 -> [w1989 w1997]
                  tunnel: [w1989 w2006] -> w1981
                  tunnel: [w1991 w2005] -> w1982
                  tunnel: [w1991 w2004] -> _
                  tunnel: [u16 0 w2003] -> w1980
                  tunnel: w1979 -> [_ w1999]
                  tunnel: w1976 -> [w1988 _]
                  tunnel: [w1987 0] -> w1973
                  frame False {
                    w1991 = FALSE
                    # "Increment timeout"
                    n729 = Increment(x=w1988) -> (x+1=w1987:i32)
                  }
                  frame True {
                    # "Convert Track Angle to UINT16"
                    # "1024/300"
                    # "Move to Tracking Angle \n\nif delta is greater than move servo threshold\nAND less than max move threshold"
                    n730 = Add(x=w2010, y=w1992) -> (x+y=w2013:sgl)
                    n731 = Add(x=w2013, y=sgl 60.0) -> (x+y=w2012:sgl)
                    n732 = Multiply(x=3.413333333333333, y=w2012) -> (x*y=w1993:dbl)
                    n733 = To Word Integer(number=w1997) -> (16bit integer=w1995:i16)
                    n734 = To Unsigned Word Integer(number=w1993) -> (unsigned 16bit integer=w2009:u16)
                    n735 = To Word Integer(number=w1993) -> (16bit integer=w2008:i16)
                    n736 = Subtract(x=w2008, y=w1995) -> (x-y=w1998:i16)
                    n737 = Absolute Value(x=w1998) -> (abs(x)=w1994:i16)
                    n738 = Greater Or Equal?(x=w1994, y=w2007) -> (x >= y?=w2001:bool)
                    n739 = Less Or Equal?(x=w1994, y=w1999) -> (x <= y?=w2000:bool)
                    n740 = And(x=w2001, y=w2000) -> (x .and. y?=w2002:bool)
                    n741 = case shown="True" w2002 {
                      tunnel: w2009 -> [_ w2021]
                      tunnel: [w2016 w2021] -> w2006
                      tunnel: [w2017 w2027] -> w2005
                      tunnel: [w2017 w2027] -> w2004
                      tunnel: w1997 -> [w2016 _]
                      tunnel: w1994 -> [_ w2026]
                      tunnel: [u16 0 w2026] -> w2003
                      tunnel: w1992 -> [_ w2020]
                      frame False {
                        w2017 = FALSE
                        # "Don't Move"
                      }
                      frame True {
                        w2027 = TRUE
                        # "45 DEG MOUNT OFFSET"
                        # "1024/300"
                        # "Current Delta"
                        # "Use new Track Angle"
                        n742 = Divide(x=w2021, y=3.413333333333333) -> (x/y=w2023:dbl)
                        n743 = Negate(x=w2020) -> (-x=w2019:sgl)
                        n744 = Subtract(x=w2023, y=sgl 60.0) -> (x-y=w2025:dbl)
                        n745 = Add(x=w2025, y=w2019) -> (x+y=w2018:dbl)
                        n746 = local write "Last Track Angle - L"(w2018) -> ()
                      }
                    }
                  }
                }
                n747 = local read "Timeout to \nEnable Reactive Predict"() -> (w1974:u16)
                n748 = Less?(x=w1973, y=w1974) -> (x < y?=w1972:bool)
                n749 = case shown="True" w1972 {
                  tunnel: [enum16{"Track", "Reactive Predict", ""}."Reactive Predict" ("Initial Tracking State - Right") enum16{"Track", "Reactive Predict", ""}."Track" ("Initial Tracking State - Right")] -> w1971
                  frame False {
                  }
                  frame True {
                  }
                }
              }
              frame "Reactive Predict" {
                # "Choose New\nTracking State"
                n750 = Or(x=w2031, y=w2034) -> (x .or. y?=w2030:bool)
                n751 = case shown="False" w2030 {
                  tunnel: [w2060 w2112] -> w2047
                  tunnel: w2046 -> [w2059 _]
                  tunnel: w2045 -> [w2058 _]
                  tunnel: w2044 -> [w2057 _]
                  tunnel: w2043 -> [w2056 _]
                  tunnel: w2042 -> [w2055 _]
                  tunnel: w2040 -> [w2054 _]
                  tunnel: [w2053 w2111] -> w2039
                  tunnel: [w2052 w2111] -> w2037
                  tunnel: w2036 -> [w2051 _]
                  tunnel: [w2050 0] -> w2035
                  tunnel: [enum16{"Track", "Reactive Predict", ""}."Reactive Predict" ("Initial Tracking State - Right") enum16{"Track", "Reactive Predict", ""}."Track" ("Initial Tracking State - Right")] -> w2033
                  tunnel: w2041 -> [w2048 w2112]
                  frame False {
                    # "Stay in Reactive State"
                    # "Increment Track Timeout"
                    # "Move Respond Flag"
                    n752 = Increment(x=w2051) -> (x+1=w2050:i32)
                    n753 = case shown="True" w2055 {
                      tunnel: w2059 -> [_ w2075]
                      tunnel: w2058 -> [_ w2074]
                      tunnel: w2057 -> [_ w2073]
                      tunnel: w2056 -> [_ w2072]
                      tunnel: w2054 -> [_ w2069]
                      tunnel: [w2061 w2065] -> w2060
                      tunnel: [w2062 w2064] -> w2053
                      tunnel: [w2062 w2064] -> w2052
                      tunnel: w2048 -> [w2061 w2063]
                      frame False {
                        w2062 = FALSE
                        # "Reset Move Respond = F"
                        # "Move Servo = F"
                      }
                      frame True {
                        w2064 = TRUE
                        # "Position Lock"
                        # "Current Servo\nPosition"
                        # "Reset Move\nRespond = T"
                        # "Move Servo = T"
                        # "Apply Direction \nto Offset (delta sum)"
                        # "Check Last Known Position of Robot"
                        n754 = case shown="True" w2075 {
                          tunnel: w2074 -> [_ w2103]
                          tunnel: w2073 -> [_ w2078]
                          tunnel: w2072 -> [_ w2079]
                          tunnel: [sgl 1.0 ("y") w2077] -> w2071
                          frame False {
                            # "No Position Data Available"
                            # "Default is to move\nSame Direction as other\nServo"
                          }
                          frame True {
                            w2084 = sgl 1.0 ("y")
                            # "Use previous position/orientation to Guess Which Direction to Move Servo"
                            # "Choose Search Direction"
                            # "\"Perpendicular \nThreshold\""
                            # "If Orientation is\n ~Perpendicular -> Start Search\n in Opposite Direction of Other"
                            # "****add 90 until orientation angle is fixed"
                            # "Last Orientation"
                            # "Convert to Rad"
                            # "Avoid Divide by 0"
                            # "-1/m"
                            # "Calculate Normal Line to \nLast Robot Position\nfrom Center Beacon"
                            # "last Position \nCoordinates"
                            n755 = Unbundle(w2103) -> ("X"=w2083:sgl, "Y"=w2082:sgl)
                            n756 = Unbundle(w2079) -> ("X"=w2081:sgl, "Y"=w2080:sgl)
                            n757 = Subtract(x=w2082, y=w2080) -> (x-y=w2099:sgl)
                            n758 = Subtract(x=w2083, y=w2081) -> (x-y=w2097:sgl)
                            n759 = Equal To 0?(x=w2097) -> (x = 0?=w2098:bool)
                            n760 = case shown="False" w2098 {
                              tunnel: w2099 -> [w2106 _]
                              tunnel: w2097 -> [w2105 _]
                              tunnel: [w2104 1000000000000000.0] -> w2096
                              frame False {
                                n761 = Divide(x=w2106, y=w2105) -> (x/y=w2104:sgl)
                              }
                              frame True {
                              }
                            }
                            n762 = Equal To 0?(x=w2096) -> (x = 0?=w2101:bool)
                            n763 = case shown="False" w2101 {
                              tunnel: [w2108 1e-08] -> w2100
                              tunnel: w2096 -> [w2108 _]
                              frame False {
                              }
                              frame True {
                                # "Can't have infinit slope"
                              }
                            }
                            n764 = Divide(x=-1.0, y=w2100) -> (x/y=w2095:dbl)
                            n765 = Inverse Tangent(1:w2095) -> (0:w2093:dbl)
                            n766 = expression code="(x/pi)*180.0" "radians to degrees"(w2093) -> (w2094:dbl)
                            n767 = To Single Precision Float(number=w2094) -> (single precision float=w2091:sgl)
                            n768 = Add(x=w2078, y=sgl 90.0) -> (x+y=w2090:sgl)
                            n769 = Subtract(x=w2091, y=w2090) -> (x-y=w2089:sgl)
                            n770 = Absolute Value(x=w2089) -> (abs(x)=w2088:sgl)
                            n771 = Less Or Equal?(x=w2088, y=sgl 10.0) -> (x <= y?=w2086:bool)
                            n772 = Negate(x=w2084) -> (-x=w2085:sgl)
                            n773 = Select(t=w2085, s=w2086, f=w2084) -> (s? t:f=w2077:sgl)
                          }
                        }
                        n774 = To Word Integer(number=w2071) -> (16bit integer=w2070:i16)
                        n775 = Multiply(x=w2070, y=w2069) -> (x*y=w2068:i32)
                        n776 = To Word Integer(number=w2063) -> (16bit integer=w2067:i16)
                        n777 = Add(x=w2068, y=w2067) -> (x+y=w2066:i32)
                        n778 = To Unsigned Word Integer(number=w2066) -> (unsigned 16bit integer=w2065:u16)
                      }
                    }
                  }
                  frame True {
                    w2111 = TRUE
                    # "Go Directly to Track State"
                  }
                }
              }
            }
            n779 = local read "Tracking Timeout\nThreshold"() -> (w1955:i32)
            n780 = Less?(x=w1948, y=w1955) -> (x < y?=w1956:bool)
            n781 = case shown="False" w1956 {
              tunnel: [T1."Recovery Mode" ("Next Main State") T1."Tracking" ("Next Main State")] -> w1960
              frame False {
              }
              frame True {
              }
            }
          }
          frame "Recovery Mode" {
            w2123 = u16 0
            # "***Compltetly resets as of R17, used to just reset to \"Max Recovery Count - 1\""
            # "Increment Recoveyr Mode Count"
            # "Frames Processed"
            # "Choose Next Main State"
            # "Reset recovery count"
            # "Recovery move\nCount"
            # "Recovery Search\nAttempt count"
            # "Move Servo = T"
            # "delta move sum"
            # "Robot Position Valid"
            n782 = local read "Image Lock - Right"() -> (w2127:bool)
            n783 = Or(x=w2118, y=w2119) -> (x .or. y?=w2117:bool)
            n784 = case shown="\"Generic Sweep\"" w2120 {
              tunnel: w2149 -> [_ _]
              tunnel: w2148 -> [_ _]
              tunnel: w2147 -> [_ _]
              tunnel: w2146 -> [_ _]
              tunnel: w2145 -> [_ _]
              tunnel: w2144 -> [_ _]
              tunnel: w2143 -> [w2177 w2263]
              tunnel: [w2169 w2261] -> w2142
              tunnel: [w2166 w2255] -> w2141
              tunnel: [FALSE FALSE] -> w2121
              tunnel: [w2171 w2252] -> w2140
              tunnel: w2137 -> [w2175 _]
              tunnel: w2139 -> [w2178 _]
              tunnel: w2138 -> [w2176 w2258]
              tunnel: [w2168 w2251] -> w2135
              tunnel: [w2167 w2251] -> w2136
              tunnel: w2127 -> [w2165 _]
              tunnel: [w2156 w2262] -> w2134
              tunnel: w2133 -> [w2154 w2246]
              tunnel: w2132 -> [w2159 w2259]
              tunnel: w2131 -> [w2155 w2257]
              tunnel: w2118 -> [_ _]
              tunnel: w2119 -> [_ w2254]
              tunnel: [FALSE w2253] -> w2129
              tunnel: w2126 -> [w2163 _]
              tunnel: w2125 -> [w2162 _]
              tunnel: [w2159 w2250] -> w2124
              frame "Recovery Search" {
                # "Wait for 2 Images to be Processed\nBefore Going to Next Step"
                # "Choose Next Reovery State"
                # "Recovery Search \nAttempt Count"
                # "Move Servo"
                # "Goal Position"
                # "Recovery Search\nmove Count"
                # "Attempt Recovery Search if Other Servo has Valid Angle"
                n785 = local read "Last Track Angle - R"() -> (w2158:sgl)
                n786 = Greater Or Equal?(x=w2154, y=w2155) -> (x >= y?=w2157:bool)
                n787 = case shown="True" w2157 {
                  tunnel: w2178 -> [_ w2198]
                  tunnel: [w2183 w2197] -> w2167
                  tunnel: w2177 -> [w2186 w2196]
                  tunnel: w2176 -> [_ w2195]
                  tunnel: [w2184 w2194] -> w2168
                  tunnel: [w2186 w2193] -> w2169
                  tunnel: [FALSE w2192] -> w2166
                  tunnel: w2163 -> [w2184 w2191]
                  tunnel: w2162 -> [w2183 w2190]
                  tunnel: w2165 -> [_ w2189]
                  tunnel: w2158 -> [_ w2188]
                  tunnel: [w2181 0 ("Frames Processed\nCount - in")] -> w2156
                  tunnel: w2154 -> [w2182 _]
                  frame False {
                    # "Increment Frames Processed"
                    # "WAIT"
                    n788 = Increment(x=w2182) -> (x+1=w2181:i32)
                  }
                  frame True {
                    n789 = case shown="True" w2189 {
                      tunnel: w2188 -> [_ w2211]
                      tunnel: w2191 -> [w2199 w2207]
                      tunnel: w2198 -> [_ w2212]
                      tunnel: [w2202 w2210] -> w2193
                      tunnel: [w2200 w2209] -> w2197
                      tunnel: w2190 -> [w2200 w2208]
                      tunnel: w2196 -> [w2202 w2206]
                      tunnel: w2195 -> [_ w2205]
                      tunnel: [FALSE TRUE] -> w2192
                      tunnel: [w2199 w2203] -> w2194
                      frame False {
                        # "Don't Move bc Other Servo Doesn't Have Image Lock"
                      }
                      frame True {
                        # "Move Servo = T"
                        n790 = Greater Than 0?(x=w2207) -> (x > 0?=w2213:bool)
                        n791 = case shown="True" w2213 {
                          tunnel: w2212 -> [w2220 _]
                          tunnel: w2211 -> [w2214 _]
                          tunnel: [w2219 w2230] -> w2210
                          tunnel: [w2217 w2236] -> w2209
                          tunnel: w2208 -> [w2218 w2236]
                          tunnel: w2207 -> [w2216 w2233]
                          tunnel: [w2215 w2235] -> w2203
                          tunnel: w2206 -> [_ w2231]
                          tunnel: w2205 -> [_ w2228]
                          frame False {
                            # "Increment move count to transition\nto Pan mode"
                            # "Increment Recovery Search Attempt Count"
                            # "1024/300"
                            # "Move Parallel to Other Servo"
                            n792 = Increment(x=w2218) -> (x+1=w2217:i32)
                            n793 = Add(x=w2214, y=w2220) -> (x+y=w2226:sgl)
                            n794 = Add(x=w2226, y=sgl 60.0) -> (x+y=w2225:sgl)
                            n795 = Multiply(x=3.413333333333333, y=w2225) -> (x*y=w2223:dbl)
                            n796 = Add(x=0.5, y=w2223) -> (x+y=w2221:dbl)
                            n797 = To Unsigned Word Integer(number=w2221) -> (unsigned 16bit integer=w2219:u16)
                            n798 = Increment(x=w2216) -> (x+1=w2215:i32)
                          }
                          frame True {
                            # "Apply Direction"
                            # "Step SIze"
                            # "Current Position"
                            # "Attempt to Pan in Steps Towards other Servo"
                            # "Could be same or function of \nregular search step size"
                            # "Max # of Pan\nMoves"
                            # "Pan Towards Other Servo"
                            n799 = Greater Or Equal?(x=w2233, y=u16 20) -> (x >= y?=w2234:bool)
                            n800 = case shown="False" w2234 {
                              tunnel: w2233 -> [w2244 _]
                              tunnel: [w2243 u16 0] -> w2235
                              frame False {
                                # "Increment Pan Count"
                                n801 = Increment(x=w2244) -> (x+1=w2243:i32)
                              }
                              frame True {
                                # "Reset move count"
                              }
                            }
                            n802 = local read "Recovery Search\nDirection - L"() -> (w2229:bool)
                            n803 = case shown="False" w2229 {
                              tunnel: w2231 -> [w2238 w2242]
                              tunnel: w2228 -> [w2239 w2241]
                              tunnel: [w2237 w2240] -> w2230
                              frame False {
                                # "CCW"
                                n804 = Add(x=w2238, y=w2239) -> (x+y=w2237:u16)
                              }
                              frame True {
                                # "CW"
                                n805 = Subtract(x=w2242, y=w2241) -> (x-y=w2240:u16)
                              }
                            }
                          }
                        }
                      }
                    }
                  }
                }
                n806 = local read "Max Recovery Count\n(Recovery Search)"() -> (w2160:u16)
                n807 = local read "Max Recovery\nSearch Attempts"() -> (w2161:u16)
                n808 = Less Or Equal?(x=w2167, y=w2161) -> (x <= y?=w2173:bool)
                n809 = Less Or Equal?(x=w2175, y=w2160) -> (x <= y?=w2174:bool)
                n810 = And(x=w2173, y=w2174) -> (x .and. y?=w2172:bool)
                n811 = case shown="False" w2172 {
                  tunnel: [enum16{"Generic Sweep", "Recovery Search"}."Generic Sweep" enum16{"Generic Sweep", "Recovery Search"}."Recovery Search"] -> w2171
                  frame False {
                  }
                  frame True {
                  }
                }
              }
              frame "Generic Sweep" {
                w2251 = u16 0
                # "Angle Valid?"
                # "Choose Next Recovery State"
                # "Wait for 2 Images to be Processed\nBefore Going to Next Step"
                # "New Goal Position"
                # "Move Servo"
                # "Frames Processed Count"
                n812 = Greater Or Equal?(x=w2246, y=w2257) -> (x >= y?=w2264:bool)
                n813 = case shown="True" w2264 {
                  tunnel: w2263 -> [w2280 w2292]
                  tunnel: w2258 -> [_ w2290]
                  tunnel: w2259 -> [w2279 w2289]
                  tunnel: [w2280 w2286] -> w2261
                  tunnel: [w2278 0] -> w2262
                  tunnel: [FALSE TRUE] -> w2256
                  tunnel: w2246 -> [w2281 _]
                  tunnel: [w2279 w2283] -> w2250
                  frame False {
                    # "Increment Frames Processed"
                    n814 = Increment(x=w2281) -> (x+1=w2278:i32)
                  }
                  frame True {
                    # "Reset Frames\nProcessed Count"
                    # "SWEEP SEARCH - Startup"
                    # "Multiple New Step\nby Step SIze"
                    # "F = CCW\nT = CW"
                    # "Last Direction"
                    # "Min Step"
                    # "add 10 in case\nactual position\nis lower than GP"
                    # "Set New Step #"
                    # "Choose Direction"
                    # "Nearest step"
                    # "Adjust Actual Posiiton\n to pre-determiend steps"
                    # "Move Servo 1 \"Step\" to\nSearch"
                    n815 = Add(x=5, y=w2292) -> (x+y=w2298:i32)
                    n816 = Quotient & Remainder(x=w2298, y=w2290) -> (floor(x/y)=w2296:i32)  [unwired: 1 out]
                    n817 = To Byte Integer(number=w2296) -> (8bit integer=w2287:i8)
                    n818 = Less?(x=w2287, y=1) -> (x < y?=w2293:bool)
                    n819 = case shown="False" w2293 {
                      tunnel: w2287 -> [w2309 w2317]
                      tunnel: [w2311 FALSE] -> w2283
                      tunnel: [w2310 w2317] -> w2295
                      tunnel: w2289 -> [w2308 _]
                      tunnel: w2290 -> [w2306 _]
                      frame False {
                        # "Max Step"
                        # "# of steps\nminus 1"
                        n820 = Divide(x=1024, y=w2306) -> (x/y=w2303:dbl)
                        n821 = To Unsigned Byte Integer(number=w2303) -> (unsigned 8bit integer=w2304:u8)
                        n822 = Greater Or Equal?(x=w2309, y=w2304) -> (x >= y?=w2305:bool)
                        n823 = case shown="True" w2305 {
                          tunnel: [w2312 TRUE] -> w2311
                          tunnel: [w2313 w2314] -> w2310
                          tunnel: w2309 -> [w2313 w2314]
                          tunnel: w2308 -> [w2312 _]
                          frame False {
                            # "No Need to\nChange Direction"
                          }
                          frame True {
                            # "T"
                            # "Move CW"
                          }
                        }
                      }
                      frame True {
                        # "F"
                        # "Move CCW"
                      }
                    }
                    n824 = case shown="True" w2283 {
                      tunnel: w2295 -> [w2300 w2301]
                      tunnel: [w2299 w2302] -> w2291
                      frame False {
                        # "CCW\n+1"
                        n825 = Increment(x=w2300) -> (x+1=w2299:i8)
                      }
                      frame True {
                        # "CW\n-1"
                        n826 = Decrement(x=w2301) -> (x-1=w2302:i8)
                      }
                    }
                    n827 = Multiply(x=w2291, y=w2290) -> (x*y=w2288:u16)
                    n828 = To Unsigned Word Integer(number=w2288) -> (unsigned 16bit integer=w2286:u16)
                  }
                }
                n829 = local read "Track Angle Valid  - R"() -> (w2249:bool)
                n830 = local read "Image Lock - Right"() -> (w2248:bool)
                n831 = Or(x=w2248, y=w2249) -> (x .or. y?=w2247:bool)
                n832 = case shown="False" w2254 {
                  tunnel: [w2267 w2277] -> w2255
                  tunnel: w2256 -> [w2268 _]
                  tunnel: [w2269 enum16{"Generic Sweep", "Recovery Search"}."Generic Sweep"] -> w2252
                  tunnel: [w2266 w2277] -> w2253
                  tunnel: w2247 -> [w2265 _]
                  frame False {
                    # "Is other servo tracking?"
                    n833 = case shown="True" w2265 {
                      tunnel: [enum16{"Generic Sweep", "Recovery Search"}."Generic Sweep" enum16{"Generic Sweep", "Recovery Search"}."Recovery Search"] -> w2269
                      tunnel: w2268 -> [w2272 _]
                      tunnel: [w2272 FALSE] -> w2267
                      tunnel: [FALSE TRUE] -> w2266
                      frame False {
                        # "Stay in Sweep"
                      }
                      frame True {
                        # "G o to Recovery Search  State"
                      }
                    }
                  }
                  frame True {
                    w2277 = FALSE
                    # "Override Move Servo\nCommand bc an Angle Was Found\nduring this Step"
                    # "Stay In Sweep\nLet Main State Machine transition\ninto Tracking"
                  }
                }
              }
            }
            n834 = Increment(x=w2137) -> (x+1=w2116:i32)
            n835 = case shown="True" w2129 {
              tunnel: w2116 -> [w2152 _]
              tunnel: [w2152 0] -> w2130
              frame False {
              }
              frame True {
              }
            }
            n836 = case shown="False" w2117 {
              tunnel: [T1."Recovery Mode" ("Next Main State") T1."Tracking" ("Next Main State")] -> w2128
              frame False {
              }
              frame True {
              }
            }
          }
        }
        "Current Move Delta - L" <- w1843
        n837 = Less?(x=w1870, y=w1869) -> (x < y?=w1868:bool)
        n838 = local write "New Data  Flag\nLeft Servo"(FALSE) -> ()
        n839 = Select(t=w1869, s=w1868, f=w1870) -> (s? t:f=w1865:u16)
        n840 = Greater?(x=w1865, y=w1866) -> (0:w1867:bool)
        n841 = Select(t=w1866, s=w1867, f=w1865) -> (s? t:f=w1864:u16)
      }
    }
    "Next Main State - Left" <- w1271
    "Next Tracking State - Left" <- w1254
    "Next Recovery State - Left" <- w1252
    n842 = flat-sequence {
      tunnel: w1297 -> [w2324]
      tunnel: w1224 -> [w2323]
      tunnel: w1298 -> [w2326]
      tunnel: w1213 -> [w2325]
      tunnel: [w2324] -> w1311
      tunnel: [w2323] -> w1310
      tunnel: w1311 -> [w2332]
      tunnel: [w2331] -> w1306
      tunnel: [w2330] -> w1307
      tunnel: w1310 -> [w2329]
      frame #0 {
        # "Only Update GP if Moving Servo"
        n843 = case shown="True" w2324 {
          tunnel: w2326 -> [_ w2328]
          frame False {
          }
          frame True {
            # "Update Goal Position"
            n844 = local write "Servo Goal Position\n - Left"(w2328) -> ()
          }
        }
        n845 = case shown="True" w2323 {
          tunnel: w2325 -> [_ w2327]
          frame False {
          }
          frame True {
            # "New Direction"
            # "Update Goal Position"
            # "Update Direction"
            n846 = local write "Servo Goal Position\n - Right"(w2327) -> ()
          }
        }
      }
      frame #1 {
        # "Allow Comm Process to Take Down the Flag\nOnly Raise if not already in motion"
        n847 = local read "Servo Moving - R"() -> (w2337:bool)
        n848 = local read "Servo Moving - L"() -> (w2334:bool)
        n849 = local read "Move Servo - L"() -> (w2333:bool)
        n850 = local read "Move Servo - R"() -> (w2340:bool)
        n851 = Not(x=w2337) -> (.not. x?=w2339:bool)
        n852 = Not(x=w2334) -> (.not. x?=w2336:bool)
        n853 = And(x=w2329, y=w2339) -> (x .and. y?=w2338:bool)
        n854 = And(x=w2332, y=w2336) -> (x .and. y?=w2335:bool)
        n855 = case shown="True" w2338 {
          selector: w2338 -> [_ w2342]
          tunnel: [w2341 w2342] -> w2330
          tunnel: w2340 -> [w2341 _]
          frame False {
          }
          frame True {
          }
        }
        n856 = case shown="False" w2335 {
          selector: w2335 -> [_ w2344]
          tunnel: [w2343 w2344] -> w2331
          tunnel: w2333 -> [w2343 _]
          frame False {
          }
          frame True {
          }
        }
        n857 = local write "Move Servo - R"(w2330) -> ()
        n858 = local write "Move Servo - L"(w2331) -> ()
      }
    }
    n859 = local read "Current Main State - Right"() -> (w1276:T1)
    n860 = local read "Current Main State - Left"() -> (w1277:T1)
    n861 = Equal?(x=w1277, y=w1275) -> (x = y?=w1274:bool)
    n862 = Equal?(x=w1276, y=w1275) -> (x = y?=w1273:bool)
    n863 = And(x=w1274, y=w1306) -> (x .and. y?=w1302:bool)
    n864 = And(x=w1307, y=w1273) -> (x .and. y?=w1303:bool)
    n865 = And(x=w1274, y=w1273) -> (x .and. y?=w1301:bool)
    n866 = Exclusive Or(1:w1303, 2:w1302) -> (0:w1300:bool)
    n867 = case shown="True" w1300 {
      tunnel: [w2355 w2376] -> w1308
      tunnel: [w2356 w2375] -> w1304
      tunnel: w1223 -> [_ w2379]
      tunnel: w1264 -> [w2353 w2380]
      tunnel: w1227 -> [w2351 w2378]
      tunnel: [w2354 w2366] -> w1305
      tunnel: [w2352 w2365] -> w1309
      tunnel: w1272 -> [_ w2377]
      tunnel: w1301 -> [w2350 _]
      tunnel: w1302 -> [_ w2376]
      tunnel: w1303 -> [_ w2375]
      frame False {
        n868 = case shown="False" w2350 {
          tunnel: [w2360 w2362] -> w2356
          tunnel: [w2359 w2362] -> w2355
          tunnel: [w2358 w2361] -> w2354
          tunnel: w2353 -> [w2358 _]
          tunnel: [w2357 w2361] -> w2352
          tunnel: w2351 -> [w2357 _]
          frame False {
            # "No Movement\nRetain All Values"
            n869 = local read "Move Respond - L"() -> (w2360:bool)
            n870 = local read "Move Respond - R"() -> (w2359:bool)
          }
          frame True {
            w2361 = i16 0
            w2362 = FALSE
            # "Reset Delta Move sum\nfor both"
            # "F"
            # "Both Moved,\nMake Flags False"
          }
        }
      }
      frame True {
        w2372 = 200 ("y")
        w2363 = -200 ("y")
        # "Add/Clear Sum for \nServo That didn't move"
        # "Update Moving Servo's  Delta Position"
        # "if one Servo Moves, other should \nmove too eventually,\nUsed in Search Process"
        # "Only 1 Servo is Moving Due to Tracking --> Update delta move sum"
        n871 = case shown="True" w2375 {
          tunnel: w2380 -> [_ w2388]
          tunnel: w2379 -> [_ w2387]
          tunnel: [i16 0 w2386] -> w2373
          frame False {
          }
          frame True {
            n872 = Add(x=w2388, y=w2387) -> (x+y=w2386:i32)
          }
        }
        n873 = case shown="True" w2376 {
          tunnel: w2378 -> [_ w2384]
          tunnel: w2377 -> [_ w2383]
          tunnel: [i16 0 w2382] -> w2370
          frame False {
          }
          frame True {
            n874 = Add(x=w2384, y=w2383) -> (x+y=w2382:i32)
          }
        }
        n875 = Greater?(x=w2373, y=w2372) -> (0:w2374:bool)
        n876 = Greater?(x=w2370, y=w2372) -> (0:w2371:bool)
        n877 = Select(t=w2372, s=w2371, f=w2370) -> (s? t:f=w2367:i32)
        n878 = Select(t=w2372, s=w2374, f=w2373) -> (s? t:f=w2368:i32)
        n879 = Greater?(x=w2368, y=w2363) -> (0:w2364:bool)
        n880 = Greater?(x=w2367, y=w2363) -> (0:w2369:bool)
        n881 = Select(t=w2367, s=w2369, f=w2363) -> (s? t:f=w2365:i32)
        n882 = Select(t=w2368, s=w2364, f=w2363) -> (s? t:f=w2366:i32)
      }
    }
    n883 = case shown="True" w1219 {
      selector: w1219 -> [_ w2322]
      tunnel: [w2319 w2321] -> w1259
      tunnel: [w2318 i16 0] -> w1260
      tunnel: w1308 -> [w2319 _]
      tunnel: w1309 -> [w2318 _]
      frame False {
      }
      frame True {
        n884 = Not(x=w2322) -> (.not. x?=w2321:bool)
      }
    }
    "Move Respond - R" <- w1259
    "deltaMoveServo\n- R" <- w1260
    n885 = case shown="False" w1270 {
      selector: w1270 -> [_ w2349]
      tunnel: [w2346 w2348] -> w1262
      tunnel: [w2345 i16 0] -> w1265
      tunnel: w1304 -> [w2346 _]
      tunnel: w1305 -> [w2345 _]
      frame False {
      }
      frame True {
        n886 = Not(x=w2349) -> (.not. x?=w2348:bool)
      }
    }
    "Move Respond - L" <- w1262
    "deltaMoveServo\n- L" <- w1265
    "Current Main State - Left" <- w1296
    "Frames Processed\nCount - in -L" <- w1288
    "Recovery Mode Count - in Left" <- w1283
    "Recovery Search\nmove Count - in - L" <- w1282
    "Recovery Search\nAttempt Count - in - L" <- w1281
    "Current Main State - Right" <- w1250
    "Frames Processed\nCount - in Right" <- w1233
    "Recovery Search\nmove Count - Right" <- w1235
    "Recovery Search\nAttempt Count - Right" <- w1234
    "Recovery Mode Count in Right" <- w1226
    "Tracking Timeout\nCount - L" <- w1257
    "Tracking Timeout\nCount - R" <- w1242
    "Current Tracking State - Left" <- w1256
    "Current Tracking State - Right 2" <- w1248
    "Current Recovery State - Right" <- w1249
    "Current Recovery State -L" <- w1253
  }
